vi "UHR-Fleezers Control (host) - 9.0.vi"() -> ()   [LabVIEW 2009]
uses:
  <vilib>/Utility/miscctls.llb/LVPoint32TypeDef.ctl
  <vilib>/Utility/miscctls.llb/LVMinMaxIncTypeDef.ctl
  <vilib>/userDefined/High Color/nirio_resource_hc.ctl
  <vilib>/Instr/_visa.llb/VISA Configure Serial Port (Instr).vi
  <vilib>/rvi/interface/nirviOpenFPGA/nirviOpenFPGA.xnode
  FPGA Bitfiles/UHR-Fleezers Instr~3C_FPGA Target_UHR-Fleezers Contr~F0.lvbitx
  UHR-Fleezers Control (fpga) - 9.1.vi
  <vilib>/FPGAPlugInAG/PCIe-7852R/nirviIntfOpen_PCIe-7852R.vi
  <vilib>/rvi/interface/nirviMethod/nirviMethod.xnode
  <vilib>/Utility/error.llb/Merge Errors.vi
  <vilib>/LabVIEW Targets/FPGA/Rio/nirio_HostInterface/nirio_Reset.vi
  <vilib>/LabVIEW Targets/FPGA/Rio/nirio_HostInterface/nirio_DMAStopAll.vi
  <vilib>/rvi/interface/common/niFpgaNodeNameForErrorReporting.ctl
  <vilib>/rvi/errors/niLvFpgaWhatHappensToTopLevelVI.ctl
  <vilib>/LabVIEW Targets/FPGA/Rio/nirio_HostInterface/nirio_DisableInterrupts.vi
  <vilib>/Utility/error.llb/Error Cluster From Error Code.vi
  <vilib>/rvi/errors/niLvFpgaAdjustHostInterfaceError.vi
  <vilib>/rvi/interface/nirviReadWriteControl/nirviReadWriteControl.xnode
  <vilib>/LabVIEW Targets/FPGA/Rio/nirio_HostInterface/nirio_WriteBig.vi
  <vilib>/LabVIEW Targets/FPGA/Rio/nirio_HostInterface/nirio_DMAConfigure.vi
  <vilib>/LabVIEW Targets/FPGA/Rio/nirio_HostInterface/nirio_DMAStop.vi
  <vilib>/RVI Host/nirviSupport.llb/nirviErrorClusterFromErrorCode.vi
  <vilib>/LabVIEW Targets/FPGA/Rio/nirio_HostInterface/nirio_EnableInterrupts.vi
  <vilib>/rvi/errors/niLvFpgaReportInternalErrorWithAdditionalInfo.vi
  <vilib>/Platform/TimedLoop/XDataNode/XDataNode.xnode
  <vilib>/Platform/TimedLoop/XDataNode/loadlvalarms.vi
  <vilib>/Platform/TimedLoop/XDataNode/timing_clust.ctl
  <vilib>/Platform/TimedLoop/XDataNode/nitl_modes.ctl
  <vilib>/Platform/TimedLoop/XDataNode/wakeup.ctl
  <vilib>/express/express analysis/Spectral/XNode/ExpressSpectralMeasurementsBlockNode.xnode
  <vilib>/express/express analysis/Spectral/Block/exnSpectralBlock spectral measurements PSD poly.vi
  <vilib>/express/express analysis/Spectral/Block/exnSpectralBlock spectral measurements PSD WFM.vi
  <vilib>/Waveform/WDTOps.llb/WDT Append Waveforms DBL.vi
  <vilib>/LabVIEW Targets/FPGA/Rio/nirio_HostInterface/nirio_ReadBig.vi
  <vilib>/vision/Avi1.llb/AviRefnum.ctl
  <vilib>/rvi/interface/nirviCloseFPGA/nirviCloseFPGA.xnode
  <vilib>/FPGAPlugInAG/PCIe-7852R/nirviIntfClose_PCIe-7852R.vi
  <vilib>/Analysis/NI_AALBase.lvlib
  <vilib>/Platform/TimedLoop/XDataNode/XDNodeRunTimeDep.lvlib
  openfpgaref.8.6.ctl
  NiRioSrv.dll
  <vilib>/vision/NI_Vision_Development_Module.lvlib
panel:
  in  "Set Confocal Spot":bool
  out "X (V)":dbl format="%_3g"
  out "Y (V)":dbl format="%_3g"
  in  "Tab Control 8":enum32{"APD 1 Image", "APD 1 Line Scan"}(tab)
  out "APD 1b":T1(plugin-control)
  out "Waveform Graph":dbl[](graph)
  in  "Total Volume\nFlushed (uL)":dbl
  in  "Flush Center Channel":bool
  in  "Inject Bottom Channel":bool
  in  "Inject Top Channel":bool
  out "Messages":string
  in  "APD Ave N":dbl=10.0
  out "Int. Time (s)":dbl
  in  "Stop All":bool
  out "sigma/mean":dbl
  out "Rate sigma (Hz)":dbl format="%0.2f"
  out "Current Stage  Position":cluster{dbl, dbl, dbl}
  in  "Index":dbl=1.0 caption="Save File Index" min=1.0 step=1.0
  in  "Tab Control 6":T2(tab)=enum."Dual Display (APD)"
  out "All Signals":waveform(dbl)[](graph)
  in  "Signals to Plot":i32(listbox)
  out "Trap Disp. Freq. (Hz)":dbl caption="Freq. (Hz)" format="%#_6p"
  out "Display Period (s)":dbl caption="Period (s)" format="%#_6p"
  in  "Trap Disp. Downsample":dbl=20000.0 caption="Downsample"
  in  "APD Disp. Scale":dbl=0.1 caption="Scale (Divide,\nfor above plot only)"
  in  "APD Disp. Downsample":dbl=30.0 caption="Integrate" min=1.0 step=1.0
  out "APD Display Freq. (Hz)":dbl caption="Freq. (Hz)"
  out "APD Display Period (s)":dbl caption="Period (s)"
  out "RMS (Ang)":dbl format="%_2g"
  in  "Bead Sep. Int. Time (s)":dbl=5.0 caption="Int. Time (s)"
  in  "Below (kHz)":dbl=0.5
  in  "Above (kHz)":dbl=2.0
  in  "Adjust Scale\nto Mean":bool
  in  "Rescale on Mean":bool
  in  "Offset (nm)":dbl
  out "Mean":dbl caption="Mean (pN)" format="%#_3g"
  out "Force":waveform(dbl)[](graph)
  out "APD 1 Chart":waveform(dbl)(graph)
  in  "Calibration":u16(ring)=2 items=["None", "Position", "Force"]
  out "T1 X":dbl caption="T1 X (pN)" format="%0.2f"
  out "T2 X":dbl caption="T2 X (pN)" format="%0.2f"
  out "Bead Separation":waveform(dbl)(graph)
  in  "Amplitude (nm)":dbl=1.0
  out "Bead Mean (nm)":dbl caption="Mean (nm)" format="%0.2f"
  out "Difference":dbl caption="Difference (pN)" format="%.2g"
  out "FFT 1":cluster{"f0":dbl, "df":dbl, "magnitude":dbl[]}[](graph)
  out "FFT 2":cluster{"f0":dbl, "df":dbl, "magnitude":dbl[]}[](graph)
  in  "FFT 1 Choice 1":u16(ring) items=["T1 Y", "T1 X", "T1 Sum", "T2 Y", "T2 X", "T2 Sum", "T1 FB X", "T1 FB Sum", "T2 FB X", "T2 FB Sum", "PSD Y", "PSD X", "PSD Y Sum", "none"]
  in  "FFT 2 Choice 1":u16(ring)=13 items=["T1 Y", "T1 X", "T1 Sum", "T2 Y", "T2 X", "T2 Sum", "T1 FB X", "T1 FB Sum", "T2 FB X", "T2 FB Sum", "PSD Y", "PSD X", "PSD Y Sum", "none"]
  in  "FFT 1 Choice 2":u16(ring)=1 items=["T1 Y", "T1 X", "T1 Sum", "T2 Y", "T2 X", "T2 Sum", "T1 FB X", "T1 FB Sum", "T2 FB X", "T2 FB Sum", "PSD Y", "PSD X", "PSD Y Sum", "none"]
  in  "FFT 2 Choice 2":u16(ring)=13 items=["T1 Y", "T1 X", "T1 Sum", "T2 Y", "T2 X", "T2 Sum", "T1 FB X", "T1 FB Sum", "T2 FB X", "T2 FB Sum", "PSD Y", "PSD X", "PSD Y Sum", "none"]
  in  "Compute FFT":bool
  in  "Reset FFT":bool
  in  "# Spectra to Ave.":dbl=100.0
  out "Ave. Time (s)":dbl
  out "1 Channel":waveform(dbl)(graph)
  out "Slow mean":dbl format="%0.2f"
  in  "Slow mean N ave.":dbl=1.0 min=1.0 step=1.0
  out "Mean Intensity":dbl
  out "Sigma":dbl
  out "Sigma/Mean":dbl
  in  "Subtract mean":bool
  in  "High Res. Display":u16(ring) items=["T1 Y", "T1 X", "T1 Sum", "T2 Y", "T2 X", "T2 Sum", "T1 FB X", "T1 FB Sum", "T2 FB X", "T2 FB Sum", "PSD Y", "PSD X", "PSD Y Sum"]
  out "APD 1 Rate (Hz)":dbl format="%#_3p"
  out "Image":u32[][](graph)
  in  "Tab Control":T3(tab)
  in  "Read Cal":bool
  out "Tether":bool
  in  "Tether Alarm?":bool=TRUE
  in  "Move to Delta (MHz)":dbl=15.6
  in  "Then...":string(combo)="2"
  in  "Data Acq. Spot":bool
  out "Fl. High":bool
  out "Waiting":bool
  in  "Yank to Freq. (MHz)":dbl
  in  "Fl. Threshold (kHz)":dbl
  in  "Fl. Triggered...":bool
  in  "Confocal Linescan":bool
  in  "Speed (nm/s)":dbl=100.0
  in  "Stop F (pN)":dbl=4.0
  in  "Furthest Withdraw (MHz)":dbl=15.0
  in  "Closest Delta (MHz)":dbl=10.0 step=0.25
  in  "Fish for Tether":bool
  in  "Confocal Image":bool
  in  "Round T1 X":bool caption="Round"
  in  "T1 offset_x (mV)":dbl=-26.302542012392074 format="%#_2g"
  in  "T1 kappa_x (pN/nm)":dbl=0.22546432407642192 min=0.0 step=0.001 format="%#_2g"
  out "Time (s)":dbl
  out "Total Time (s)":dbl
  in  "Start Saving":bool
  in  "Limits Enable":bool=TRUE caption="Enable"
  in  "Limit Max (MHz)":dbl=16.0 caption="Max (MHz)"
  in  "Limit Min (MHz)":dbl=10.0 caption="Min (MHz)"
  in  "Cal sets to save":u32=100 min=1 step=1
  in  "Comment (data description)":string="testing confocal setup"
  out "Calibrating Trap...":bool
  in  "Trap 2 (ON/OFF)":bool
  in  "Trap 1 (ON/OFF)":bool
  in  "Save Calibration":bool
  in  "N sets to save":u32=200 caption="N Sets"
  in  "Save N Sets":bool
  out "Save file name":path
  in  "Save ave N":dbl=500.0 caption="Averaging Factor"
  out "Saving...":bool
  in  "Stop Saving":bool
  out "Progress":u16(slide) scale=0.0..100.0
  out "Manipulating Trap":bool
  out "Buffer Status":dbl(slide) scale=0.0..1.0
  out "Overflow (data lost)":bool
  in  "Reset":bool
  out "Data Rate (Hz)":dbl caption="Trap Data Rate (Hz)" format="%#_3p"
  out "Data Period (s)":dbl caption="Trap Data Period (s)" format="%#_6p"
  out "Save Data Rate (Hz)":dbl caption="Rate (Hz)" format="%#_6p"
  out "Save Data Period (s)":dbl caption="Period (s)" format="%#_6p"
  in  "T1 alpha_x (nm/V)":dbl=630.439304367558 step=10.0 format="%#_3g"
  in  "T2 alpha_x (nm/V)":dbl=704.7738222964198 step=10.0 format="%#_3g"
  in  "T2 kappa_x (pN/nm)":dbl=0.2030110880477556 min=0.0 step=0.001 format="%#_2g"
  in  "T2 offset_x (mV)":dbl=-26.67973517613748 format="%#_2g"
  in  "BD 1 Frequency 1 (MHz)":dbl=69.4 caption="T1 X (MHz)" min=60.0 max=90.0 step=1.0 format="%#_6p"
  in  "BD 1 Frequency 2 (MHz)":dbl=85.0 caption="T2 X (MHz)" min=60.0 max=90.0 step=1.0 format="%#_6p"
  in  "Green Laser ON/Interlacing":bool
  in  "Round T2 X":bool caption="Round"
  in  "AO1":dbl(slide)=5.5955906765028605 caption="Confocal Y (V)" min=0.0 max=10.0 step=0.01 scale=0.0..10.0 scale format="%_1f"
  in  "AO2":dbl(slide)=5.59714185835527 caption="Confocal X (V)" min=0.0 max=10.0 step=0.01 scale=0.0..10.0 scale format="%_1f"
  in  "Upper Cap.":bool
  in  "Lower Cap.":bool
  in  "Trap Raster Scan":bool
  out "Raster Scanning...":bool
  in  "Trap Delta (MHz)":dbl=15.599999999999994
  in  "Action":string(combo)="Alarm"
  in  "Dump Beads":bool
  out "Duration (s)":dbl
  out "Stage Moving":bool
  in  "Wait Before Save (s)":u32=1
  out "Attempts":dbl
  in  "Attempt Limit":dbl=20.0 caption="Limit"
  in  "z nudge increment (um)":dbl=0.5
  in  "+z":bool
  in  "Saved Stage Positions":T4={"Position 1"={1.27817, -0.38076, 0.0}, "Position 2"={0.0, 0.0, 0.0}, "Position 3"={2.04843, -0.2477, 0.0}, "Position 4"={2.04843, 0.60288, 0.0}} {"Position 1"."?" min=-0.1 max=0.1 step=0.1; "Position 2"."?" min=-0.1 max=0.1 step=0.1; "Position 3"."?" min=-0.1 max=0.1 step=0.1; "Position 4"."?" min=-0.1 max=0.1 step=0.1}
  in  "Position 1 Label":string="Upper capillary"
  in  "Set Position 1":bool
  in  "Set Position 2":bool
  in  "Set Position 3":bool
  in  "Set Position 4":bool
  in  "Move to Position 3":bool
  in  "Move to Position 4":bool
  in  "Move to Position 2":bool
  in  "Move to Position 1":bool
  in  "Position 2 Label":string="Lower capillary"
  in  "Position 3 Label":string="Measurement Spot"
  in  "Position 4 Label":string="Dump beads"
  in  "-z":bool
  in  "Top Ch Inject Rate (ul/h)":dbl=10.0
  in  "Pump write delay (ms)":dbl=300.0
  in  "All Pump Parameters":T5={"Pump 1"={"Diameter (mm)"=4.61, "Units"=3.0, "Volume"=0.0, "Rate"=0.0}, "Pump 2"={"Diameter (mm)"=4.61, "Units"=3.0, "Volume"=0.0, "Rate"=0.0}, "Pump 3"={"Diameter (mm)"=4.61, "Units"=3.0, "Volume"=0.0, "Rate"=0.0}}
  in  "Top Ch Inject Volume (uL)":dbl=100.0
  in  "Pump pause delay (ms)":u32
  in  "Bottom Ch Inject Volume (uL)":dbl=100.0
  in  "Bottom Ch Inject Rate (ul/h)":dbl=10.0
  in  "Flush Center Ch Volume (uL)":dbl=15.0
  in  "Flush Center Ch Rate (ul/m)":dbl=100.0
  in  "Tab Control 2":T6(tab)=enum."AOD Raster Scan"
  out "Total Counts (ticks)":u32
  in  "Trap ON/OFF X or Y Amp?":bool=TRUE
  in  "Oscillate Set 1":bool
  in  "Trap 1 ON":bool
  in  "Number Interlace Sets":u8=3 min=1 max=3
  in  "DIO count 3 (ticks)":u32=200
  in  "DIO count 2 (ticks)":u32=200
  in  "DIO count 1 (ticks)":u32=200
  in  "BD 2 Amplitude 3 (%)":dbl min=0.0 max=50.0 step=1.0
  in  "BD 2 Amplitude 2 (%)":dbl min=0.0 max=50.0 step=1.0
  in  "BD 2 Amplitude 1 (%)":dbl min=0.0 max=50.0 step=1.0
  in  "BD 1 Amplitude 3 (%)":dbl min=0.0 max=50.0 step=1.0
  in  "BD 1 Amplitude 2 (%)":dbl=35.0 min=0.0 max=50.0 step=1.0
  in  "BD 1 Amplitude 1 (%)":dbl=10.0 min=0.0 max=50.0 step=1.0
  in  "BD 2 Frequency 3 (MHz)":dbl=26.0 min=0.0 max=40.0 step=1.0 format="%#_6p"
  in  "BD 1 Frequency 3 (MHz)":dbl=70.0 min=60.0 max=90.0 step=1.0 format="%#_6p"
  in  "BD 2 Frequency 2 (MHz)":dbl=26.0 min=0.0 max=40.0 step=1.0 format="%#_6p"
  in  "BD 2 Frequency 1 (MHz)":dbl=26.0 min=0.0 max=40.0 step=1.0 format="%#_6p"
  in  "Not-Interlacing Set":enum32{"Set 1", "Set 2", "Set 3"}(radio)
  in  "Interlace":bool=TRUE
  in  "Trap 2 ON":bool
  in  "Trap 3 ON":bool
  in  "Scan axis 2":bool=TRUE
  in  "Osc. freq. (Hz)":dbl=0.25
  in  "Osc. amp. (MHz)":dbl=2.0
  out "Coords":T7
  in  "Manipulation Scaling":cluster{"Horizontal":dbl, "Vertical":dbl}={"Horizontal"=0.075, "Vertical"=0.01}
  in  "Freq or Amp switch first":bool=TRUE
  in  "Swap F1 and F2":bool
  in  "Freq switch delay":u16
  in  "Amp switch delay":u16=5
  in  "MCL Step Increment (V_int)":dbl=3.0
  out "Time to Finish All (min)":dbl format="%#_2p"
  in  "Scan Speed (nm/s)":dbl=100.0
  in  "Scan Range (nm)":dbl=600.0
  in  "Step Size (nm)":dbl=1.0
  in  "MCL/AOM Scale Tweak":dbl=1.0
  in  "MCL Step Position Ratio":dbl=0.5
  in  "Move MCL Also?":bool=TRUE
  out "Final sep (nm)":dbl
  out "Initial sep (nm)":dbl
  out "Save index":dbl
  out "Final delta (MHz)":dbl
  out "Initial delta (MHz)":dbl
  out "Final freq. (MHz)":dbl
  out "Initial freq. (MHz)":dbl
  in  "Saved AOD Raster Scan Parameter Sets":T8(array[cluster])=[{"Scan Range AOD (nm) 2"=500.0, "Step Size AOD (nm) 2"=1.0, "Scan Speed AOD (nm/s) 2"=200.0, "Number of scans (AOD) 2"=1, "Label"=""}, {"Scan Range AOD (nm) 2"=1000.0, "Step Size AOD (nm) 2"=1.0, "Scan Speed AOD (nm/s) 2"=200.0, "Number of scans (AOD) 2"=5, "Label"="wide offset scan"}, {"Scan Range AOD (nm) 2"=20.0, "Step Size AOD (nm) 2"=0.68, "Scan Speed AOD (nm/s) 2"=0.68, "Number of scans (AOD) 2"=1, "Label"="2 bp steps"}]
  in  "Load parameters":bool
  out "Scan Range (MHz)":dbl=10.0
  in  "Restart DMA? (AOD)":bool=TRUE caption="Restart DMA?"
  out "Incr. int (AOD)":i64
  out "Time/Scan (s) (AOD)":dbl format="%#_2p"
  out "Data points/scans":dbl
  out "Data points/scan (f/b)":dbl
  in  "Save scans":bool=TRUE
  out "AOD Scan I":u64 caption="Scan I"
  in  "Continuous AOD Scanning":bool caption="Continuous Scanning"
  in  "Abort AOD Scan":bool caption="Abort Scan"
  in  "Scan BD":bool=TRUE
  out "Cycles/step (AOD)":u64=400 format="%.0p"
  in  "Number of F/B Scans (AOD)":u16=3 min=1
  out "Scan steps (AOD)":u64=1000
  out "Scan Increment (MHz)":dbl=0.2
  out "AOD Scanning":bool caption="Scanning"
  in  "Start AOD Scan":bool caption="Start Scan"
  out "N sets should be saved":dbl
  out "Progress 2":u16(slide) caption="Progress" scale=0.0..100.0
  in  "Abort save 2":bool caption="Abort save"
  in  "Trap 1 Bead Size (nm)":dbl=860.0
  in  "Trap 2 Bead Size (nm)":dbl=790.0
  out "MCL Count":dbl
  in  "All FB On/Off":bool=TRUE
  in  "AI2 to Setpoint":cluster{"Set 1":bool, "Set 2":bool}
  out "AI2 (V)":cluster{"Set 1":dbl, "Set 2":dbl}
  in  "Reset Feedback":cluster{"Set 1":bool, "Set 2":bool}
  in  "PID Gains":T9={"Set 1"={"proportional gain (Kc)"=0, "integral gain (Kc*Ts/Ti)"=5, "derivative gain (Kc*Td/Ts)"=0}, "Set 2"={"proportional gain (Kc)"=0, "integral gain (Kc*Ts/Ti)"=5, "derivative gain (Kc*Td/Ts)"=0}}
  in  "Setpoints (V)":cluster{"Set 1":dbl, "Set 2":dbl}={"Set 1"=7.0, "Set 2"=7.0}
  in  "Feedback On/Off":cluster{"Set 1":bool, "Set 2":bool}={"Set 1"=TRUE, "Set 2"=TRUE}
  in  "Tab Control 3":enum32{"Timing", "MCL Scan", "Analog Out"}(tab)
  out "APD Gate Late Counter":u32
  in  "- phase (APD Gate)":bool
  in  "+ phase (APD Gate)":bool
  out "APD Gate Relative Phase":i16
  in  "Phase Adj. (APD Gate)":i16=20
  in  "Initial Phase Adjustment (APD Gate)":i16=95
  in  "Save APD Data\nwith Trap Data":bool=TRUE
  out "APD FIFO Elements Remaining":u32
  in  "- phase (APD Acq)":bool
  in  "+ phase (APD Acq)":bool
  out "APD Acq Late Counter":u32
  out "APD Acq Relative Phase":i16
  in  "Phase Adj. (APD Acq)":i16=20
  in  "Initial Phase Adjustment (APD Acq)":i16
  in  "Invert APD Gate":bool caption="Invert Gate"
  in  "APD Gate OFF Count":u32=450 caption="Gate OFF Count"
  in  "APD Gate ON Count":u32=150 caption="Gate ON Count"
  in  "APD Gate":enum32{"ON", "OFF", "Interlace"}(radio)=enum."Interlace"
  in  "APD Integration Time (s)":dbl=0.01 caption="Integration Time (s)"
  out "APD Acq Rate (Hz)":dbl=20000000.0 caption="Rate (Hz)"
  out "APD Samples/FIFO Acq.":dbl
  out "APD Elements/DMA read":u32
  out "APD Int. Count":u32 format="%.0p"
  in  "Tab Control 5":enum32{"PSD X", "PSD Y", "Other Data Channel"}(tab)
  out "PSD X map":dbl[][](graph)
  out "PSD Y map":dbl[][](graph)
  out "Data map":dbl[][](graph)
  in  "Channel":i32=4
  in  "Abort MCL Scan":bool
  out "MCL Scan I":u64
  out "MCL Scanning":bool
  in  "Start MCL Scan":bool
  out "wait to reset values":bool
  in  "Tab Control 4":enum32{"Scan Settings", "MCL FPGA Loop Timing"}(tab)
  out "Total Time (s)":dbl
  in  "Scan lines (y)":u64=10
  in  "Fast Scan Dir":bool=TRUE
  in  "2D or 1D Scan":bool=TRUE
  out "Initial X":dbl
  out "Initial Y":dbl
  out "Time/f+b scan (s) (MCL)":dbl caption="Time/scan (s)"
  in  "Number of scans (MCL)":u64=1 caption="Scans"
  in  "Scan steps (MCL)":u64=20 caption="Scan steps (x)"
  in  "N APD Samp/step":dbl=6.0
  in  "Scan Range (V)\n(of steps)":dbl=3.0
  in  "Restart DMA? (MCL)":bool=TRUE caption="Restart DMA?"
  in  "Continuous MCL Scanning":bool caption="Cont. Scanning"
  in  "Center Scan":bool=TRUE
  in  "Save Data (MCL)":bool=TRUE caption="Save Data"
  out "Actual Incr. int (MCL)":i16 caption="Incr. int"
  out "Desired incr (int)":dbl
  out "Desired Scan Incr (V)":dbl
  out "N sets should be saved (MCL)":dbl caption="N sets should be saved"
  out "Data points/scans (MCL)":dbl caption="Data points/scans"
  out "Data points/scan (f+b)":dbl caption="points/scan (f+b)"
  out "Cycles/step (MCL)":u64 caption="Cycles/step" format="%.0p"
  out "Actual MCL Inc (V)":dbl
  in  "Phase adjust (MCL)":i16 caption="Phase adjust"
  out "Relative Phase (MCL)":i16 caption="Relative Phase"
  in  "Initial Phase Adj. (MCL)":i16 caption="Initial Phase Adj."
  in  "Update Count (MCL)":u32=800
  in  "+ phase (MCL)":bool
  in  "- phase (MCL)":bool
  out "MCL Late Counter":u32
  in  "APD 1 AO Mult.":i16=1 min=1
  in  "APD 2 AO Mult.":i16=1 min=1
  in  "APD 1 AO offset":i16
  in  "APD 2 AO offset":i16
  in  "Tab Control 7":enum32{"Green FB Signals", "Slow MCL Scan"}(tab)
  out "Green FB Plot":dbl(graph)
  out "MCL Scan 2":cluster{"Begin (V)":dbl, dbl, dbl[]}(graph)
  out "MCL Scan":cluster{"Begin (V)":dbl, dbl, dbl[]}(graph)
  in  "Green laser mode":enum32{"Laser ON", "Laser OFF", "Interlace"}(radio)=enum."Interlace"
  in  "GI Frequency, ON count":u32=150 min=1 step=1
  in  "Invert GI":bool
  out "GI Late Counter":u32
  in  "Phase adj. (GI)":i16=5
  out "GI relative phase":i16
  in  "+ phase (GI)":bool
  in  "Initial Phase Adjustment (GI)":i16=15
  in  "GI Frequency, OFF count":u32=450 min=1 step=1
  in  "- phase (GI)":bool
  out "Green FB Signals (V)":cluster{"Y":dbl, "X":dbl, "Sum":dbl}
  out "Relative phase (Green FB)":i16
  in  "+ phase (Green FB)":bool
  in  "- phase (Green FB)":bool
  in  "Green FB Count":u32=600
  in  "Phase adj. (Green FB)":i16=10
  in  "Initial Phase Adjustment (Green FB)":i16=50
  in  "Green FB On/Off":bool=TRUE
  in  "Current When FB OFF (%)":dbl=65.0 min=0.0 max=100.0 step=1.0
  in  "Green int current ON count adj":u32=150
  in  "Green FB Gains":T10={"proportional gain (Kc)"=10, "integral gain (Kc*Ts/Ti)"=5, "derivative gain (Kc*Td/Ts)"=0}
  in  "Green FB Setpoint (mV)":dbl=125.0
  in  "- phase (GI) 2":bool
  in  "Initial Phase Adjustment (GI) 2":i16=-100
  in  "+ phase (GI) 2":bool
  out "GI relative phase 2":i16
  in  "Phase adj. (GI) 2":i16=20
  out "GI Late Counter 2":u32
  in  "# Samples/trap":dbl=20000.0 format="%#_6p"
  out "Elements/DMA read":u32 format="%.0p"
  out "Ave. Rate (Hz)":dbl format="%#_6p"
  out "FIFO El. Rem.":u32 format="%.0p"
  in  "Phase adj. (AI1)":i16=15
  out "Relative phase (AI1)":i16
  in  "+ phase (AI1)":bool
  in  "- phase (AI1)":bool
  out "Late Counter (AI1)":u32
  in  "Initial Phase Adjustment (AI1)":i16=220
  out "AI rate (Hz)":dbl=50000.0 format="%#_6p"
  in  "AI Count (ticks)":u32=200
  out "# Samples/channel":u32=20000 format="%.0p"
  in  "FIFO Depth":u32=600000 format="%.0p"
  in  "Detector Type":string(combo)="IR-QPD + PSD + FB-QPD X position"
  in  "N Acq Sets (Traps)":i16=3
  in  "Sets to FIFO (Traps)":T11={"Set 1"=TRUE, "Set 2"=TRUE, "Set 3"=FALSE}
  in  "FPGA Ave.":dbl=1.0 min=1.0 step=1.0
  out "Ave. Period (s)":dbl format="%#_6p"
  out "DMA Update Period (s)":dbl
  out "FPGA Averaging":bool
  out "Trap Sets":i16
  out "Counts/DMA":dbl format="%#_6p"
  in  "Video Capture Rate (Hz)":dbl=30.0
  in  "Video Index":dbl=1.0 min=1.0 step=1.0
  in  "New Video File":bool
  in  "Capture Video":bool
  in  "Reset Averaging":bool
  in  "Averaging":bool
  in  "Capture and Save Image":bool
  in  "Image Index":dbl=1.0 min=1.0
  out "Path Out":path
  in  "Center Point":cluster{"X":i32, "Y":i32}
  in  "Zoom Factor":sgl=2.0
  out "Window Size":cluster{"Width":i32, "Height":i32}
  out "Window Position":cluster{"X Position":i32, "Y Position":i32}={"X Position"=40, "Y Position"=40}
  in  "Initial Window Size":cluster{"Width":i32, "Height":i32}={"Width"=884, "Height"=619}
  in  "Initial Window Position":cluster{"X Position":i32, "Y Position":i32}={"X Position"=796, "Y Position"=4}
  in  "Intensity Upper":u8=88
  in  "Intensity Lower":u8=66
  out "error out":errorcluster
  out "error out 2":errorcluster
  in  "Lost Tether Alarm Threshold (pN)":dbl=0.5
  in  "AOM X Cal (nm/MHz)":dbl=123.0
  in  "MCL X Cal (nm/V)":dbl=1070.0
  out "X RF Amplitude Limits (%)":T12={"Minimum"=0.0, "Maximum"=50.0, "Increment"=1.0}
  out "X RF Frequency Limits (MHz)":T12={"Minimum"=60.0, "Maximum"=90.0, "Increment"=1.0}
  out "Y RF Frequency Limits (MHz)":T12={"Minimum"=60.0, "Maximum"=90.0, "Increment"=1.0}
  out "Y RF Amplitude Limits (%)":T12={"Minimum"=0.0, "Maximum"=50.0, "Increment"=1.0}
  in  "Manip. X?":bool=TRUE
  in  "Manip. Y?":bool
  in  "Force Manip Abort":bool
  out "Read cal error":errorcluster
  in  "DAQ Delay (ms)":u32=1000
  in  "Start Scan":bool
  in  "Scan axis":bool=TRUE
  in  "Osc. amp. (V)":dbl=5.0
  in  "Osc. center (V)":dbl=5.0
  in  "Osc. freq. (Hz) 2":dbl=1.0
  in  "MCL Mode":u16(ring) items=["Manual Positioning", "Sinusoidal Wave", "Linear Scan"]
  in  "Begin (V)":dbl
  in  "End (V)":dbl=10.0
  in  "N Points":dbl=20.0
  in  "Delay to Interlace (s)":dbl
  in  "Delayed Interlace Start":bool
  in  "Read Lateness and Rel Phase":bool
  out "Vec Mean of T1 T2":dbl[](array[numeric])
  in  "Cal read wait (s)":u32=5
  out "Time tether formed":timestamp
  in  "Sample Chamber Stage Serial Port":refnum<visa-resource-name>="COM5"
  in  "Syringe Pump Serial Port":refnum<visa-resource-name>="COM4"
  # "Trap Display:"
  # "APD Display:"
  # "DAQ"
  # "Move Stage and Take Action"
  # "Trap Manipulation"
  # "Data Saving"
  # "Bead Calibration"
  # "Trap Position Difference Limits"
  # "Center channel"
  # "Units: \n1 = ml/m\n2 = ml/h\n3 = ul/m\n4 = ul/h"
  # "Rate param is ul/h\nVolume param is ul"
  # "X"
  # "Y"
  # "Oscillate Set 1 freq. (debugging)"
  # "BD 1"
  # "BD 2"
  # "AOD Raster Scan"
  # "Approx. trap separations"
  # "X"
  # "Y"
  # "Gate"
  # "X"
  # "2D"
  # "Y"
  # "1D"
  # "Green Laser Interlacing"
  # "Green FB Measurement"
  # "Digital Gate"
  # "Current Analog Control"
  # "Total AI Rates (NOT rates/trap)"
  # "(Samples/trap x Trap Sets)"
  # "(Samples/channel x\n8 if averaging (8 channels)\n4 if no averaging)"
  # "Trap 1"
  # "Trap 2"
  # "Flour./Trap 3"
  # "External Video Window"
  # "MCL Position Debugging"
  # "Temporary Control Storage\n(these used to be somewhere else, still want to keep them)"
  # "Y"
  # "X"
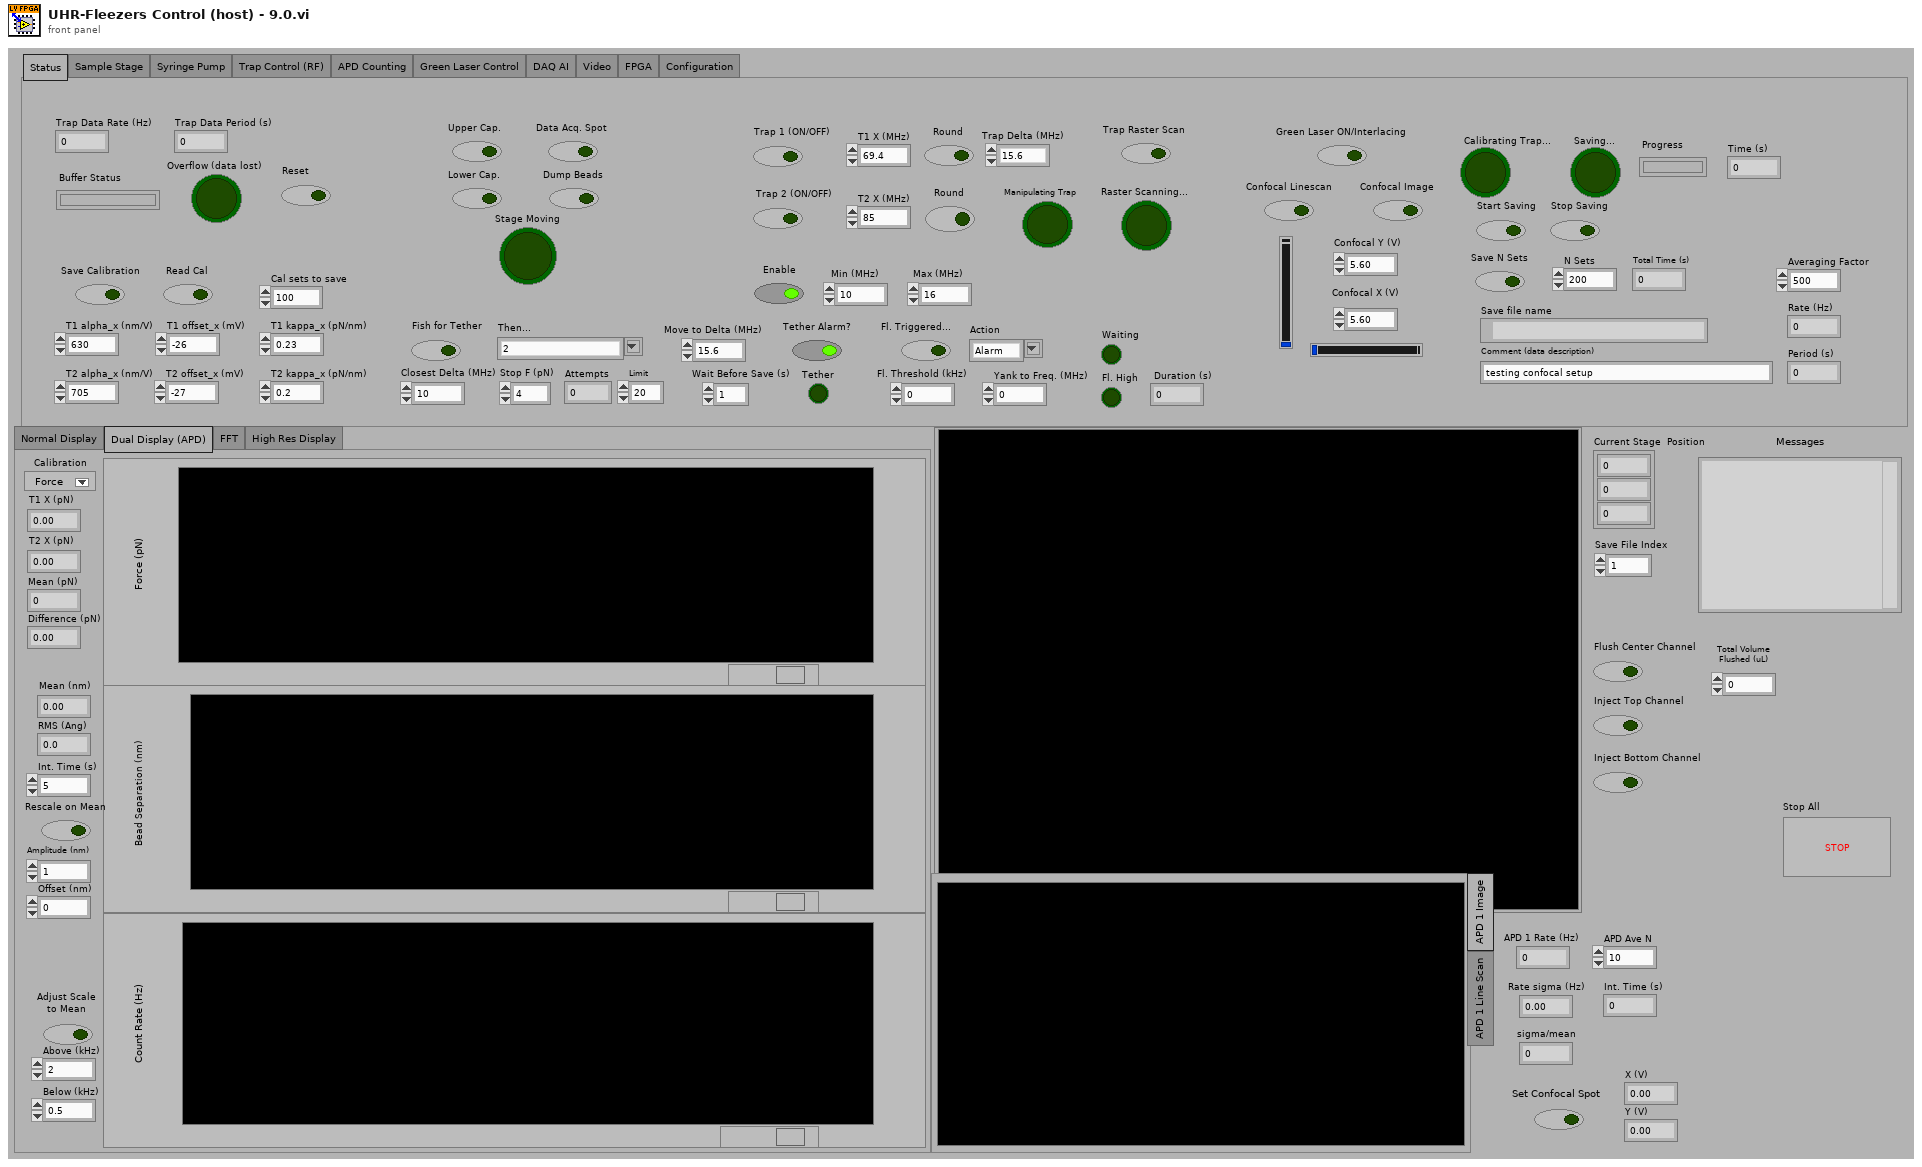
[diagram p1: front panel]
types:
  T1 = typedef "IMAQ Image.ctl" = refnum<image>
  T2 = enum32{"Normal Display", "Dual Display (APD)", "FFT", "High Res Display"}
  T3 = enum32{"Status", "Sample Stage", "Syringe Pump", "Trap Control (RF)", "APD Counting", "Green Laser Control", "DAQ AI", "Video", "FPGA", "Configuration"}
  T4 = cluster{"Position 1":cluster{dbl, dbl, dbl}, "Position 2":cluster{dbl, dbl, dbl}, "Position 3":cluster{dbl, dbl, dbl}, "Position 4":cluster{dbl, dbl, dbl}}
  T5 = cluster{"Pump 1":cluster{"Diameter (mm)":dbl, "Units":dbl, "Volume":dbl, "Rate":dbl}, "Pump 2":cluster{"Diameter (mm)":dbl, "Units":dbl, "Volume":dbl, "Rate":dbl}, "Pump 3":cluster{"Diameter (mm)":dbl, "Units":dbl, "Volume":dbl, "Rate":dbl}}
  T6 = enum32{"IR Laser Interlacing (Direct RF Board Control Method)", "AOD Raster Scan", "Feedback on BD 1 Amp to Control AI2"}
  T7 = typedef "LVPoint32TypeDef.ctl" = cluster{"Horizontal":i32, "Vertical":i32}
  T8 = cluster{"Scan Range AOD (nm) 2":dbl, "Step Size AOD (nm) 2":dbl, "Scan Speed AOD (nm/s) 2":dbl, "Number of scans (AOD) 2":u16, "Label":string}[]
  T9 = cluster{"Set 1":cluster{"proportional gain (Kc)":i16, "integral gain (Kc*Ts/Ti)":i16, "derivative gain (Kc*Td/Ts)":i16}, "Set 2":cluster{"proportional gain (Kc)":i16, "integral gain (Kc*Ts/Ti)":i16, "derivative gain (Kc*Td/Ts)":i16}}
  T10 = cluster{"proportional gain (Kc)":i16, "integral gain (Kc*Ts/Ti)":i16, "derivative gain (Kc*Td/Ts)":i16}
  T11 = cluster{"Set 1":bool, "Set 2":bool, "Set 3":bool}
  T12 = typedef "LVMinMaxIncTypeDef.ctl" = cluster{"Minimum":dbl, "Maximum":dbl, "Increment":dbl}
  T13 = typedef "Image Type" = u32
  T14 = typedef "nirio_resource_hc.ctl" = tag
  T15 = typedef "openfpgaref.8.6.ctl" = refnum<k20>
  T16 = typedef "niFpgaNodeNameForErrorReporting.ctl" = enum16{"Open FPGA VI Reference", "Read/Write Control", "Invoke Method: Abort", "Invoke Method: Acknowledge IRQ", "Invoke Method: Download", "Invoke Method: FIFO.Configure", "Invoke Method: FIFO.Read", "Invoke Method: FIFO.Start", "Invoke Method: FIFO.Stop", "Invoke Method: FIFO.Write", "Invoke Method: Reset", "Invoke Method: Run", "Invoke Method: Wait on IRQ", "Close FPGA VI Reference"}
  T17 = typedef "niLvFpgaWhatHappensToTopLevelVI.ctl" = enum16{"top level VI scripted behind XNode", "top level VI inlined behind XNode"}
  T18 = typedef "XDNodeRunTimeDep.lvlib/timing_clust.ctl" = cluster{"Expected End [f-1]":u64, "Actual End [f-1]":u64, "Finished Late? [f-1]":bool, "Expected End [i-1]":u64, "Actual End [i-1]":u64, "Finished Late? [i-1]":bool, "Expected Start [i]":u64, "Actual Start [i]":u64, "Expected Start [f]":u64, "Actual Start [f]":u64, "Source Name":string, "Structure Name":string, "Period":i64, "Deadline":i64, "Offset":i64, "Start":i64, "Priority":i32, "Timeout":i32, "Mode":T19, "Wakeup Reason":T20, "Error":errorcluster, "Source Type":string, "Secondary Source Type":string, "Global End Time":u64, "Global Start Time":u64, "Frame Duration":u64, "Iteration Duration":u64, "Assigned CPU":i32, "I/O Scan Engine Mode":u32}
  T19 = typedef "XDNodeRunTimeDep.lvlib/nitl_modes.ctl" = enum32{"No Change", "Process missed periods, maintain original phase", "Discard missed periods, maintain original phase", "Process missed periods, ignore original phase", "Discard missed periods, ignore original phase"}
  T20 = typedef "XDNodeRunTimeDep.lvlib/wakeup.ctl" = enum32{"Normal", "Aborted", "Asynchronous wakeup", "Timing source error", "Timed loop error", "Timeout"}
  T21 = enum32{"setting", "request", "request control", "info", "statistics", "system settings", "I/O sub system", "HRT control", "camera descriptions", "device specific data", "event sub system settings", "event sub system results", "image memory manager"}
  T22 = typedef "AviRefnum.ctl" = refnum<k1>
  T23 = typedef "imagedata.ctl" = cluster{"image type":i32, "image depth":i32, "image":u8[], "mask":u8[], "colors":u32[], "Rectangle":cluster{"left":i16, "top":i16, "right":i16, "bottom":i16}}
  T24 = cluster{"Origin Pixel":cluster{"X":sgl, "Y":sgl}, "Angle Relative to Horizontal (deg)":sgl, "Axis Reference":u32}
  T25 = typedef "Simple Grid Descriptor" = cluster{"X Step":sgl, "Y Step":sgl, "Unit":T26}
  T26 = typedef "Image Unit" = enum32{"Undefined", "Angström", "Micrometer", "Millimeter", "Centimeter", "Meter", "Kilometer", "Microinch", "Inch", "Feet", "Nautical miles", "Standard miles", "Steps"}
  T27 = cluster{"averaging mode":u16, "weighting mode":u16, "number of averages":u32}
  T28 = cluster{"dB On (F)":bool, "unwrap phase (F)":bool, "convert to degree (F)":bool}
  T29 = cluster{"Green FB Ch 0":i16, "Green FB Ch 1":i16, "Green FB Ch 2":i16}
  T30 = enum16{"open", "replace", "create", "open or create", "replace or create", "replace or create with confirmation"}
  T31 = enum16{"big-endian, network order", "native, host order", "little-endian"}
  T32 = cluster{string, string, string, string, string, string, string, string}
  T33 = cluster{string, string, string, string, string, string, string, string, string, string, string, string}
  T34 = cluster{string, string, string, string, string, string, string, string, string, string, string, string, string}
  T35 = cluster{string, string, string, string, string, string, string, string, string, string, string, string, string, string}
  T36 = cluster{"f0":dbl, "df":dbl, "magnitude":dbl[]}[][]
  T37 = cluster{"Green FB Ch 0":dbl, "Green FB Ch 1":dbl, "Green FB Ch 2":dbl}
  T38 = cluster{"Scan Range AOD (nm) 2":dbl, "Step Size AOD (nm) 2":dbl, "Scan Speed AOD (nm/s) 2":dbl, "Number of scans (AOD) 2":u16, "Label":string}
  T39 = cluster{"[0]":dbl, "[1]":dbl, "[2]":dbl, "[3]":dbl, "[4]":dbl, "[5]":dbl}
  T40 = cluster{"Diameter (mm)":dbl, "Units":dbl, "Volume":dbl, "Rate":dbl}
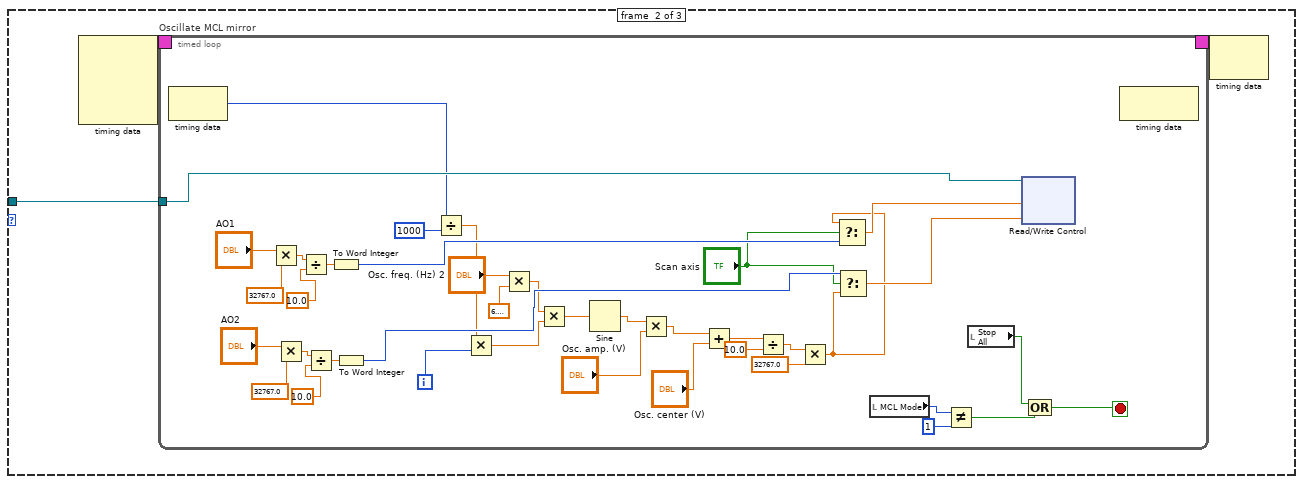
[diagram p2: hidden frame]
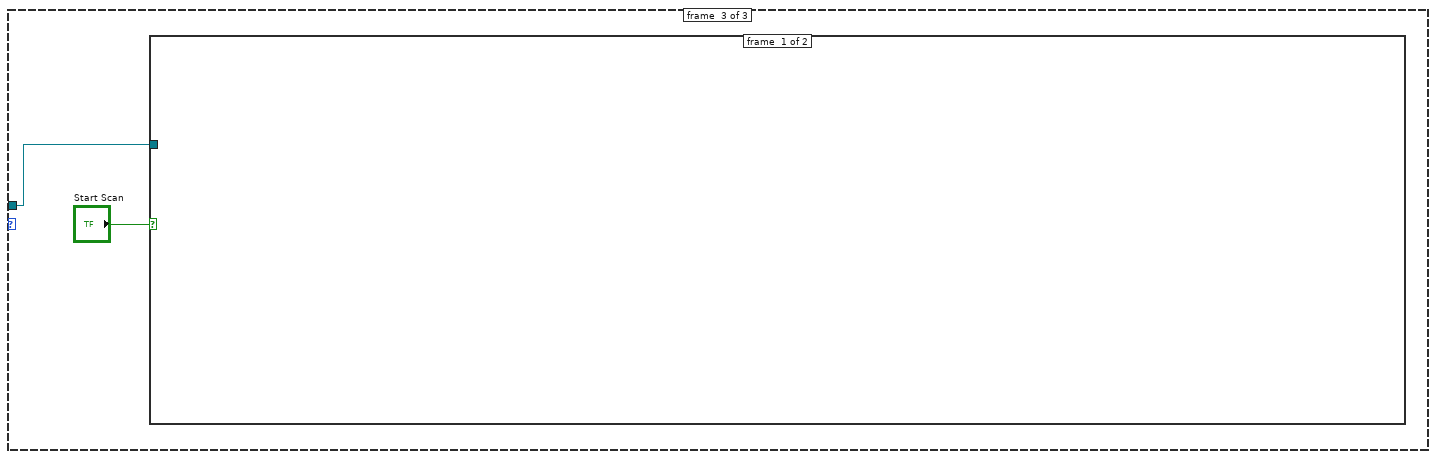
[diagram p3: hidden frame]
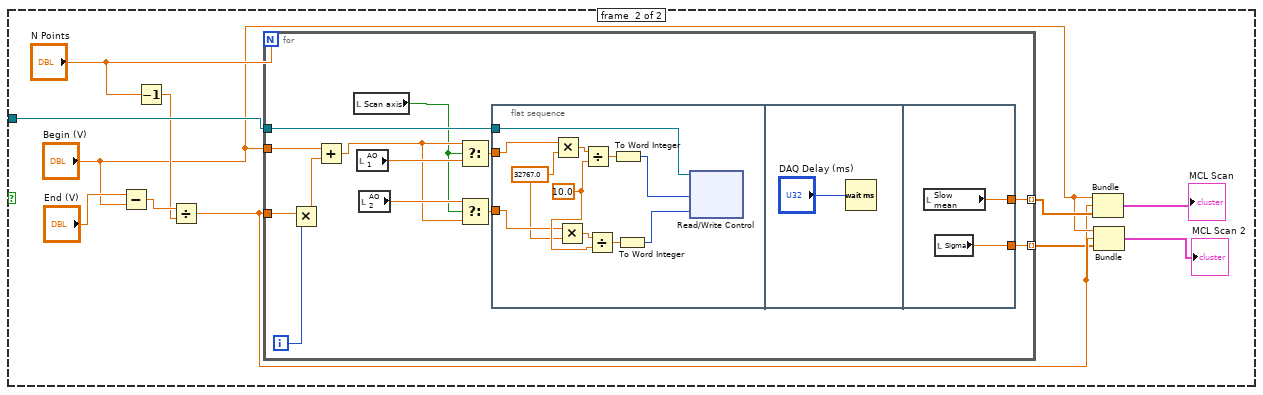
[diagram p4: hidden frame]
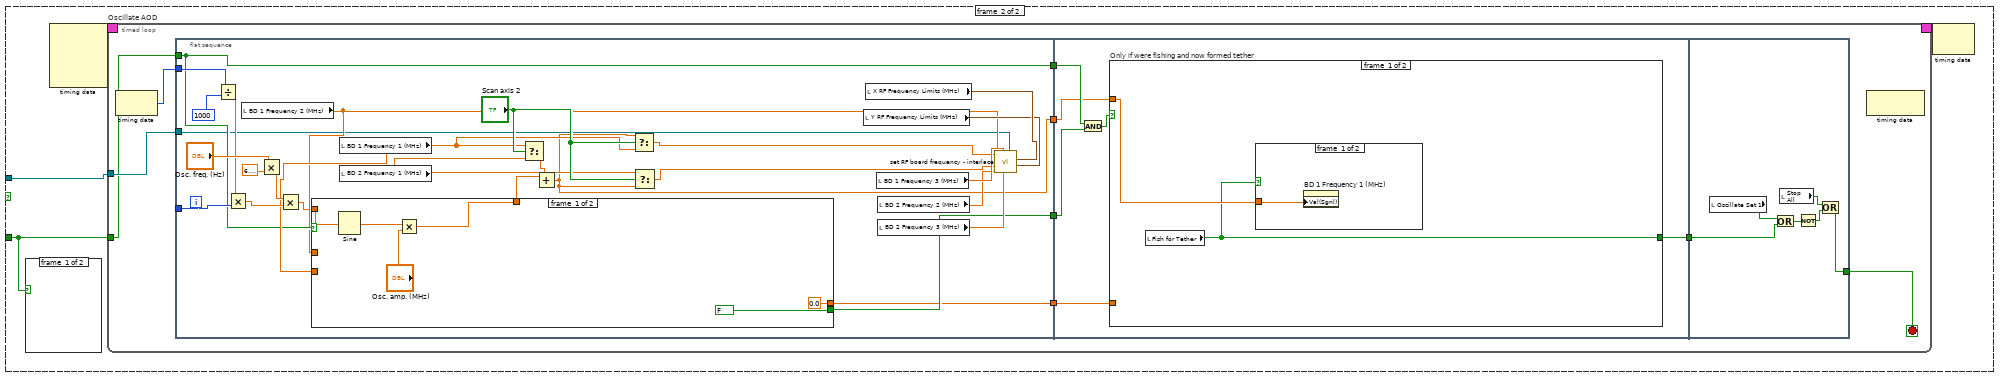
[diagram p5: hidden frame]
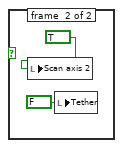
[diagram p6: hidden frame]
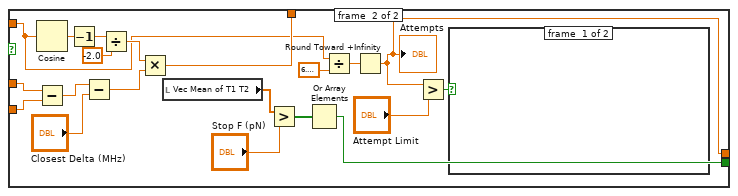
[diagram p7: hidden frame]
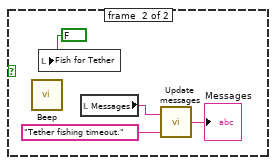
[diagram p8: hidden frame]
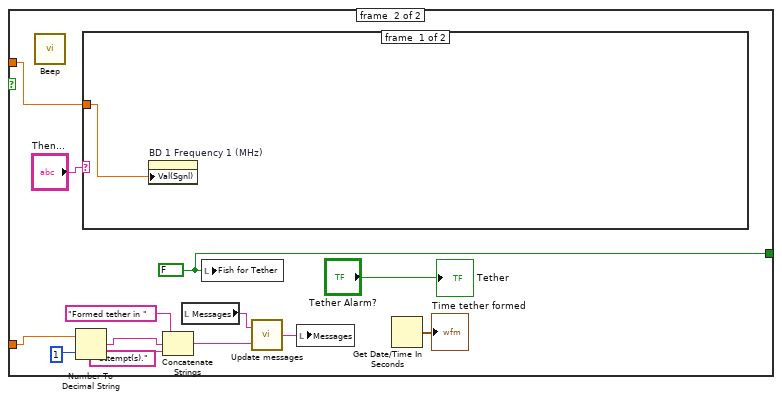
[diagram p10: hidden frame]
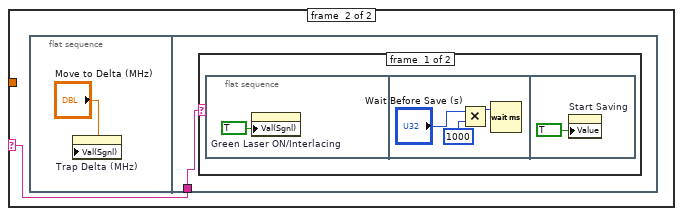
[diagram p11: hidden frame]
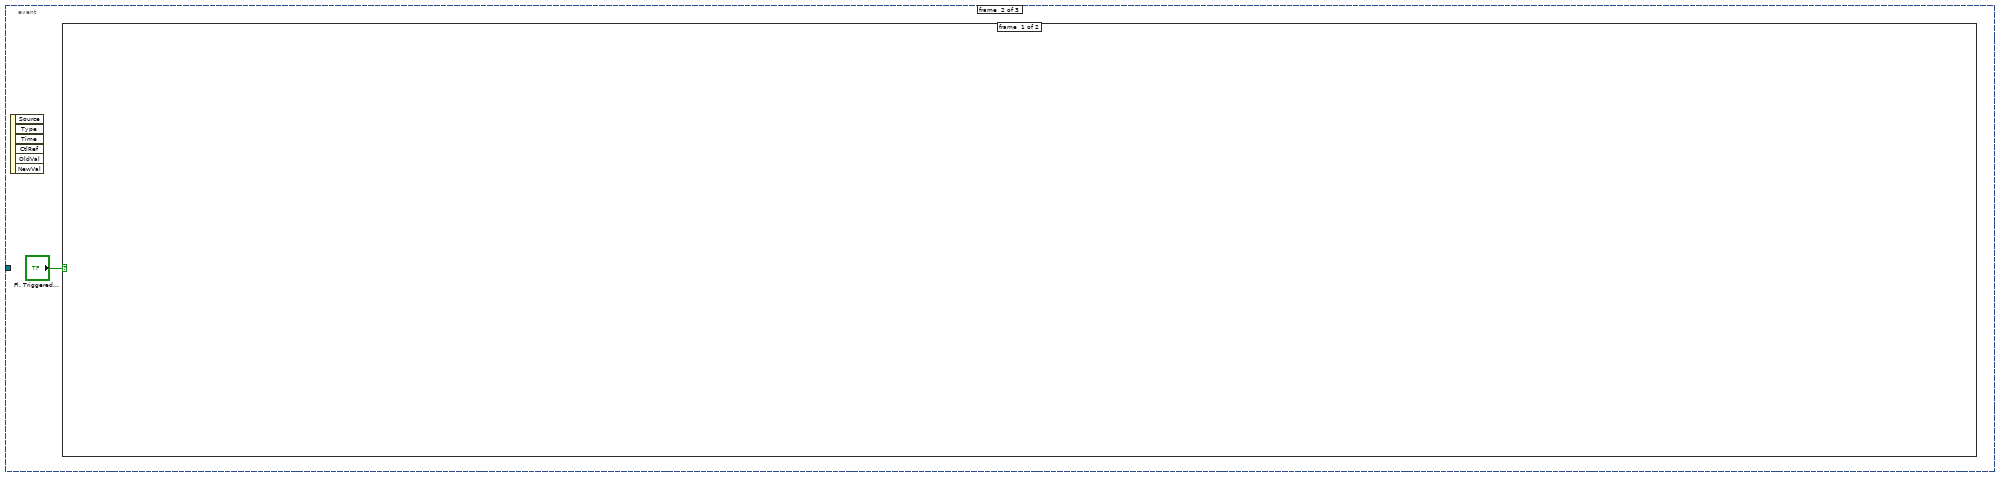
[diagram p13: hidden frame]
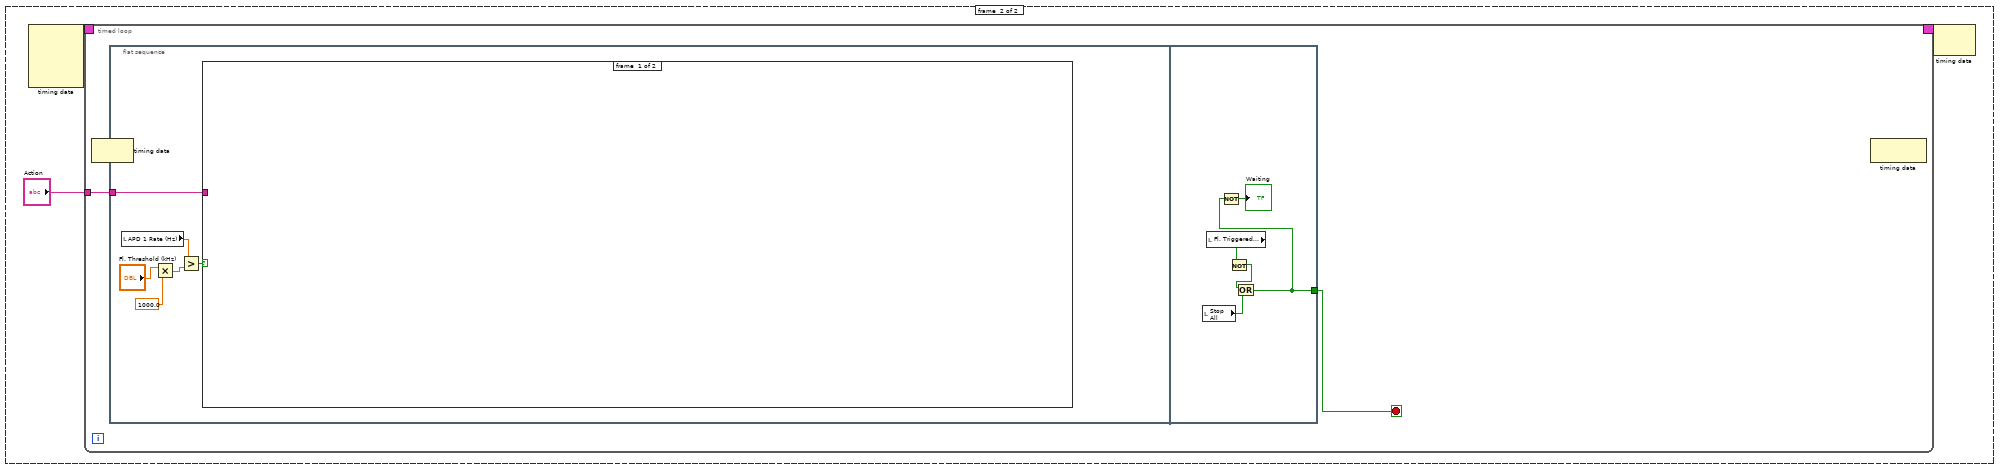
[diagram p14: hidden frame]
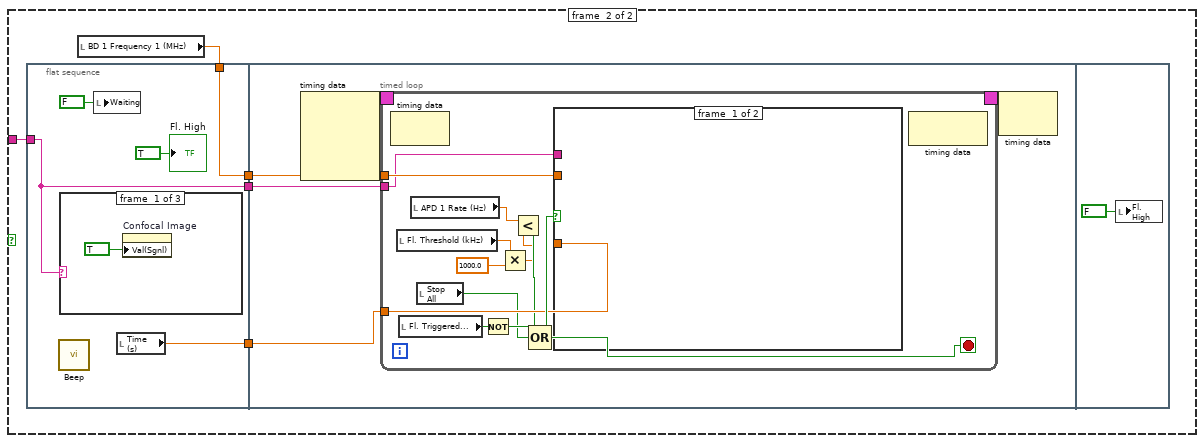
[diagram p15: hidden frame]
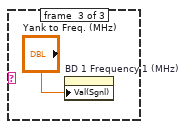
[diagram p17: hidden frame]
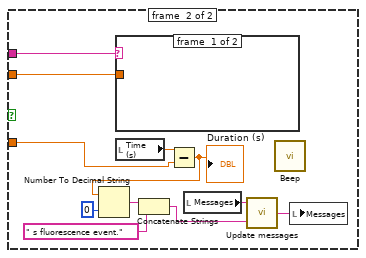
[diagram p18: hidden frame]
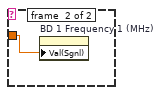
[diagram p19: hidden frame]
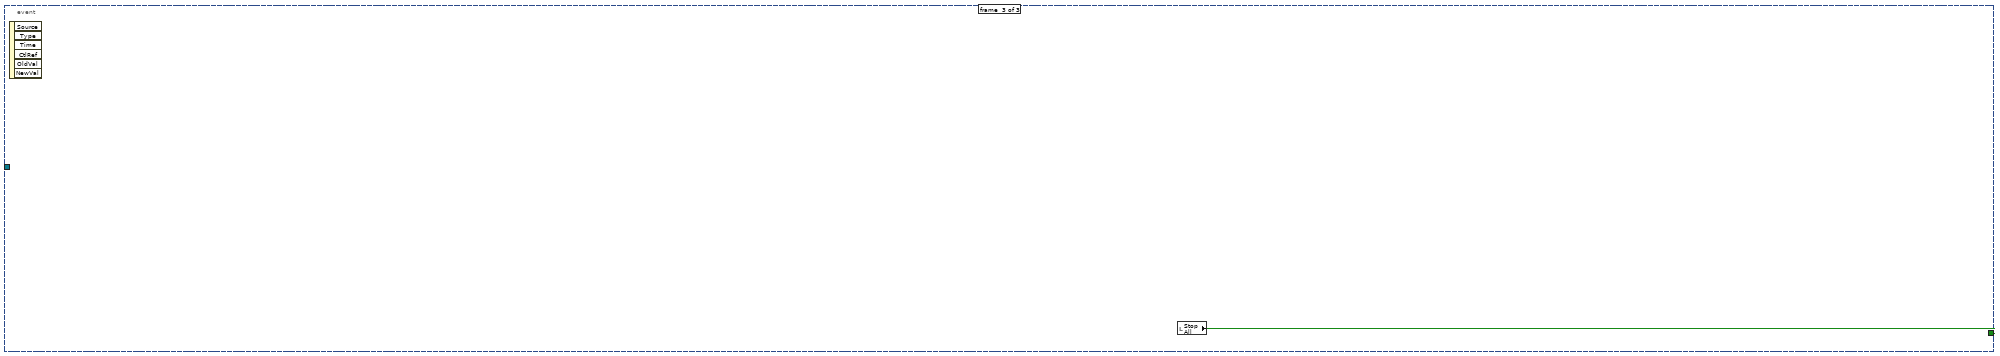
[diagram p20: hidden frame]
diagram:
  w2 = T13 2 items=["Grayscale (U8)", "Grayscale (I16)", "Grayscale (SGL)", "Complex (CSG)", "RGB (U32)", "HSL (U32)", "RGB (U64)", "Grayscale (U16)"] ("Image Type")
  w55 = T12 {"Minimum"=-0.1, "Maximum"=0.1, "Increment"=0.1}  # Z Limits
  w68 = cluster{"output high":i16, "output low":i16} {"output high"=3000, "output low"=0} ("FB output range 1")
  w74 = TRUE ("AI to FIFO")
  w159 = 10.0 ("y")
  w158 = 32767.0 ("y")
  w174 = 6.0  # clock mult.
  w175 = 49152000.0  # TCXO frequ.
  n1 = Build Array("DIO count 1 (ticks)", "DIO count 2 (ticks)", "DIO count 3 (ticks)") -> (w50:u32[])
  n2 = Multiply(x="APD Integration Time (s)", y=40000000.0) -> (x*y=w82:dbl)
  n3 = Reciprocal(x="APD Integration Time (s)") -> (1/x=w79:dbl)
  n4 = local write "APD Acq Rate (Hz)"(w79) -> ()
  n5 = local read "AO1"() -> (w153:dbl)
  n6 = local read "AO2"() -> (w152:dbl)
  n7 = To Unsigned Long Integer(number=w82) -> (unsigned 32bit integer=w81:u32)
  "APD Int. Count" <- w81
  n8 = local read "Scan Increment (MHz)"() -> (w170:dbl)
  n9 = local read "Fast Scan Dir"() -> (w139:bool)
  n10 = local read "Continuous MCL Scanning"() -> (w140:bool)
  n11 = Multiply(x=w153, y=w158) -> (x*y=w155:dbl)
  n12 = Multiply(x=w152, y=w158) -> (x*y=w157:dbl)
  n13 = local read "Number of scans (MCL)"() -> (w141:u64)
  n14 = Divide(x=w155, y=w159) -> (x/y=w154:dbl)
  n15 = Divide(x=w157, y=w159) -> (x/y=w156:dbl)
  n16 = To Word Integer(number=w154) -> (16bit integer=w151:i16)
  n17 = To Word Integer(number=w156) -> (16bit integer=w150:i16)
  n18 = Not(x=w139) -> (.not. x?=w134:bool)
  n19 = local read "Cycles/step (MCL)"() -> (w142:u64)
  n20 = Multiply(x=w170, y=1000.0) -> (x*y=w177:dbl)
  n21 = local read "Scan steps (MCL)"() -> (w143:u64)
  n22 = local read "Desired Scan Incr (V)"() -> (w145:dbl)
  n23 = Scale By Power Of 2(n=48, x=w177) -> (x*2^n=w178:dbl)
  n24 = Multiply(x=w175, y=w174) -> (x*y=w173:dbl)
  n25 = Divide(x=w178, y=w173) -> (x/y=w172:dbl)
  n26 = local read "Setpoints (V)"() -> (w198:cluster{"Set 1":dbl, "Set 2":dbl})
  n27 = property on="AI Count (ticks)" class="DigNum (strict)"("Val(Sgnl)"="AI Count (ticks)") -> ()  [unwired: 2 in, 2 out]
  n28 = local read "Number Interlace Sets"() -> (w43:u8)
  n29 = Split 1D Array(array=w50, index=w43) -> (first subarray=w52:u32[])  [unwired: 1 out]
  n30 = Add Array Elements(numeric array=w52) -> (sum=w51:u32)
  n31 = To Quad Integer(1:w172) -> (0:w169:i64)
  n32 = local read "Sets to FIFO (Traps)"() -> (w205:T11)
  n33 = local read "# Samples/channel"() -> (w162:u32)
  n34 = local read "Number of F/B Scans (AOD)"() -> (w163:u16)
  n35 = local read "Not-Interlacing Set"() -> (w42:enum32{"Set 1", "Set 2", "Set 3"})
  n36 = To Unsigned Byte Integer(number=w42) -> (unsigned 8bit integer=w48:u8)
  n37 = Index Array(array=w50, index=w48) -> (element=w49:u32)
  n38 = Divide(x=40000000.0, y="AI Count (ticks)") -> (x/y=w130:dbl)
  n39 = Multiply(x=w145, y=32767.0) -> (x*y=w147:dbl)
  n40 = local read "Feedback On/Off"() -> (w201:cluster{"Set 1":bool, "Set 2":bool})
  n41 = local read "PID Gains"() -> (w193:T9)
  n42 = local read "Scan steps (AOD)"() -> (w168:u64)
  n43 = local read "All FB On/Off"() -> (w202:bool)
  n44 = local write "AI rate (Hz)"(w130) -> ()
  n45 = local read "Cycles/step (AOD)"() -> (w167:u64)
  n46 = Divide(x=w147, y=10.0) -> (x/y=w146:dbl)
  n47 = Multiply(x=w168, y=w167) -> (x*y=w166:u64)
  n48 = Multiply(x=3276.7, y=w198) -> (x*y=w197:cluster{"Set 1":dbl, "Set 2":dbl})
  n49 = To Word Integer(number=w146) -> (16bit integer=w144:i16)
  n50 = Multiply(x=w166, y=u64 2) -> (x*y=w164:u64)
  n51 = Divide(x=w130, y="FPGA Ave.") -> (x/y=w131:dbl)
  n52 = To Word Integer(number=w197) -> (16bit integer=w196:cluster{"Set 1":i16, "Set 2":i16})
  n53 = xnode "Open FPGA VI Reference"("resource name"=T14 "750kHzDAQ") -> ("FPGA VI Reference Out"=w185:T15, "error out"=w184:errorcluster)  [unwired: 1 in]
  n54 = Unbundle By Name(w193) -> ("Set 1"=w192:T10, "Set 2"=w191:T10)
  n55 = Multiply(x=w164, y=w163) -> (x*y=w161:u64)
  n56 = Divide(x=w161, y=w162) -> (x/y=w160:dbl)
  n57 = Unbundle By Name(w196) -> ("Set 1"=w195:i16, "Set 2"=w194:i16)
  n58 = local write "Ave. Rate (Hz)"(w131) -> ()
  n59 = And(x=w201, y=w202) -> (x .and. y?=w200:cluster{"Set 1":bool, "Set 2":bool})
  n60 = local read "2D or 1D Scan"() -> (w71:bool)
  n61 = local write "Data points/scans"(w161) -> ()
  n62 = local read "Scan BD"() -> (w179:bool)
  n63 = Reciprocal(x=w131) -> (1/x=w132:dbl)
  n64 = local write "Data points/scan (f/b)"(w164) -> ()
  n65 = local write "N sets should be saved"(w160) -> ()
  n66 = local read "N Acq Sets (Traps)"() -> (w123:i16)
  n67 = Unbundle By Name(w200) -> ("Set 1"=w204:bool, "Set 2"=w203:bool)
  n68 = xnode "Invoke Method"("FPGA VI Reference In"=w185, "error in"=w184) -> ("FPGA VI Reference Out"=w67:T15, "error out"=w97:errorcluster)
  n69 = local read "Interlace"() -> (w44:bool)
  n70 = Select(t=w51, s=w44, f=w49) -> (s? t:f=w41:u32)
  n71 = local write "Update Count (MCL)"(w41) -> ()
  n72 = local write "Total Counts (ticks)"(w41) -> ()
  n73 = local write "Ave. Period (s)"(w132) -> ()
  n74 = property on="2D or 1D Scan" class="Bool (strict)"("Val(Sgnl)"=w71) -> ()  [unwired: 2 in, 2 out]
  n75 = xnode "Read/Write Control"("FPGA VI Reference In"=w66, "error in"=w97, "ai count"="AI Count (ticks)", "AI Averages"="FPGA Ave.", "DMA buffer timeout"=0, "AI to FIFO"=FALSE, "Interlace ON/OFF"=w44, "Number Interlace Cycles"=w43, "AI1 Sets to FIFO"=w205, "FB On/Off Set 1"=w204, "FB On/Off Set 2"=w203, "Interlace Off Parameters"=w42, "FB Setpoint Set 1"=w195, "FB Setpoint Set 2"=w194, "FB Gains Set 1"=w192, "FB Gains Set 2"=w191, "FB output range 1"=w68, "FB output range 2"=w68, "Cycles per step"=w167, "Scan BD"=w179, "Number of scans"=w163, "Scan steps"=w168, "Scan freq.  increment"=w169, "AO1"=w151, "AO2"=w150, "Scan freq.  increment (MCL)"=w144, "Scan steps (MCL)"=w143, "Cycles per step (MCL)"=w142, "Number of scans (MCL)"=w141, "MCL count"=w41, "Cont. Scan (MCL)"=w140, "MCL Scan Axis"=w134, "1D or 2D Scan?"=w71, "N of AI1 Int Acq Sets"=w123, "Freq or Amp switch first"="Freq or Amp switch first", "Freq switch delay"="Freq switch delay", "Amp switch delay"="Amp switch delay", "Swap F1 and F2"="Swap F1 and F2", "APD Acq Rate Count"=w81, "APD to FIFO"=FALSE, "APD Gate Operating Mode"="APD Gate", "APD Gate ON Count"="APD Gate ON Count", "APD Gate OFF Count"="APD Gate OFF Count", "Invert APD Gate"="Invert APD Gate", "DIO count 1 (ticks)"="DIO count 1 (ticks)", "DIO count 2 (ticks)"="DIO count 2 (ticks)", "DIO count 3 (ticks)"="DIO count 3 (ticks)", "APD 1 AO scale factor"="APD 1 AO Mult.", "APD 2 AO scale factor"="APD 2 AO Mult.", "APD 1 AO offset"="APD 1 AO offset", "APD 2 AO offset"="APD 2 AO offset") -> ("FPGA VI Reference Out"=w36:T15, "error out"=w38:errorcluster)
  n76 = local read "Green Laser ON/Interlacing"() -> (w39:bool)
  n77 = local read "GI Frequency, OFF count"() -> (w32:u32)
  n78 = Multiply(x="Current When FB OFF (%)", y=655.35) -> (x*y=w22:dbl)
  n79 = local read "GI Frequency, ON count"() -> (w31:u32)
  n80 = local read "Green laser mode"() -> (w40:enum32{"Laser ON", "Laser OFF", "Interlace"})
  n81 = local read "Green FB Count"() -> (w30:u32)
  n82 = To Unsigned Word Integer(number=w22) -> (unsigned 16bit integer=w20:u16)
  n83 = local read "Invert GI"() -> (w34:bool)
  n84 = Multiply(x="Green FB Setpoint (mV)", y=3.2767) -> (x*y=w19:dbl)
  n85 = case shown="False" w39 {
    tunnel: w40 -> [_ w232]
    tunnel: [enum32{"Laser ON", "Laser OFF", "Interlace"}."Laser OFF" ("Green laser mode") w232] -> w33
    frame #0 {
    }
    frame #1 {
    }
  }
  n86 = To Word Integer(number=w19) -> (16bit integer=w17:i16)
  n87 = xnode "Read/Write Control"("FPGA VI Reference In"=w36, "error in"=w38, "Green interlace ON count 2"=w31, "Green interlace OFF count 2"=w32, "Invert GI 2"=w34, "Operating Mode 2"=w33, "Green FB Gains"="Green FB Gains", "Green FB Setpoint"=w17, "Green FB On/Off"="Green FB On/Off", "Current Out"=w20, "Green int current ON count adj"="Green int current ON count adj", "Green FB Count"=w30, "Operating Mode"=w33, "Green interlace OFF count"=w32, "Green interlace ON count"=w31, "Invert GI"=w34) -> ("FPGA VI Reference Out"=w35:T15, "error out"=w37:errorcluster)
  n88 = flat-sequence {
    tunnel: w67 -> [w237]
    tunnel: [w237] -> w66
    tunnel: [w236] -> w65
    tunnel: [w235] -> w64
    tunnel: [w233] -> w62
    tunnel: [w234] -> w63
    frame #0 {
      w234 = T12 {"Minimum"=0.0, "Maximum"=40.0, "Increment"=1.0} ("Min Max Inc")
      w233 = T12 {"Minimum"=0.0, "Maximum"=50.0, "Increment"=1.0} ("Data Entry Limits")
      w236 = T12 {"Minimum"=60.0, "Maximum"=90.0, "Increment"=1.0} ("Min Max Inc")
      w235 = T12 {"Minimum"=0.0, "Maximum"=50.0, "Increment"=1.0} ("Data Entry Limits")
      n89 = property on="BD 2 Frequency 1 (MHz)" class="DigNum (strict)"("Data Range"=w234) -> ()  [unwired: 2 in, 2 out]
      n90 = property on="BD 2 Frequency 3 (MHz)" class="DigNum (strict)"("Data Range"=w234) -> ()  [unwired: 2 in, 2 out]
      n91 = property on="BD 2 Frequency 2 (MHz)" class="DigNum (strict)"("Data Range"=w234) -> ()  [unwired: 2 in, 2 out]
      n92 = property on="BD 1 Frequency 1 (MHz)" class="DigNum (strict)"("Data Range"=w236) -> ()  [unwired: 2 in, 2 out]
      n93 = property on="BD 1 Frequency 2 (MHz)" class="DigNum (strict)"("Data Range"=w236) -> ()  [unwired: 2 in, 2 out]
      n94 = property on="BD 1 Frequency 3 (MHz)" class="DigNum (strict)"("Data Range"=w236) -> ()  [unwired: 2 in, 2 out]
      n95 = property on="BD 2 Amplitude 1 (%)" class="DigNum (strict)"("Data Range"=w233) -> ()  [unwired: 2 in, 2 out]
      n96 = property on="BD 2 Amplitude 2 (%)" class="DigNum (strict)"("Data Range"=w233) -> ()  [unwired: 2 in, 2 out]
      n97 = property on="BD 2 Amplitude 3 (%)" class="DigNum (strict)"("Data Range"=w233) -> ()  [unwired: 2 in, 2 out]
      n98 = property on="BD 1 Amplitude 3 (%)" class="DigNum (strict)"("Data Range"=w235) -> ()  [unwired: 2 in, 2 out]
      n99 = property on="BD 1 Amplitude 2 (%)" class="DigNum (strict)"("Data Range"=w235) -> ()  [unwired: 2 in, 2 out]
      n100 = property on="BD 1 Amplitude 1 (%)" class="DigNum (strict)"("Data Range"=w235) -> ()  [unwired: 2 in, 2 out]
      "X RF Frequency Limits (MHz)" <- w236
      "X RF Amplitude Limits (%)" <- w235
      "Y RF Amplitude Limits (%)" <- w233
      "Y RF Frequency Limits (MHz)" <- w234
    }
  }
  n101 = xnode "Invoke Method"("FPGA VI Reference In"=w35, "error in"=w37, "Depth"="FIFO Depth") -> ("FPGA VI Reference Out"=w190:T15, "error out"=w189:errorcluster)
  n102 = xnode "Invoke Method"("FPGA VI Reference In"=w190, "error in"=w189) -> ("FPGA VI Reference Out"=w96:T15, "error out"=w95:errorcluster)
  n103 = xnode "Invoke Method"("FPGA VI Reference In"=w96, "error in"=w95) -> ("FPGA VI Reference Out"=w94:T15, "error out"=w93:errorcluster)  [unwired: 1 out]
  n104 = flat-sequence "Initial FPGA Loop Relative Phase Adjustment" {
    tunnel: "Initial Phase Adjustment (AI1)" -> [w247]
    tunnel: "Initial Phase Adjustment (GI)" -> [w246]
    tunnel: w94 -> [w245]
    tunnel: w93 -> [w244]
    tunnel: "Initial Phase Adj. (MCL)" -> [w243]
    tunnel: [w248] -> w105
    tunnel: [w242] -> w101
    tunnel: "Initial Phase Adjustment (APD Acq)" -> [w241]
    tunnel: "Initial Phase Adjustment (APD Gate)" -> [w240]
    tunnel: "Initial Phase Adjustment (Green FB)" -> [w239]
    tunnel: "Initial Phase Adjustment (GI) 2" -> [w238]
    tunnel: w105 -> [w400]
    tunnel: [w401] -> w102
    tunnel: w101 -> [w401]
    tunnel: [w400] -> w100
    tunnel: w102 -> [w404]
    tunnel: w100 -> [w403]
    tunnel: [w406] -> w99
    tunnel: [w405] -> w98
    tunnel: [w565] -> w103
    tunnel: [w566] -> w104
    tunnel: w99 -> [w566]
    tunnel: w98 -> [w565]
    frame #0 {
      n105 = xnode "Read/Write Control"("FPGA VI Reference In"=w245, "error in"=w244, "Phase count adjustment"=w247, "Phase count adjustment (GI)"=w246, "Phase count adjustment (MCL)"=w243, "Phase Count Adjustment (APD Acq)"=w241, "Phase count adjustment (APD Gate)"=w240, "Phase count adjustment (Green FB)"=w239, "Phase count adjustment (GI) 2"=w238) -> ("FPGA VI Reference Out"=w242:T15, "error out"=w248:errorcluster)
    }
    frame #1 {
      n106 = Wait (ms)(milliseconds to wait=u32 1000) -> ()  [unwired: 1 out]
    }
    frame #2 {
      w402 = TRUE
      n107 = xnode "Read/Write Control"("FPGA VI Reference In"=w404, "error in"=w403, "+ phase"=w402, "+ phase (GI)"=w402, "+ phase (MCL)"=w402, "+ phase (APD Acq)"=w402, "+ phase (APD Gate)"=w402, "+ phase (Green FB)"=w402, "+ phase (GI) 2"=w402) -> ("FPGA VI Reference Out"=w405:T15, "error out"=w406:errorcluster)
    }
    frame #3 {
      n108 = Wait (ms)(milliseconds to wait=u32 1000) -> ()  [unwired: 1 out]
    }
  }
  n109 = local read "Phase adj. (Green FB)"() -> (w53:i16)
  n110 = local read "Phase adj. (GI) 2"() -> (w23:i16)
  n111 = local read "Phase adj. (AI1)"() -> (w137:i16)
  n112 = local read "Phase adj. (GI)"() -> (w136:i16)
  n113 = local read "Phase adjust (MCL)"() -> (w135:i16)
  n114 = xnode "Read/Write Control"("FPGA VI Reference In"=w103, "error in"=w104, "Phase count adjustment"=w137, "Phase count adjustment (GI)"=w136, "Phase count adjustment (MCL)"=w135, "Phase Count Adjustment (APD Acq)"="Phase Adj. (APD Acq)", "Phase count adjustment (APD Gate)"="Phase Adj. (APD Gate)", "Phase count adjustment (Green FB)"=w53, "Phase count adjustment (GI) 2"=w23) -> ("FPGA VI Reference Out"=w4:T15, "error out"=w112:errorcluster)
  n115 = call "Initialize RF boards - interlace 3.vi"("error in"=w112, "FPGA VI Reference In"=w4) -> ("error out"=w110:errorcluster, "FPGA VI Reference Out"=w111:T15)
  n116 = call "set RF board frequency - interlace.vi"("Board 2 Frequency Limits"=w63, "Board 1 Frequency Limits"=w65, "error in"=w110, "FPGA VI Reference In"=w111, "Board 2 Frequency 3 (MHz)"="BD 2 Frequency 3 (MHz)", "Board 1 Frequency 3 (MHz)"="BD 1 Frequency 3 (MHz)", "Board 2 Frequency 2 (MHz)"="BD 2 Frequency 2 (MHz)", "Board 2 Frequency 1 (MHz)"="BD 2 Frequency 1 (MHz)", "Board 1 Frequency 2 (MHz)"="BD 1 Frequency 2 (MHz)", "Board 1 Frequency 1  (MHz)"="BD 1 Frequency 1 (MHz)") -> ("error out"=w221:errorcluster, "FPGA VI Reference Out"=w222:T15)
  n117 = call "set RF board amplitude - interlace.vi"("Board 2 Amplitude Limits"=w62, "Board 1 Amplitude Limits"=w64, "error in"=w221, "FPGA VI Reference In"=w222, "Board 2 Amplitude 3 (%)"="BD 2 Amplitude 3 (%)", "Board 1 Amplitude 3 (%)"="BD 1 Amplitude 3 (%)", "Board 2 Amplitude 2 (%)"="BD 2 Amplitude 2 (%)", "Board 2 Amplitude 1 (%)"="BD 2 Amplitude 1 (%)", "Board 1 Amplitude 2 (%)"="BD 1 Amplitude 2 (%)", "Board 1 Amplitude 1 (%)"="BD 1 Amplitude 1 (%)") -> ("error out"=w209:errorcluster, "FPGA VI Reference Out"=w210:T15)
  n118 = flat-sequence {
    tunnel: w210 -> [w575]
    tunnel: w209 -> [w574]
    tunnel: [w573] -> w214
    tunnel: [w572] -> w213
    tunnel: [w616] -> w212
    tunnel: w214 -> [w616]
    tunnel: [w615] -> w211
    tunnel: w213 -> [w615]
    tunnel: w212 -> [w624]
    tunnel: w211 -> [w623]
    tunnel: [w622] -> w76
    tunnel: [w621] -> w75
    frame #0 {
      n119 = local read "Trap 1 (ON/OFF)"() -> (w567:bool)
      n120 = xnode "Read/Write Control"("FPGA VI Reference In"=w575, "error in"=w574, "Direct RF Box  Communication"=FALSE) -> ("FPGA VI Reference Out"=w573:T15, "error out"=w572:errorcluster)
      n121 = local write "Saving..."(FALSE ("Saving Data")) -> ()
      n122 = local write "Stop All"(FALSE ("Stop All")) -> ()
      n123 = local write "Index"(1.0 ("Index")) -> ()
      n124 = property on="Trap 1 ON" class="Bool (strict)"("Value"=w567) -> ()  [unwired: 2 in, 2 out]
      "Manipulating Trap" <- FALSE ("Manipulating Trap")
    }
    frame #1 {
      n125 = local read "Trap 2 (ON/OFF)"() -> (w614:bool)
      n126 = Wait (ms)(milliseconds to wait=u32 10) -> ()  [unwired: 1 out]
      n127 = property on="Trap 2 ON" class="Bool (strict)"("Val(Sgnl)"=w614) -> ()  [unwired: 2 in, 2 out]
    }
    frame #2 {
      n128 = xnode "Read/Write Control"("FPGA VI Reference In"=w624, "error in"=w623, "FPGA Controls  RF Box"=TRUE ("Direct RF Box  Communication")) -> ("FPGA VI Reference Out"=w622:T15, "error out"=w621:errorcluster)
      n129 = call "Update messages.vi"("Message to add"="UHR-Fleezers ready.", "Old message string"="") -> ("New message string"=w620:string)
      n130 = local write "Messages"(w620) -> ()
    }
  }
  n131 = Subtract(x="BD 1 Frequency 1 (MHz)", y="BD 1 Frequency 2 (MHz)") -> (x-y=w122:dbl)
  n132 = Subtract(x="BD 2 Frequency 1 (MHz)", y="BD 2 Frequency 2 (MHz)") -> (x-y=w121:dbl)
  n133 = Square(x=w121) -> (x^2=w119:dbl)
  n134 = Square(x=w122) -> (x^2=w120:dbl)
  n135 = Add(x=w120, y=w119) -> (x+y=w118:dbl)
  n136 = Square Root(x=w118) -> (sqrt(x)=w117:dbl)
  n137 = local write "Trap Delta (MHz)"(w117) -> ()
  n138 = xnode "Read/Write Control"("FPGA VI Reference In"=w76, "error in"=w75, "AI to FIFO"=w74, "APD to FIFO"=w74) -> ("FPGA VI Reference Out"=w73:T15, "error out"=w72:errorcluster)
  n139 = property on="pos 1 z" class="DigNum (strict)"("Data Range"=w55) -> ()  [unwired: 2 in, 2 out]
  n140 = property on="pos 2 z" class="DigNum (strict)"("Data Range"=w55) -> ()  [unwired: 2 in, 2 out]
  n141 = property on="pos 3 z" class="DigNum (strict)"("Data Range"=w55) -> ()  [unwired: 2 in, 2 out]
  n142 = property on="pos 4 z" class="DigNum (strict)"("Data Range"=w55) -> ()  [unwired: 2 in, 2 out]
  n143 = node-c288(i64 1 ("Period")) -> (w126:T18)  [unwired: 3 out]
  n144 = node-c288() -> (w9:T18)  [unwired: 4 out]
  n145 = node-c288() -> (w11:T18)  [unwired: 4 out]
  n146 = node-c288() -> (w7:T18)  [unwired: 4 out]
  n147 = node-c288() -> (w15:T18)  [unwired: 4 out]
  n148 = node-c288() -> (w13:T18)  [unwired: 4 out]
  n149 = call-poly "VISA Configure Serial Port"("VISA resource name"="Sample Chamber Stage Serial Port") -> ("VISA resource name out"=w59:refnum<visa-resource-name>, "error out"=w58:errorcluster)  [unwired: 5 in, 8 out]
  n150 = call "IMAQ Create"("Image Name"="APD1 Image", "Image Type"=w2) -> ("New Image"=w1:T1)  [unwired: 3 in, 1 out]
  n151 = flat-sequence "Video" {
    tunnel: [w671] -> w188
    tunnel: w188 -> [w707]
    tunnel: w186 -> [w705]
    frame #0 {
      n152 = while {
        stop <- w664 continue-if-true
        n153 = call "Close Video Capture.vi"() -> ("error code OUT"=w666:i32)
        n154 = Equal?(x=w666, y=0) -> (x = y?=w664:bool)
      }
      n155 = local write "Stop All"(FALSE ("Stop All")) -> ()
    }
    frame #1 {
      n156 = call "DMR_Init.vi"() -> ()  [unwired: 3 out]
    }
    frame #2 {
      # "Setting the destination format to Mono8 makes sure that the image can be displayed in the intensity plot."
      n157 = call "DMR_GetDevice.vi"("search string IN"="DE019116701") -> ("device handle OUT"=w689:i32)  [unwired: 4 in, 2 out]
      n158 = call "DMR_OpenDevice.vi"("device handle IN"=w689) -> ("driver handle OUT"=w672:i32)  [unwired: 4 out]
      n159 = call "DMR_FindList.vi"("flags IN"=u32 0 ("flags"), "list name IN"="" ("String"), "list type IN"=T21."camera descriptions", "driver handle IN"=w672) -> ("list handle OUT"=w675:i32)  [unwired: 2 out]
      n160 = call "DMR_FindList.vi"("flags IN"=u32 0 ("flags"), "list name IN"="Base", "list type IN"=T21."setting", "driver handle IN"=w672) -> ("list handle OUT"=w673:i32)  [unwired: 2 out]
      n161 = call "OBJ_GetHandle.vi"("object name IN"="VideoStandard", "list handle IN"=w675) -> ("object handle OUT"=w669:i32)  [unwired: 3 out]
      n162 = call "OBJ_GetHandle.vi"("object name IN"="PixelFormat", "list handle IN"=w673) -> ("object handle OUT"=w683:i32)  [unwired: 3 out]
      n163 = call "OBJ_SetS.vi"("value index IN"=0, "value IN"="NTSC M", "object handle IN"=w669) -> ()  [unwired: 2 out]
      n164 = call "OBJ_SetS.vi"("value index IN"=0, "value IN"="Mono8" ("value"), "object handle IN"=w683) -> ()  [unwired: 2 out]
      n165 = call "OBJ_GetHandle.vi"("object name IN"="VideoChannel", "list handle IN"=w673) -> ("object handle OUT"=w679:i32)  [unwired: 3 out]
      n166 = while {
        tunnel: [w694] -> w671
        tunnel: w672 -> [w691]
        stop <- w692 continue-if-true
        n167 = call "DMR_ImageRequestSingle.vi"("request control IN"=0, "driver handle IN"=w691) -> ("error code OUT"=w693:i32, "driver handle OUT"=w694:i32)  [unwired: 2 out]
        n168 = Equal To 0?(x=w693) -> (x = 0?=w692:bool)
      }
      n169 = call "OBJ_SetI.vi"("value index IN"=0, "value IN"=3 ("Video channel"), "object handle IN"=w679) -> ()  [unwired: 2 out]
    }
    frame #3 {
      w702 = T13 0 items=["Grayscale (U8)", "Grayscale (I16)", "Grayscale (SGL)", "Complex (CSG)", "RGB (U32)", "HSL (U32)", "RGB (U64)"] ("Image Type")
      n170 = call "IMAQ Create"("Image Name"="untitled", "Image Type"=w702) -> ("New Image"=w703:T1)  [unwired: 2 in, 2 out]
      n171 = node-c288() -> (w701:T18)  [unwired: 4 out]
      n172 = Initialize Array(u32 0 ("Window Number (0...15)"), 480 ("dimension size"), 640 ("dimension size")) -> (w696:u32[][])
      n173 = timed-loop {
        tunnel: w707 -> [w725]
        tunnel: [w724] -> w706
        tunnel: w705 -> [w723]
        tunnel: w703 -> [w722]
        timing: w701 -> [_]
        timing-out: [_] -> w700
        tunnel: w696 -> [w708]
        stop <- w711 stop-if-true
        # "This block performs the \nactual image capture."
        n174 = node-c288() -> ()  [unwired: 2 out]
        n175 = local read "Stop All"() -> (w712:bool)
        n176 = Reciprocal(x="Video Capture Rate (Hz)") -> (1/x=w714:dbl)
        n177 = Or(x=FALSE, y=w712) -> (x .or. y?=w711:bool)
        n178 = Multiply(x=w714, y=1000.0) -> (x*y=w709:dbl)
        n179 = call "DMR_ImageRequestWaitFor.vi"("queue number IN"=0, "timeout(ms) IN"=500, "driver handle IN"=w725) -> ("error code OUT"=w729:i32, "request number OUT"=w726:i32, "driver handle OUT"=w727:i32)
        n180 = feedback #1(T22 refnum ("Avi Refnum")) -> (w716:T22)
        n181 = case shown="True" "New Video File" {
          tunnel: [T22 refnum ("Avi Refnum") w746] -> w718
          tunnel: [FALSE TRUE] -> w719
          tunnel: w716 -> [_ w742]
          frame #0 {
          }
          frame #1 {
            n182 = call "Create new save file.vi"("Ext"=".avi" ("string"), "Index In"="Video Index") -> ("Path Out"=w738:path, "Index Out"=w739:dbl)  [unwired: 1 in]
            "Path Out" <- w738
            n183 = Not Equal?(x=w742, y=T22 refnum ("Avi Refnum")) -> (x != y?=w743:bool)
            n184 = Increment(x=w739) -> (x+1=w748:dbl)
            n185 = case shown="True" w743 {
              tunnel: w742 -> [_ w749]
              frame #0 {
              }
              frame #1 {
                n186 = call "IMAQ AVI Close"("Avi Refnum"=w749) -> ()  [unwired: 1 in, 10 out]
              }
            }
            n187 = call "IMAQ AVI Create"("Frames Per Second"=u32 30, "AVI Path"=w738) -> ("Avi Refnum"=w746:T22)  [unwired: 5 in, 4 out]
            n188 = local write "Video Index"(w748) -> ()
          }
        }
        n189 = Equal To 0?(x=w729) -> (x = 0?=w728:bool)
        n190 = Select(t=w718, s=w719, f=w716) -> (s? t:f=w717:T22)
        n191 = case shown="True" w728 {
          tunnel: w727 -> [w750 w790]
          tunnel: w726 -> [_ w789]
          tunnel: [w750 w786] -> w724
          tunnel: w723 -> [_ w776]
          tunnel: w722 -> [_ w769]
          tunnel: w708 -> [_ w773]
          tunnel: w717 -> [_ w771]
          frame #0 {
          }
          frame #1 {
            w780 = u32 0 ("X-offset IN")
            n192 = call "DMR_GetImageRequestBufferData.vi"("driver handle IN"=w790, "request number IN"=w789) -> ("width OUT"=w779:i32, "height OUT"=w778:i32, "driver handle OUT"=w785:i32, "request number OUT"=w784:i32, "bytes per pixel OUT"=w781:i32)  [unwired: 13 out]
            n193 = call "DMR_GetImageRequestBufferImageData.vi"("driver handle IN"=w785, "request number IN"=w784, "bytes per pixel IN"=w781, "X-offset IN"=w780, "Y-offset IN"=w780, "height IN"=w778, "width IN"=w779) -> ("driver handle OUT"=w783:u32, "request number OUT"=w782:u32, "image OUT"=w774:u32[][])  [unwired: 10 out]
            n194 = call "DMR_ImageRequestUnlock.vi"("request number IN"=w782, "driver handle IN"=w783) -> ("driver handle OUT"=w788:i32)  [unwired: 1 in, 2 out]
            n195 = case shown="True" "Averaging" {
              tunnel: w774 -> [w816 w821]
              tunnel: [w816 w820] -> w770
              tunnel: w773 -> [_ w818]
              frame #0 {
              }
              frame #1 {
                (unwired) 1
                w826 = 1
                n196 = feedback #2(w818) -> (w817:u32[][])
                n197 = Add(x=w821, y=w817) -> (x+y=w822:u32[][])
                n198 = Select(t=w818, s="Reset Averaging", f=w822) -> (s? t:f=w824:u32[][])
                n199 = feedback #3(w826) -> (w819:i32)
                n200 = Divide(x=w822, y=w819) -> (x/y=w823:dbl[][])
                n201 = Increment(x=w819) -> (x+1=w827:i32)
                n202 = To Unsigned Long Integer(number=w823) -> (unsigned 32bit integer=w820:u32[][])
                n203 = Select(t=w826, s="Reset Averaging", f=w827) -> (s? t:f=w825:i32)
              }
            }
            "Image" <- w770
            n204 = case shown="True" "Capture and Save Image" {
              tunnel: w770 -> [_ w838]
              tunnel: w776 -> [_ w837]
              frame #0 {
              }
              frame #1 {
                n205 = To Unsigned Byte Integer(number=w838) -> (unsigned 8bit integer=w834:u8[][])
                n206 = call <vilib>:"Flatten Pixmap.vi"("colors"=w837, "8-bit pixmap"=w834) -> ("image data"=w835:T23)  [unwired: 4 in, 5 out]
                n207 = call "Create new save file.vi"("Insert"="video_frame_" ("string"), "Ext"=".bmp" ("string"), "Index In"="Image Index") -> ("Path Out"=w830:path, "Index Out"=w836:dbl)
                n208 = call <vilib>:"Write BMP File.vi"("image data"=w835, "path to BMP file"=w830) -> ()  [unwired: 1 in, 9 out]
                n209 = Increment(x=w836) -> (x+1=w829:dbl)
                n210 = local write "Image Index"(w829) -> ()
              }
            }
            n211 = case shown="True" "Capture Video" {
              tunnel: w771 -> [_ w815]
              tunnel: w770 -> [_ w813]
              tunnel: w769 -> [_ w812]
              frame #0 {
              }
              frame #1 {
                n212 = To Unsigned Byte Integer(number=w813) -> (unsigned 8bit integer=w814:u8[][])
                n213 = call "IMAQ ArrayToImage"("Image Pixels (U8)"=w814, "Image"=w812) -> ("Image Out"=w811:T1)  [unwired: 4 in, 5 out]
                n214 = call "IMAQ AVI Write Frame"("Image"=w811, "Avi Refnum"=w815) -> ()  [unwired: 2 in, 8 out]
              }
            }
            n215 = call "DMR_ImageRequestSingle.vi"("request control IN"=0, "driver handle IN"=w788) -> ("driver handle OUT"=w786:i32)  [unwired: 3 out]
            n216 = To Double Precision Float(number=w770) -> (double precision float=w763:dbl[][])
            n217 = Initialize Array(u8 1, 480 ("dimension size"), 640 ("dimension size")) -> (w762:u8[][])
            n218 = Multiply(x=w762, y="Intensity Upper") -> (x*y=w761:u8[][])
            n219 = Multiply(x=w762, y="Intensity Lower") -> (x*y=w760:u8[][])
            n220 = In Range and Coerce(upper limit=w761, x=w763, lower limit=w760) -> (coerced(x)=w759:dbl[][])  [unwired: 1 out]
            n221 = Subtract(x=w759, y="Intensity Lower") -> (x-y=w755:dbl[][])
            n222 = Subtract(x="Intensity Upper", y="Intensity Lower") -> (x-y=w754:u8)
            n223 = Divide(x=w755, y=w754) -> (x/y=w756:dbl[][])
            n224 = Multiply(x=u8 255, y=w756) -> (x*y=w752:dbl[][])
            n225 = To Unsigned Byte Integer(number=w752) -> (unsigned 8bit integer=w751:u8[][])
            n226 = call "IMAQ ArrayToImage"("Image Pixels (U8)"=w751, "Image"=w769) -> ("Image Out"=w767:T1)  [unwired: 4 in, 5 out]
            n227 = First Call?() -> (First Call?: T/F=w768:bool)
            n228 = case shown="False" w768 {
              tunnel: w767 -> [w791 w802]
              frame #0 {
                n229 = flat-sequence {
                  tunnel: w791 -> [w797]
                  frame #0 {
                    w794 = FALSE ("Get/Set Status? (Set)")
                    w793 = 0 ("Window Number (0...15)")
                    n230 = call "IMAQ WindSize"("Get/Set Status? (Set)"=w794, "Window Number"=w793) -> ("Width & Height out"=→"Window Size":cluster{"Width":i32, "Height":i32})  [unwired: 4 in, 2 out]
                    n231 = call "IMAQ WindMove"("Window Number (0...15)"=w793, "Get/Set Status? (Set)"=w794) -> ("Coordinates (screen)"=→"Window Position":cluster{"X Position":i32, "Y Position":i32})  [unwired: 3 in, 1 out]
                    n232 = call "IMAQ WindDraw"("Resize to Image Size? (Y)"=FALSE, "Window Number (0...15)"=w793, "Image"=w797) -> ()  [unwired: 7 in, 2 out]
                  }
                  frame #1 {
                    n233 = call "IMAQ WindZoom 2"("Center Point"="Center Point", "Zoom to Fit? (False)"=FALSE, "Zoom Factor"="Zoom Factor") -> ()  [unwired: 5 in, 4 out]
                  }
                }
              }
              frame #1 {
                n234 = flat-sequence {
                  tunnel: w802 -> [w805]
                  tunnel: [w803] -> w801
                  tunnel: w801 -> [w807]
                  frame #0 {
                    w804 = TRUE ("Resize to Image Size? (Y)")
                    w803 = 0 ("Window Number (0...15)")
                    n235 = call "IMAQ WindNonTearing"("Window Number"=w803, "NonTearing? (True)"=w804) -> ()  [unwired: 8 in, 2 out]
                    n236 = call "IMAQ WindDraw"("Resize to Image Size? (Y)"=w804, "Window Number (0...15)"=w803, "Image"=w805) -> ()  [unwired: 7 in, 2 out]
                  }
                  frame #1 {
                    n237 = call "IMAQ WindToolsSetup"() -> ("error out"=w810:errorcluster)  [unwired: 6 in]
                    n238 = call "IMAQ WindSize"("Scrollbars? (N)"=FALSE, "Width & Height"="Initial Window Size", "Window Number"=w807) -> ()  [unwired: 3 in, 3 out]
                    n239 = call "IMAQ WindToolsShow"("error in (no error)"=w810) -> ()  [unwired: 4 in, 2 out]
                    n240 = call "IMAQ WindMove"("Window Number (0...15)"=w807, "Coordinates (screen)"="Initial Window Position") -> ()  [unwired: 3 in, 2 out]
                  }
                }
              }
            }
          }
        }
        n241 = node-c288(w709) -> ()  [unwired: 1 out]
      }
      n242 = node-c288(w700) -> ()  [unwired: 1 out]
      n243 = call "DMR_CloseDevice.vi"("driver handle IN"=w706) -> ()  [unwired: 1 in, 4 out]
    }
    frame #4 {
      n244 = call "DMR_Close.vi"() -> ()  [unwired: 1 out]
    }
  }
  n245 = timed-loop "Acquire Data" {
    tunnel: w73 -> [w1013]
    tunnel: w72 -> [w1012]
    tunnel: [w1050] -> w229
    tunnel: [w1044] -> w227
    timing: w126 -> [_]
    timing-out: [_] -> w125
    tunnel: w1 -> [w842]
    stop <- "Stop All" stop-if-true
    w893 = "NI_ChannelName" ("name")
    n246 = node-c288() -> ()  [unwired: 2 out]
    n247 = case "Reset data stream" shown="True" "Reset" {
      tunnel: w1013 -> [w3229 w3236]
      tunnel: w1012 -> [w3228 w3235]
      tunnel: [w3229 w3231] -> w1008
      tunnel: [w3228 w3230] -> w1007
      frame #0 {
      }
      frame #1 {
        w3234 = TRUE ("AI to FIFO")
        w3241 = FALSE ("AI to FIFO")
        n248 = local write "Overflow (data lost)"(FALSE ("Overflow (data lost)")) -> ()
        n249 = xnode "Read/Write Control"("FPGA VI Reference In"=w3236, "error in"=w3235, "AI to FIFO"=w3241, "APD to FIFO"=w3241) -> ("FPGA VI Reference Out"=w3239:T15, "error out"=w3240:errorcluster)
        n250 = xnode "Invoke Method"("FPGA VI Reference In"=w3239, "error in"=w3240) -> ("FPGA VI Reference Out"=w3237:T15, "error out"=w3238:errorcluster)
        n251 = xnode "Invoke Method"("FPGA VI Reference In"=w3237, "error in"=w3238) -> ("FPGA VI Reference Out"=w3233:T15, "error out"=w3232:errorcluster)
        n252 = xnode "Read/Write Control"("FPGA VI Reference In"=w3233, "error in"=w3232, "AI to FIFO"=w3234, "APD to FIFO"=w3234) -> ("FPGA VI Reference Out"=w3231:T15, "error out"=w3230:errorcluster)
      }
    }
    n253 = Or(x="Start AOD Scan", y="Trap Raster Scan") -> (x .or. y?=w955:bool)
    n254 = And(x="Save scans", y=w955) -> (x .and. y?=w1004:bool)
    n255 = case "Start AOM raster scan" shown="True" w955 {
      tunnel: w1008 -> [w2468 w2477]
      tunnel: w1007 -> [w2467 w2476]
      tunnel: [w2468 w2470] -> w1006
      tunnel: [w2467 w2469] -> w1005
      frame #0 {
      }
      frame #1 {
        n256 = case shown="True" "Restart DMA? (AOD)" {
          tunnel: [w2843 w2844] -> w2471
          tunnel: [w2842 w2845] -> w2472
          tunnel: w2477 -> [w2843 w2851]
          tunnel: w2476 -> [w2842 w2850]
          frame #0 {
          }
          frame #1 {
            w2847 = FALSE ("AI to FIFO")
            n257 = xnode "Read/Write Control"("FPGA VI Reference In"=w2851, "error in"=w2850, "AI to FIFO"=w2847, "APD to FIFO"=w2847) -> ("FPGA VI Reference Out"=w2849:T15, "error out"=w2848:errorcluster)
            n258 = xnode "Invoke Method"("FPGA VI Reference In"=w2849, "error in"=w2848) -> ("FPGA VI Reference Out"=w2853:T15, "error out"=w2852:errorcluster)
            n259 = xnode "Invoke Method"("FPGA VI Reference In"=w2853, "error in"=w2852) -> ("FPGA VI Reference Out"=w2844:T15, "error out"=w2845:errorcluster)
            n260 = local write "Overflow (data lost)"(FALSE ("Overflow (data lost)")) -> ()
          }
        }
        n261 = case shown="True" "Move MCL Also?" {
          tunnel: w2472 -> [w2480 w2586]
          tunnel: w2471 -> [w2481 w2587]
          tunnel: [w2479 w2590] -> w2470
          tunnel: [w2478 w2589] -> w2469
          frame #0 {
            w2482 = TRUE ("AI to FIFO")
            n262 = xnode "Read/Write Control"("FPGA VI Reference In"=w2481, "error in"=w2480, "AI to FIFO"=w2482, "APD to FIFO"=w2482, "Start scan"=w2482) -> ("FPGA VI Reference Out"=w2479:T15, "error out"=w2478:errorcluster)
          }
          frame #1 {
            w2583 = FALSE ("1D or 2D Scan?")
            w2588 = TRUE ("AI to FIFO")
            # "Count for MCL loop"
            # "N total cycles"
            # "N steps"
            # "V_int"
            n263 = local read "Scan Range (nm)"() -> (w2565:dbl)
            n264 = local read "Number of F/B Scans (AOD)"() -> (w2582:u16)
            n265 = Sign(1:w2565) -> (0:w2564:dbl)
            n266 = Compound Arithmetic op=MULTIPLY(w2565, "MCL Step Position Ratio", "MCL/AOM Scale Tweak") -> (w2569:dbl)
            n267 = Negate(x=w2564) -> (-x=w2561:dbl)
            n268 = Multiply(x=w2561, y="MCL Step Increment (V_int)") -> (x*y=w2563:dbl)
            n269 = Divide(x=w2569, y="MCL X Cal (nm/V)") -> (x/y=w2575:dbl)
            n270 = Multiply(x=32767.0 ("y"), y=w2575) -> (x*y=w2581:dbl)
            n271 = local read "Total Counts (ticks)"() -> (w2566:u32)
            n272 = local read "Cycles/step (AOD)"() -> (w2577:u64)
            n273 = local read "Scan steps (AOD)"() -> (w2578:u64)
            n274 = Divide(x=w2581, y=10.0) -> (x/y=w2574:dbl)
            n275 = Divide(x=w2574, y="MCL Step Increment (V_int)") -> (x/y=w2572:dbl)
            n276 = Absolute Value(x=w2572) -> (abs(x)=w2560:dbl)
            n277 = Compound Arithmetic op=MULTIPLY(w2578, w2577, w2566) -> (w2573:u64)
            n278 = local write "wait to reset values"(w2588) -> ()
            n279 = local write "MCL Scanning"(w2588) -> ()
            n280 = Divide(x=w2573, y=w2560) -> (x/y=w2570:dbl)
            "MCL Count" <- w2570
            n281 = xnode "Read/Write Control"("FPGA VI Reference In"=w2587, "error in"=w2586, "Scan steps (MCL)"=w2560, "Number of scans (MCL)"=w2582, "Cycles per step (MCL)"=u64 1, "Scan freq.  increment (MCL)"=w2563, "1D or 2D Scan?"=w2583, "MCL Scan Axis"=w2583, "Cont. Scan (MCL)"=w2583, "MCL count"=w2570) -> ("FPGA VI Reference Out"=w2585:T15, "error out"=w2584:errorcluster)
            n282 = xnode "Read/Write Control"("FPGA VI Reference In"=w2585, "error in"=w2584, "AI to FIFO"=w2588, "APD to FIFO"=w2588, "Start scan"=w2588, "Start scan (MCL)"=w2588) -> ("FPGA VI Reference Out"=w2590:T15, "error out"=w2589:errorcluster)
          }
        }
        "Raster Scanning..." <- TRUE ("Scanning...")
      }
    }
    n283 = Compound Arithmetic op=OR("Start MCL Scan", "Confocal Image", "Confocal Linescan") -> (w953:bool)
    n284 = And(x="Save Data (MCL)", y=w953) -> (x .and. y?=w1003:bool)
    n285 = case "Start MCL raster scan" shown="True" w953 {
      tunnel: w1006 -> [w1652 w1667]
      tunnel: w1005 -> [w1651 w1666]
      tunnel: [w1652 w1662] -> w888
      tunnel: [w1651 w1661] -> w887
      tunnel: [FALSE w1660] -> w989
      tunnel: "Start MCL Scan" -> [_ w1655]
      tunnel: "Confocal Image" -> [_ w1654]
      tunnel: "Confocal Linescan" -> [_ _]
      frame #0 {
      }
      frame #1 {
        w1660 = TRUE
        n286 = case shown="True" "Restart DMA? (MCL)" {
          tunnel: [w1904 w1907] -> w1665
          tunnel: [w1903 w1906] -> w1664
          tunnel: w1667 -> [w1904 w1912]
          tunnel: w1666 -> [w1903 w1911]
          frame #0 {
          }
          frame #1 {
            w1908 = FALSE ("AI to FIFO")
            n287 = xnode "Read/Write Control"("FPGA VI Reference In"=w1912, "error in"=w1911, "AI to FIFO"=w1908, "APD to FIFO"=w1908) -> ("FPGA VI Reference Out"=w1910:T15, "error out"=w1909:errorcluster)
            n288 = xnode "Invoke Method"("FPGA VI Reference In"=w1910, "error in"=w1909) -> ("FPGA VI Reference Out"=w1914:T15, "error out"=w1913:errorcluster)
            n289 = xnode "Invoke Method"("FPGA VI Reference In"=w1914, "error in"=w1913) -> ("FPGA VI Reference Out"=w1907:T15, "error out"=w1906:errorcluster)
            n290 = local write "Overflow (data lost)"(FALSE ("Overflow (data lost)")) -> ()
          }
        }
        n291 = case shown="False" w1655 {
          selector: w1655 -> [_ w1671]
          tunnel: w1654 -> [w1670 _]
          tunnel: [w1670 w1671] -> w1653
          frame #0 {
            n292 = property on="2D or 1D Scan" class="Bool (strict)"("Val(Sgnl)"=w1670) -> ()  [unwired: 2 in, 2 out]
            n293 = property on="Confocal Image" class="Bool (strict)"("Value"=FALSE ("Start Confocal Map")) -> ()  [unwired: 2 in, 2 out]
          }
          frame #1 {
          }
        }
        n294 = local write "MCL Scanning"(w1660) -> ()
        n295 = local read "AO1"() -> (w1657:dbl)
        n296 = local read "AO2"() -> (w1656:dbl)
        n297 = case shown="True" "Center Scan" {
          tunnel: w1665 -> [w1678 w1787]
          tunnel: w1664 -> [w1677 w1786]
          tunnel: [w1676 w1785] -> w1662
          tunnel: [w1675 w1784] -> w1661
          tunnel: [w1673 w1771] -> w1659
          tunnel: [w1672 w1770] -> w1658
          tunnel: w1657 -> [w1673 w1776]
          tunnel: w1656 -> [w1672 w1779]
          tunnel: w1653 -> [_ _]
          frame #0 {
            w1674 = TRUE ("AI to FIFO")
            n298 = xnode "Read/Write Control"("FPGA VI Reference In"=w1678, "error in"=w1677, "AI to FIFO"=w1674, "APD to FIFO"=w1674, "Start scan (MCL)"=w1674) -> ("FPGA VI Reference Out"=w1676:T15, "error out"=w1675:errorcluster)
          }
          frame #1 {
            w1783 = TRUE ("AI to FIFO")
            n299 = local read "Scan steps (MCL)"() -> (w1762:u64)
            n300 = local read "Scan lines (y)"() -> (w1758:u64)
            n301 = local read "Fast Scan Dir"() -> (w1769:bool)
            n302 = local read "Actual MCL Inc (V)"() -> (w1759:dbl)
            n303 = Decrement(x=w1758) -> (x-1=w1757:u64)
            n304 = Decrement(x=w1762) -> (x-1=w1761:u64)
            n305 = Multiply(x=w1759, y=w1757) -> (x*y=w1756:dbl)
            n306 = Divide(x=w1756, y=2.0) -> (x/y=w1766:dbl)
            n307 = Multiply(x=w1759, y=w1761) -> (x*y=w1760:dbl)
            n308 = Divide(x=w1760, y=2.0) -> (x/y=w1765:dbl)
            n309 = Select(t=w1765, s=w1769, f=w1766) -> (s? t:f=w1764:dbl)
            n310 = Select(t=w1766, s=w1769, f=w1765) -> (s? t:f=w1768:dbl)
            n311 = Subtract(x=w1776, y=w1768) -> (x-y=w1767:dbl)
            n312 = Subtract(x=w1779, y=w1764) -> (x-y=w1763:dbl)
            n313 = local read "2D or 1D Scan"() -> (w1781:bool)
            n314 = Not(x=w1769) -> (.not. x?=w1775:bool)
            n315 = Not(x=w1781) -> (.not. x?=w1777:bool)
            n316 = And(x=w1769, y=w1777) -> (x .and. y?=w1778:bool)
            n317 = And(x=w1777, y=w1775) -> (x .and. y?=w1780:bool)
            n318 = Select(t=w1779, s=w1780, f=w1763) -> (s? t:f=w1770:dbl)
            n319 = Select(t=w1776, s=w1778, f=w1767) -> (s? t:f=w1771:dbl)
            n320 = call "Volt to I16.vi"("Voltage In"=w1771) -> ("I16 Voltage Out"=w1774:i16)
            n321 = call "Volt to I16.vi"("Voltage In"=w1770) -> ("I16 Voltage Out"=w1773:i16)
            n322 = xnode "Read/Write Control"("FPGA VI Reference In"=w1787, "error in"=w1786, "AI to FIFO"=w1783, "APD to FIFO"=w1783, "Start scan (MCL)"=w1783, "AO1"=w1774, "AO2"=w1773) -> ("FPGA VI Reference Out"=w1785:T15, "error out"=w1784:errorcluster)
          }
        }
        "Initial Y" <- w1659
        "Initial X" <- w1658
        "wait to reset values" <- w1660
      }
    }
    n323 = local read "APD Elements/DMA read"() -> (w856:u32)
    n324 = local read "Elements/DMA read"() -> (w911:u32)
    n325 = xnode "Get APD Data"("FPGA VI Reference In"=w888, "error in"=w887, "Number of Elements"=w856, "Timeout (ms)"=-1) -> ("Data"=w855:u32[], "Elements Remaining"=→"APD FIFO Elements Remaining":u32)  [unwired: 2 out]
    n326 = xnode "Get Trap Data"("FPGA VI Reference In"=w888, "error in"=w887, "Number of Elements"=w911, "Timeout (ms)"=-1 ("Timeout")) -> ("FPGA VI Reference Out"=w890:T15, "error out"=w889:errorcluster, "Data"=w1029:u32[], "Elements Remaining"=w1059:u32)
    "FIFO El. Rem." <- w1059
    n327 = local read "FIFO Depth"() -> (w1061:u32)
    n328 = Subtract(x=w1061, y=w911) -> (x-y=w1060:u32)
    n329 = Divide(x=w1059, y=w1060) -> (x/y=w1058:dbl)
    "Buffer Status" <- w1058
    n330 = Equal?(x=w1058, y=1.0) -> (x = y?=w1056:bool)
    n331 = case "Alert buffer overflow" shown="True" w1056 {
      frame #0 {
      }
      frame #1 {
        n332 = call <vilib>:"Beep.vi"() -> ()  [unwired: 3 in, 9 out]
        "Overflow (data lost)" <- TRUE ("Overflow (data lost)")
      }
    }
    n333 = local read "FPGA Averaging"() -> (w910:bool)
    n334 = case "Special unpacking case if no averaging done by FPGA" shown="False" w910 {
      tunnel: w1029 -> [w2064 w2090]
      tunnel: [w2035 w2065] -> w1028
      frame #0 {
        n335 = Decimate 1D Array(w2064) -> (w2063:u32[], w2062:u32[], w2061:u32[], w2060:u32[])
        n336 = Split Number(x=w2063) -> (hi(x)=w2059:u16[], lo(x)=w2058:u16[])
        n337 = Split Number(x=w2062) -> (hi(x)=w2057:u16[], lo(x)=w2056:u16[])
        n338 = Split Number(x=w2061) -> (hi(x)=w2055:u16[], lo(x)=w2054:u16[])
        n339 = Split Number(x=w2060) -> (hi(x)=w2053:u16[], lo(x)=w2052:u16[])
        n340 = To Word Integer(number=w2059) -> (16bit integer=w2051:i16[])
        n341 = To Word Integer(number=w2058) -> (16bit integer=w2050:i16[])
        n342 = To Word Integer(number=w2057) -> (16bit integer=w2049:i16[])
        n343 = To Word Integer(number=w2056) -> (16bit integer=w2048:i16[])
        n344 = To Word Integer(number=w2055) -> (16bit integer=w2047:i16[])
        n345 = To Word Integer(number=w2054) -> (16bit integer=w2046:i16[])
        n346 = To Word Integer(number=w2053) -> (16bit integer=w2045:i16[])
        n347 = To Word Integer(number=w2052) -> (16bit integer=w2044:i16[])
        n348 = To Double Precision Float(number=w2051) -> (double precision float=w2043:dbl[])
        n349 = To Double Precision Float(number=w2050) -> (double precision float=w2042:dbl[])
        n350 = To Double Precision Float(number=w2049) -> (double precision float=w2041:dbl[])
        n351 = To Double Precision Float(number=w2048) -> (double precision float=w2040:dbl[])
        n352 = To Double Precision Float(number=w2047) -> (double precision float=w2039:dbl[])
        n353 = To Double Precision Float(number=w2046) -> (double precision float=w2038:dbl[])
        n354 = To Double Precision Float(number=w2045) -> (double precision float=w2037:dbl[])
        n355 = To Double Precision Float(number=w2044) -> (double precision float=w2036:dbl[])
        n356 = Interleave 1D Arrays(w2043, w2042, w2041, w2040, w2039, w2038, w2037, w2036) -> (w2035:dbl[])
      }
      frame #1 {
        n357 = Decimate 1D Array(w2090) -> (w2081:u32[], w2079:u32[], w2077:u32[], w2075:u32[], w2073:u32[], w2071:u32[], w2069:u32[], w2067:u32[])
        n358 = To Long Integer(number=w2081) -> (32bit integer=w2089:i32[])
        n359 = To Long Integer(number=w2079) -> (32bit integer=w2088:i32[])
        n360 = To Long Integer(number=w2077) -> (32bit integer=w2087:i32[])
        n361 = To Long Integer(number=w2075) -> (32bit integer=w2086:i32[])
        n362 = To Long Integer(number=w2073) -> (32bit integer=w2085:i32[])
        n363 = To Long Integer(number=w2071) -> (32bit integer=w2084:i32[])
        n364 = To Long Integer(number=w2069) -> (32bit integer=w2083:i32[])
        n365 = To Long Integer(number=w2067) -> (32bit integer=w2082:i32[])
        n366 = To Double Precision Float(number=w2089) -> (double precision float=w2080:dbl[])
        n367 = To Double Precision Float(number=w2088) -> (double precision float=w2078:dbl[])
        n368 = To Double Precision Float(number=w2087) -> (double precision float=w2076:dbl[])
        n369 = To Double Precision Float(number=w2086) -> (double precision float=w2074:dbl[])
        n370 = To Double Precision Float(number=w2085) -> (double precision float=w2072:dbl[])
        n371 = To Double Precision Float(number=w2084) -> (double precision float=w2070:dbl[])
        n372 = To Double Precision Float(number=w2083) -> (double precision float=w2068:dbl[])
        n373 = To Double Precision Float(number=w2082) -> (double precision float=w2066:dbl[])
        n374 = Interleave 1D Arrays(w2080, w2078, w2076, w2074, w2072, w2070, w2068, w2066) -> (w2065:dbl[])
      }
    }
    n375 = local read "FPGA Ave."() -> (w909:dbl)
    n376 = feedback #4(i16 -1 ("Trap Sets")) -> (w907:i16)
    n377 = feedback #5("" ("Detector Type")) -> (w904:string)
    n378 = Not Equal?(x=w904, y="Detector Type") -> (x != y?=w902:bool)
    n379 = local read "Trap Sets"() -> (w906:i16)
    n380 = Not Equal?(x=w907, y=w906) -> (x != y?=w901:bool)
    n381 = Or(x=w902, y=w901) -> (x .or. y?=w900:bool)
    n382 = Divide(x=w1028, y=w909) -> (x/y=w1036:dbl[])
    n383 = case "Deinterlace trap data, average down PSD" shown="2" w906 {
      tunnel: w1036 -> [w2109 w2174]
      tunnel: [w2106 w2171] -> w894
      tunnel: [w2109 w2173] -> w1035
      tunnel: "Detector Type" -> [w2108 w2169]
      tunnel: [w2107 w2172] -> w892
      tunnel: [w2105 w2170] -> w1027
      frame #0 {
        n384 = Divide(x=w2109, y=3276.7) -> (x/y=w2110:dbl[])
        n385 = Decimate 1D Array(w2110) -> (w2119:dbl[], w2118:dbl[], w2117:dbl[], w2116:dbl[], w2115:dbl[], w2114:dbl[], w2113:dbl[], w2112:dbl[])
        n386 = case shown="\"IR-QPD + PSD + FB-QPD position\"" w2108 {
          tunnel: w2119 -> [w2143 w2168]
          tunnel: w2118 -> [w2142 w2167]
          tunnel: w2117 -> [w2127 w2145]
          tunnel: w2116 -> [w2128 w2155]
          tunnel: w2115 -> [w2141 w2166]
          tunnel: w2114 -> [w2140 w2165]
          tunnel: w2113 -> [w2124 w2146]
          tunnel: w2112 -> [w2123 w2144]
          tunnel: [w2122 w2152] -> w2107
          tunnel: [w2121 w2151] -> w2106
          tunnel: [w2120 w2150] -> w2105
          frame #0 {
            w2120 = 0  # Channel pattern
            n387 = Divide(x=w2143, y=w2128) -> (x/y=w2130:dbl[])
            n388 = Divide(x=w2142, y=w2128) -> (x/y=w2129:dbl[])
            n389 = Divide(x=w2141, y=w2124) -> (x/y=w2126:dbl[])
            n390 = Divide(x=w2140, y=w2123) -> (x/y=w2125:dbl[])
            n391 = Build Array(w2130, w2129, w2128, w2127, w2126, w2125, w2124, w2123) -> (w2121:dbl[][])
            n392 = Bundle("T1 Y", "T1 X", "T1 Sum", "FB Sum", "PSD Y", "PSD X", "PSD Y Sum", "PSD X Sum") -> (w2139:T32)  [unwired: 1 out]
            n393 = Cluster To Array(cluster=w2139) -> (array=w2122:string[])
          }
          frame #1 {
            w2150 = 3  # Channel pattern
            n394 = Negate(x=w2146) -> (-x=w2147:dbl[])
            n395 = Divide(x=w2168, y=w2155) -> (x/y=w2157:dbl[])
            n396 = Divide(x=w2167, y=w2155) -> (x/y=w2156:dbl[])
            n397 = Divide(x=w2166, y=w2146) -> (x/y=w2154:dbl[])
            n398 = Divide(x=w2165, y=w2147) -> (x/y=w2153:dbl[])
            n399 = Build Array(w2157, w2156, w2155, w2144, w2145, w2154, w2153, w2146) -> (w2151:dbl[][])
            n400 = Bundle("T1 Y", "T1 X", "T1 Sum", "FB X", "FB Sum", "PSD Y", "PSD X", "PSD Y Sum") -> (w2164:T32)  [unwired: 1 out]
            n401 = Cluster To Array(cluster=w2164) -> (array=w2152:string[])
          }
        }
      }
      frame #1 {
        n402 = case shown="\"IR-QPD + PSD + FB-QPD X position\"" w2169 {
          tunnel: w2174 -> [w2235 w2302 w2372]
          tunnel: [w2215 w2287 w2359] -> w2173
          tunnel: [w2201 w2278 w2350] -> w2172
          tunnel: [w2200 w2238 w2317] -> w2171
          tunnel: [w2194 w2276 w2348] -> w2170
          frame #0 {
            w2194 = 1  # Channel pattern
            # "time average x2 the 4th signal and the 4 psd signals (detection laser)"
            # "deinterlace 3 signals from qpd"
            n403 = Decimate 1D Array(w2235) -> (w2234:dbl[], w2233:dbl[], w2199:dbl[], w2232:dbl[], w2222:dbl[], w2220:dbl[], w2219:dbl[], w2217:dbl[])
            n404 = Decimate 1D Array(w2199) -> (w2198:dbl[], w2197:dbl[])
            n405 = Decimate 1D Array(w2234) -> (w2231:dbl[], w2203:dbl[])
            n406 = Decimate 1D Array(w2233) -> (w2230:dbl[], w2228:dbl[])
            n407 = Decimate 1D Array(w2232) -> (w2229:dbl[], w2227:dbl[])
            n408 = call "downsample 1D array - double.vi"("Ave N"=2.0, "Array In"=w2222) -> ("Array Out"=w2221:dbl[])  [unwired: 1 out]
            n409 = call "downsample 1D array - double.vi"("Ave N"=2.0, "Array In"=w2220) -> ("Array Out"=w2202:dbl[])  [unwired: 1 out]
            n410 = call "downsample 1D array - double.vi"("Ave N"=2.0, "Array In"=w2219) -> ("Array Out"=w2218:dbl[])  [unwired: 1 out]
            n411 = call "downsample 1D array - double.vi"("Ave N"=2.0, "Array In"=w2217) -> ("Array Out"=w2216:dbl[])  [unwired: 1 out]
            n412 = Interleave 1D Arrays(w2231, w2230, w2229, w2203, w2228, w2227, w2198, w2197, w2221, w2202, w2218, w2216) -> (w2215:dbl[])
            n413 = Divide(x=w2215, y=3276.7) -> (x/y=w2214:dbl[])
            n414 = Decimate 1D Array(w2214) -> (w2213:dbl[], w2212:dbl[], w2211:dbl[], w2210:dbl[], w2209:dbl[], w2208:dbl[], w2196:dbl[], w2195:dbl[], w2207:dbl[], w2206:dbl[], w2205:dbl[], w2204:dbl[])
            n415 = Divide(x=w2213, y=w2211) -> (x/y=w2181:dbl[])
            n416 = Divide(x=w2212, y=w2211) -> (x/y=w2180:dbl[])
            n417 = Divide(x=w2210, y=w2208) -> (x/y=w2179:dbl[])
            n418 = Divide(x=w2209, y=w2208) -> (x/y=w2178:dbl[])
            n419 = Divide(x=w2207, y=w2205) -> (x/y=w2177:dbl[])
            n420 = Divide(x=w2206, y=w2204) -> (x/y=w2176:dbl[])
            n421 = Build Array(w2181, w2180, w2211, w2179, w2178, w2208, w2196, w2195, w2177, w2176, w2205, w2204) -> (w2200:dbl[][])
            n422 = Bundle("T1 Y", "T1 X", "T1 Sum", "T2 Y", "T2 X", "T2 Sum", "T1 FB Sum", "T2 FB Sum", "PSD Y", "PSD X", "PSD Y Sum", "PSD X Sum") -> (w2182:T33)  [unwired: 1 out]
            n423 = Cluster To Array(cluster=w2182) -> (array=w2201:string[])
          }
          frame #1 {
            w2276 = 2  # Channel pattern
            # "time average x2 the 3 psd signals (detection laser)"
            # "deinterlace 3 signals from qpds"
            n424 = Decimate 1D Array(w2302) -> (w2301:dbl[], w2300:dbl[], w2277:dbl[], w2299:dbl[], w2290:dbl[], w2289:dbl[], w2288:dbl[], w2264:dbl[])
            n425 = Decimate 1D Array(w2277) -> (w2259:dbl[], w2257:dbl[])
            n426 = Decimate 1D Array(w2301) -> (w2298:dbl[], w2279:dbl[])
            n427 = Decimate 1D Array(w2300) -> (w2297:dbl[], w2295:dbl[])
            n428 = Decimate 1D Array(w2299) -> (w2296:dbl[], w2294:dbl[])
            n429 = Decimate 1D Array(w2264) -> (w2260:dbl[], w2258:dbl[])
            n430 = call "downsample 1D array - double.vi"("Ave N"=2.0, "Array In"=w2290) -> ("Array Out"=w2263:dbl[])  [unwired: 1 out]
            n431 = call "downsample 1D array - double.vi"("Ave N"=2.0, "Array In"=w2289) -> ("Array Out"=w2262:dbl[])  [unwired: 1 out]
            n432 = call "downsample 1D array - double.vi"("Ave N"=2.0, "Array In"=w2288) -> ("Array Out"=w2261:dbl[])  [unwired: 1 out]
            n433 = Interleave 1D Arrays(w2298, w2297, w2296, w2279, w2295, w2294, w2260, w2259, w2258, w2257, w2263, w2262, w2261) -> (w2287:dbl[])
            n434 = Divide(x=w2287, y=3276.7) -> (x/y=w2286:dbl[])
            n435 = Decimate 1D Array(w2286) -> (w2285:dbl[], w2284:dbl[], w2283:dbl[], w2282:dbl[], w2281:dbl[], w2280:dbl[], w2249:dbl[], w2247:dbl[], w2246:dbl[], w2244:dbl[], w2243:dbl[], w2242:dbl[], w2239:dbl[])
            n436 = Negate(x=w2239) -> (-x=w2237:dbl[])
            n437 = Divide(x=w2243, y=w2239) -> (x/y=w2241:dbl[])
            n438 = Divide(x=w2242, y=w2237) -> (x/y=w2240:dbl[])
            n439 = Divide(x=w2285, y=w2283) -> (x/y=w2268:dbl[])
            n440 = Divide(x=w2284, y=w2283) -> (x/y=w2267:dbl[])
            n441 = Divide(x=w2282, y=w2280) -> (x/y=w2266:dbl[])
            n442 = Divide(x=w2281, y=w2280) -> (x/y=w2265:dbl[])
            n443 = Divide(x=w2249, y=w2247) -> (x/y=w2248:dbl[])
            n444 = Divide(x=w2246, y=w2244) -> (x/y=w2245:dbl[])
            n445 = Build Array(w2268, w2267, w2283, w2266, w2265, w2280, w2248, w2247, w2245, w2244, w2241, w2240, w2239) -> (w2238:dbl[][])
            n446 = Bundle("T1 Y", "T1 X", "T1 Sum", "T2 Y", "T2 X", "T2 Sum", "T1 FB X", "T1 FB Sum", "T2 FB X", "T2 FB Sum", "PSD Y", "PSD X", "PSD Y Sum") -> (w2269:T34)  [unwired: 1 out]
            n447 = Cluster To Array(cluster=w2269) -> (array=w2278:string[])
          }
          frame #2 {
            w2348 = 4  # Channel pattern
            # "time average x2 the 3 psd signals (detection laser)"
            # "deinterlace 3 signals from qpds"
            n448 = Decimate 1D Array(w2372) -> (w2371:dbl[], w2370:dbl[], w2349:dbl[], w2369:dbl[], w2315:dbl[], w2361:dbl[], w2360:dbl[], w2337:dbl[])
            n449 = Decimate 1D Array "Feedback Sum"(w2349) -> (w2333:dbl[], w2331:dbl[])
            n450 = Decimate 1D Array "QPD Y"(w2371) -> (w2368:dbl[], w2351:dbl[])
            n451 = Decimate 1D Array "QPD X"(w2370) -> (w2367:dbl[], w2365:dbl[])
            n452 = Decimate 1D Array "Feedback Y"(w2315) -> (w2314:dbl[], w2313:dbl[])
            n453 = Decimate 1D Array "QPD Sum"(w2369) -> (w2366:dbl[], w2364:dbl[])
            n454 = Decimate 1D Array "Feedback X"(w2337) -> (w2334:dbl[], w2332:dbl[])
            n455 = call "downsample 1D array - double.vi"("Ave N"=2.0, "Array In"=w2361) -> ("Array Out"=w2336:dbl[])  [unwired: 1 out]
            n456 = call "downsample 1D array - double.vi"("Ave N"=2.0, "Array In"=w2360) -> ("Array Out"=w2335:dbl[])  [unwired: 1 out]
            n457 = Interleave 1D Arrays(w2368, w2367, w2366, w2351, w2365, w2364, w2314, w2334, w2333, w2313, w2332, w2331, w2336, w2335) -> (w2359:dbl[])
            n458 = Divide(x=w2359, y=3276.7) -> (x/y=w2358:dbl[])
            n459 = Decimate 1D Array(w2358) -> (w2357:dbl[], w2356:dbl[], w2355:dbl[], w2354:dbl[], w2353:dbl[], w2352:dbl[], w2310:dbl[], w2324:dbl[], w2308:dbl[], w2309:dbl[], w2322:dbl[], w2306:dbl[], w2320:dbl[], w2318:dbl[])
            n460 = Negate(x=w2318) -> (-x=w2316:dbl[])
            n461 = Divide(x=w2320, y=w2316) -> (x/y=w2319:dbl[])
            n462 = Divide(x=w2309, y=w2306) -> (x/y=w2305:dbl[])
            n463 = Divide(x=w2310, y=w2308) -> (x/y=w2307:dbl[])
            n464 = Divide(x=w2357, y=w2355) -> (x/y=w2341:dbl[])
            n465 = Divide(x=w2356, y=w2355) -> (x/y=w2340:dbl[])
            n466 = Divide(x=w2354, y=w2352) -> (x/y=w2339:dbl[])
            n467 = Divide(x=w2353, y=w2352) -> (x/y=w2338:dbl[])
            n468 = Divide(x=w2324, y=w2308) -> (x/y=w2323:dbl[])
            n469 = Divide(x=w2322, y=w2306) -> (x/y=w2321:dbl[])
            n470 = Build Array(w2341, w2340, w2355, w2339, w2338, w2352, w2307, w2323, w2308, w2305, w2321, w2306, w2319, w2318) -> (w2317:dbl[][])
            n471 = Bundle("T1 Y", "T1 X", "T1 Sum", "T2 Y", "T2 X", "T2 Sum", "T1 FB Y", "T1 FB X", "T1 FB Sum", "T2 FB Y", "T2 FB X", "T2 FB Sum", "PSD X", "PSD Y Sum") -> (w2304:T35)  [unwired: 1 out]
            n472 = Cluster To Array(cluster=w2304) -> (array=w2350:string[])
          }
        }
      }
    }
    n473 = case "Update these things only if detector type or number of traps changes" shown="True" w900 {
      tunnel: w892 -> [_ w1182]
      frame #0 {
      }
      frame #1 {
        n474 = property on="High Res. Display" class="Ring (strict)"("Strings []"=w1182) -> ()  [unwired: 2 in, 2 out]
        n475 = Build Array (concatenate)(w1182, "none") -> (w1175:string[])
        n476 = property on="FFT 1 Choice 1" class="Ring (strict)"("Strings []"=w1175) -> ()  [unwired: 2 in, 2 out]
        n477 = property on="FFT 1 Choice 2" class="Ring (strict)"("Strings []"=w1175) -> ()  [unwired: 2 in, 2 out]
        n478 = property on="FFT 2 Choice 1" class="Ring (strict)"("Strings []"=w1175) -> ()  [unwired: 2 in, 2 out]
        n479 = property on="FFT 2 Choice 2" class="Ring (strict)"("Strings []"=w1175) -> ()  [unwired: 2 in, 2 out]
        n480 = Bundle("APD 1", "APD 2") -> (w1178:cluster{string, string})  [unwired: 1 out]
        n481 = Cluster To Array(cluster=w1178) -> (array=w1176:string[])
        n482 = Build Array (concatenate)(w1176, w1175) -> (w1180:string[])
        n483 = Array Size(array=w1180) -> (size(s)=w1181:i32)
        n484 = property on="Signals to Plot" class="LstBox (strict)"("Item Names"=w1180) -> ()  [unwired: 2 in, 2 out]
        n485 = property on="Signals to Plot" class="LstBox (strict)"("Number of Rows"=w1181) -> ()  [unwired: 2 in, 2 out]
        n486 = property on="All Signals" class="WFChart (strict)"("LegNumRows"=w1181) -> ()  [unwired: 2 in, 2 out]
      }
    }
    n487 = local read "Data points/scans (MCL)"() -> (w998:dbl)
    n488 = Increment(x=w998) -> (x+1=w999:dbl)
    n489 = feedback #6(w999) -> (w1002:dbl)
    n490 = Select(t=0, s=w989, f=w1002) -> (s? t:f=w995:dbl)
    n491 = To Word Integer(number=w1035) -> (16bit integer=w1062:i16[])
    n492 = Decimate 1D Array(w855) -> (w886:u32[], w1025:u32[])
    n493 = To Double Precision Float(number=w886) -> (double precision float=w885:dbl[])
    n494 = Array Size(array=w885) -> (size(s)=w1001:i32)
    n495 = Add(x=w1001, y=w995) -> (x+y=w996:dbl)
    n496 = Greater?(x=w996, y=w998) -> (0:w997:bool)
    n497 = local read "DMA Update Period (s)"() -> (w913:dbl)
    n498 = Select(t=w995, s=w997, f=w996) -> (s? t:f=w994:dbl)
    n499 = Build Array(w886, w1025) -> (w986:u32[][])
    n500 = local read "MCL Scanning"() -> (w992:bool)
    n501 = local read "Data Period (s)"() -> (w871:dbl)
    n502 = To Double Precision Float(number=w986) -> (double precision float=w987:dbl[][])
    n503 = Not(x=w997) -> (.not. x?=w991:bool)
    n504 = local read "APD Integration Time (s)"() -> (w912:dbl)
    n505 = And(x=w991, y=w992) -> (x .and. y?=w993:bool)
    n506 = feedback #7(0.0) -> (w1022:dbl)
    n507 = Add(x=w913, y=w1022) -> (x+y=w1031:dbl)
    n508 = Or(x=w993, y=w989) -> (x .or. y?=w990:bool)
    n509 = Multiply(x=w871, y="Trap Disp. Downsample") -> (x*y=w869:dbl)
    "Display Period (s)" <- w869
    n510 = Equal?(x="Tab Control 6", y=T2."High Res Display") -> (x = y?=w897:bool)
    n511 = for {
      tunnel: [w2104] -> w1021 mode=indexing
      tunnel: w1022 -> [w2103]
      tunnel: "Trap Disp. Downsample" -> [w2100]
      tunnel: w894 -> [w2098] mode=indexing
      tunnel: w871 -> [w2097]
      tunnel: w892 -> [w2096] mode=indexing
      tunnel: w893 -> [w2095]
      tunnel: [w2094] -> w841 mode=indexing
      tunnel: w869 -> [w2093]
      n512 = Bundle By Name("Y"=w2098, "dt"=w2097) -> (w2099:waveform(dbl))  [unwired: 1 out]
      n513 = Set Waveform Attribute(5:w2096, 6:w2095, 7:w2099) -> (3:w2094:waveform(dbl))  [unwired: 1 in, 2 out]
      n514 = call "downsample 1D array - double.vi"("Ave N"=w2100, "Array In"=w2098) -> ("Array Out"=w2101:dbl[])  [unwired: 1 out]
      n515 = To Time Stamp(1:w2103) -> (0:w2102:timestamp)
      n516 = Bundle By Name(cluster=w2094, "t0"=w2102, "Y"=w2101, "dt"=w2093) -> (w2104:waveform(dbl))
    }
    n517 = case "For plotting results of scanning MCL" shown="True" w990 {
      tunnel: w989 -> [_ w1607]
      tunnel: w885 -> [_ w1640]
      tunnel: w998 -> [_ _]
      tunnel: w841 -> [_ w1586]
      tunnel: w842 -> [_ w1554]
      frame #0 {
      }
      frame #1 {
        w1552 = u32 0 items=["Horizontal", "Vertical", "Central", "1st Diagonal", "2nd Diagonal"] ("Type of Symmetry")
        n518 = Index Array(array=w1586, index=11) -> (element=w1590:waveform(dbl))
        n519 = Index Array(array=w1586, index=10) -> (element=w1594:waveform(dbl))
        n520 = Index Array(array=w1586, index="Channel") -> (element=w1588:waveform(dbl))
        n521 = Unbundle By Name(w1590) -> ("Y"=w1589:dbl[])
        n522 = Unbundle By Name(w1594) -> ("Y"=w1593:dbl[])
        n523 = Unbundle By Name(w1588) -> ("Y"=w1585:dbl[])
        n524 = feedback #8(w1640) -> (w1641:dbl[])
        n525 = Build Array (concatenate)(w1641, w1640) -> (w1596:dbl[])
        n526 = Select(t=w1640, s=w1607, f=w1596) -> (s? t:f=w1601:dbl[])
        n527 = feedback #9(w1593) -> (w1608:dbl[])
        n528 = Build Array (concatenate)(w1608, w1593) -> (w1592:dbl[])
        n529 = feedback #10(w1585) -> (w1638:dbl[])
        n530 = Build Array (concatenate)(w1638, w1585) -> (w1637:dbl[])
        n531 = feedback #11(w1589) -> (w1616:dbl[])
        n532 = Build Array (concatenate)(w1616, w1589) -> (w1617:dbl[])
        n533 = Select(t=w1593, s=w1607, f=w1592) -> (s? t:f=w1609:dbl[])
        n534 = Select(t=w1585, s=w1607, f=w1637) -> (s? t:f=w1636:dbl[])
        n535 = Select(t=w1589, s=w1607, f=w1617) -> (s? t:f=w1618:dbl[])
        n536 = local read "N APD Samp/step"() -> (w1600:dbl)
        n537 = Array Size(array=w1609) -> (size(s)=w1610:i32)
        n538 = Array Size(array=w1636) -> (size(s)=w1635:i32)
        n539 = Array Size(array=w1618) -> (size(s)=w1619:i32)
        n540 = local read "Scan steps (MCL)"() -> (w1549:u64)
        n541 = local read "Scan lines (y)"() -> (w1584:u64)
        n542 = call "integrate 1D array interval - double.vi"("Ave N"=w1600, "Array In"=w1601) -> ("Array Out"=w1599:dbl[])  [unwired: 1 out]
        n543 = Array Size(array=w1599) -> (size(s)=w1606:i32)
        n544 = Divide(x=w1610, y=w1606) -> (x/y=w1611:dbl)
        n545 = call "downsample 1D array - double.vi"("Ave N"=w1611, "Array In"=w1609) -> ("Array Out"=w1613:dbl[])  [unwired: 1 out]
        n546 = Divide(x=w1635, y=w1606) -> (x/y=w1634:dbl)
        n547 = call "downsample 1D array - double.vi"("Ave N"=w1634, "Array In"=w1636) -> ("Array Out"=w1627:dbl[])  [unwired: 1 out]
        n548 = Divide(x=w1619, y=w1606) -> (x/y=w1620:dbl)
        n549 = call "downsample 1D array - double.vi"("Ave N"=w1620, "Array In"=w1618) -> ("Array Out"=w1622:dbl[])  [unwired: 1 out]
        n550 = Multiply(x=w1549, y=u64 2) -> (x*y=w1604:u64)
        n551 = Multiply(x=w1584, y=w1604) -> (x*y=w1632:u64)
        n552 = Subtract(x=w1632, y=w1606) -> (x-y=w1605:u64)
        n553 = call <vilib>:"Mean.vi"("X"=w1599) -> ("mean"=w1631:dbl)  [unwired: 1 out]
        n554 = call <vilib>:"Mean.vi"("X"=w1613) -> ("mean"=w1612:dbl)  [unwired: 1 out]
        n555 = call <vilib>:"Mean.vi"("X"=w1627) -> ("mean"=w1628:dbl)  [unwired: 1 out]
        n556 = call <vilib>:"Mean.vi"("X"=w1622) -> ("mean"=w1621:dbl)  [unwired: 1 out]
        n557 = Initialize Array(w1631, w1605) -> (w1630:dbl[])
        n558 = Initialize Array(w1612, w1605) -> (w1614:dbl[])
        n559 = Initialize Array(w1628, w1605) -> (w1626:dbl[])
        n560 = Initialize Array(w1621, w1605) -> (w1623:dbl[])
        n561 = Build Array (concatenate)(w1599, w1630) -> (w1629:dbl[])
        n562 = Build Array (concatenate)(w1613, w1614) -> (w1615:dbl[])
        n563 = Build Array (concatenate)(w1627, w1626) -> (w1625:dbl[])
        n564 = Build Array (concatenate)(w1622, w1623) -> (w1624:dbl[])
        n565 = Reshape Array(w1629, w1584, w1604) -> (w1582:dbl[][])
        n566 = Reshape Array(w1615, w1584, w1604) -> (w1563:dbl[][])
        n567 = Reshape Array(w1625, w1584, w1604) -> (w1555:dbl[][])
        n568 = Reshape Array(w1624, w1584, w1604) -> (w1571:dbl[][])
        n569 = Index Array(array=w1582, index (row)=0) -> (element=→"Waveform Graph":dbl[])  [unwired: 1 in]
        n570 = Array Subset(array=w1571, index (col)=0 ("index"), length (col)=w1549) -> (w1577:dbl[][])  [unwired: 2 in]
        n571 = Array Subset(array=w1582, index (col)=0 ("index"), length (col)=w1549) -> (w1581:dbl[][])  [unwired: 2 in]
        n572 = Array Subset(array=w1571, index (col)=w1549) -> (w1575:dbl[][])  [unwired: 3 in]
        n573 = Array Subset(array=w1582, index (col)=w1549) -> (w1579:dbl[][])  [unwired: 3 in]
        n574 = Array Subset(array=w1555, index (col)=0 ("index"), length (col)=w1549) -> (w1561:dbl[][])  [unwired: 2 in]
        n575 = Array Subset(array=w1555, index (col)=w1549) -> (w1559:dbl[][])  [unwired: 3 in]
        n576 = Array Subset(array=w1563, index (col)=0 ("index"), length (col)=w1549) -> (w1569:dbl[][])  [unwired: 2 in]
        n577 = Array Subset(array=w1563, index (col)=w1549) -> (w1567:dbl[][])  [unwired: 3 in]
        n578 = for {
          tunnel: w1577 -> [w1647] mode=indexing
          tunnel: [w1646] -> w1576 mode=indexing
          n579 = Reverse 1D Array(array=w1647) -> (reversed array=w1646:dbl[])
        }
        n580 = for {
          tunnel: w1581 -> [w1649] mode=indexing
          tunnel: [w1648] -> w1580 mode=indexing
          n581 = Reverse 1D Array(array=w1649) -> (reversed array=w1648:dbl[])
        }
        n582 = for {
          tunnel: w1561 -> [w1643] mode=indexing
          tunnel: [w1642] -> w1560 mode=indexing
          n583 = Reverse 1D Array(array=w1643) -> (reversed array=w1642:dbl[])
        }
        n584 = for {
          tunnel: w1569 -> [w1645] mode=indexing
          tunnel: [w1644] -> w1568 mode=indexing
          n585 = Reverse 1D Array(array=w1645) -> (reversed array=w1644:dbl[])
        }
        n586 = Add(x=w1576, y=w1575) -> (x+y=w1574:dbl[][])
        n587 = Add(x=w1580, y=w1579) -> (x+y=w1551:dbl[][])
        n588 = Add(x=w1560, y=w1559) -> (x+y=w1558:dbl[][])
        n589 = Add(x=w1568, y=w1567) -> (x+y=w1566:dbl[][])
        n590 = Divide(x=w1574, y=2) -> (x/y=w1572:dbl[][])
        n591 = Divide(x=w1558, y=2) -> (x/y=w1556:dbl[][])
        n592 = Transpose 2D Array(2D array=w1572) -> (transposed array=→"PSD X map":dbl[][])
        n593 = Divide(x=w1566, y=2) -> (x/y=w1564:dbl[][])
        n594 = To Single Precision Float(number=w1551) -> (single precision float=w1550:sgl[][])
        n595 = Transpose 2D Array(2D array=w1564) -> (transposed array=→"PSD Y map":dbl[][])
        n596 = Transpose 2D Array(2D array=w1556) -> (transposed array=→"Data map":dbl[][])
        n597 = call "IMAQ ArrayToImage"("Image Pixels (Float)"=w1550, "Image"=w1554) -> ("Image Out"=w1553:T1)  [unwired: 8 in, 1 out]
        n598 = call "IMAQ Symmetry"("Type of Symmetry"=w1552, "Image Src"=w1553) -> ("Image Dst Out"=w1547:T1)  [unwired: 3 in, 1 out]
        n599 = call "IMAQ Set Simple Calibration"("Calibration Axis Info"=T24 {"Origin Pixel"={"X"=0.0, "Y"=0.0}, "Angle Relative to Horizontal (deg)"=0.0, "Axis Reference"=0}, "Grid Descriptor"=T25 {"X Step"=0.3, "Y Step"=0.3, "Unit"=enum."Undefined"}, "Image"=w1547) -> ("Calibrated Image"=→"APD 1b":T1)  [unwired: 7 in, 1 out]
      }
    }
    n600 = Reciprocal(x=w869) -> (1/x=→"Trap Disp. Freq. (Hz)":dbl)
    n601 = case shown="True" w897 {
      tunnel: w841 -> [_ w1151]
      frame #0 {
      }
      frame #1 {
        n602 = Index Array(array=w1151, index="High Res. Display") -> (element=w1152:waveform(dbl))
        n603 = call <vilib>:"Std Deviation and Variance.vi"("X"=w1152) -> ("mean"=w1159:dbl, "standard deviation"=w1164:dbl)  [unwired: 1 in, 1 out]
        "Mean Intensity" <- w1159
        "Sigma" <- w1164
        n604 = Subtract(x=w1152, y=w1159) -> (x-y=w1158:waveform(dbl))
        n605 = Select(t=w1158, s="Subtract mean", f=w1152) -> (s? t:f=→"1 Channel":waveform(dbl))
        n606 = Divide(x=w1164, y=w1159) -> (x/y=→"Sigma/Mean":dbl)
        n607 = feedback #12(1) -> (w1153:i32)
        n608 = Greater Or Equal?(x=w1153, y="Slow mean N ave.") -> (x >= y?=w1166:bool)
        n609 = Increment(x=w1153) -> (x+1=w1168:i32)
        n610 = Select(t=1, s=w1166, f=w1168) -> (s? t:f=w1155:i32)
        n611 = feedback #13() -> (w1156:waveform(dbl))  [unwired: 1 out]
        n612 = case shown="Default" w1153 {
          tunnel: [w1171 w1174] -> w1157
          tunnel: w1156 -> [w1173 _]
          tunnel: w1152 -> [w1172 w1174]
          frame #0 {
            n613 = call-poly <vilib>:"Append Waveforms.vi"("waveform B"=w1172, "waveform A"=w1173) -> ("waveform out"=w1171:waveform(dbl))  [unwired: 1 in, 8 out]
          }
          frame #1 {
          }
        }
        n614 = case shown="True" w1166 {
          tunnel: w1157 -> [_ w1170]
          frame #0 {
          }
          frame #1 {
            n615 = call <vilib>:"Mean.vi"("X"=w1170) -> ("mean"=→"Slow mean":dbl)  [unwired: 1 out]
          }
        }
      }
    }
    n616 = case "For computing FFTs for display" shown="True" "Compute FFT" {
      tunnel: w841 -> [_ w2988]
      frame #0 {
      }
      frame #1 {
        n617 = Build Array("FFT 1 Choice 1", "FFT 1 Choice 2", "FFT 2 Choice 1", "FFT 2 Choice 2") -> (w2981:u16[])
        n618 = Array Size(array=w2988) -> (size(s)=w2987:i32)
        n619 = feedback #14(u16[] [100, 100, 100, 100]) -> (w2982:u16[])
        n620 = feedback #15("# Spectra to Ave.") -> (w2979:dbl)
        n621 = Not Equal?(x="# Spectra to Ave.", y=w2979) -> (x != y?=w2978:bool)
        n622 = Not Equal?(x=w2981, y=w2982) -> (x != y?=w2980:bool)
        n623 = feedback #16(1.0) -> (w2965:dbl)
        n624 = Compound Arithmetic op=OR("Reset FFT", w2980, w2978) -> (w2963:bool)
        n625 = Select(t=1.0, s=w2963, f=w2965) -> (s? t:f=w2967:dbl)
        n626 = Greater?(x=w2967, y="# Spectra to Ave.") -> (0:w2986:bool)
        n627 = Increment(x=w2967) -> (x+1=w2966:dbl)
        n628 = local read "DMA Update Period (s)"() -> (w2961:dbl)
        n629 = Multiply(x="# Spectra to Ave.", y=w2961) -> (x*y=→"Ave. Time (s)":dbl)
        n630 = Build Array(cluster{"f0":dbl, "df":dbl, "magnitude":dbl[]} {"f0"=0.0, "df"=0.0, "magnitude"=[]} ("PSD")) -> (w2970:cluster{"f0":dbl, "df":dbl, "magnitude":dbl[]}[])
        n631 = Build Array(w2970, w2970, w2970, w2970) -> (w2972:T36)
        n632 = feedback #17(w2972) -> (w2977:T36)
        n633 = for {
          N: 4 -> [_]
          tunnel: w2981 -> [w3010] mode=indexing
          tunnel: w2988 -> [w3011]
          tunnel: w2987 -> [w3013]
          tunnel: w2963 -> [w3006]
          tunnel: w2986 -> [w3005]
          tunnel: "# Spectra to Ave." -> [w3004]
          tunnel: [w3003] -> w2976 mode=indexing
          tunnel: w2977 -> [w3008] mode=indexing
          tunnel: [w3007] -> w2964 mode=indexing
          tunnel: w2967 -> [w3002]
          n634 = Less?(x=w3010, y=w3013) -> (x < y?=w3012:bool)
          n635 = Index Array(array=w3011, index=w3010) -> (element=w3009:waveform(dbl))
          n636 = case shown="True" w3012 {
            tunnel: w3009 -> [_ w3030]
            tunnel: w3008 -> [w3015 w3028]
            tunnel: [w3015 w3016] -> w3007
            tunnel: w3006 -> [_ w3027]
            tunnel: w3005 -> [_ w3020]
            tunnel: w3004 -> [_ w3019]
            tunnel: [cluster{"f0":dbl, "df":dbl, "magnitude":dbl[]} {"f0"=0.0, "df"=0.0, "magnitude"=[]} ("PSD") w3021] -> w3003
            tunnel: w3002 -> [_ w3018]
            frame #0 {
            }
            frame #1 {
              n637 = call <vilib>:"Std Deviation and Variance.vi"("X"=w3030) -> ("mean"=w3031:dbl)  [unwired: 1 in, 2 out]
              n638 = Subtract(x=w3030, y=w3031) -> (x-y=w3029:waveform(dbl))
              n639 = xnode "Spectral Measurements"("Signals"=w3029) -> ("PSD"=w3023:cluster{"f0":dbl, "df":dbl, "magnitude":dbl[]})  [unwired: 1 in, 1 out]
              n640 = case shown="False" w3027 {
                tunnel: w3028 -> [w3040 _]
                tunnel: [w3036 w3045] -> w3016
                tunnel: w3023 -> [w3039 w3046]
                tunnel: w3020 -> [w3038 _]
                frame #0 {
                  n641 = Build Array (concatenate)(w3040, w3039) -> (w3037:cluster{"f0":dbl, "df":dbl, "magnitude":dbl[]}[])
                  n642 = case shown="True" w3038 {
                    tunnel: w3037 -> [w3041 w3044]
                    tunnel: [w3041 w3042] -> w3036
                    frame #0 {
                    }
                    frame #1 {
                      n643 = Delete From Array(array=w3044, index=0) -> (array with subset deleted=w3042:cluster{"f0":dbl, "df":dbl, "magnitude":dbl[]}[])  [unwired: 1 in, 1 out]
                    }
                  }
                }
                frame #1 {
                  n644 = Build Array(w3046) -> (w3045:cluster{"f0":dbl, "df":dbl, "magnitude":dbl[]}[])
                }
              }
              n645 = for {
                tunnel: w3016 -> [w3035] mode=indexing
                tunnel: [w3034] -> w3026 mode=indexing
                n646 = Unbundle By Name(w3035) -> ("magnitude"=w3034:dbl[])
              }
              n647 = Transpose 2D Array(2D array=w3026) -> (transposed array=w3025:dbl[][])
              n648 = for {
                tunnel: w3025 -> [w3033] mode=indexing
                tunnel: [w3032] -> w3024 mode=indexing
                n649 = Add Array Elements(numeric array=w3033) -> (sum=w3032:dbl)
              }
              n650 = Select(t=w3019, s=w3020, f=w3018) -> (s? t:f=w3017:dbl)
              n651 = Divide(x=w3024, y=w3017) -> (x/y=w3022:dbl[])
              n652 = Bundle By Name(cluster=w3023, "magnitude"=w3022) -> (w3021:cluster{"f0":dbl, "df":dbl, "magnitude":dbl[]})
            }
          }
        }
        n653 = case shown="True" w2963 {
          tunnel: w2964 -> [w2995 w3001]
          tunnel: [w2995 w2996] -> w2962
          frame #0 {
          }
          frame #1 {
            n654 = Array Subset(array=w3001, index (row)=0 ("index"), length (row)=4 ("length"), index (col)=0 ("index"), length (col)=1 ("length")) -> (w2996:T36)
          }
        }
        n655 = Split 1D Array(array=w2976, index=2) -> (first subarray=→"FFT 1":cluster{"f0":dbl, "df":dbl, "magnitude":dbl[]}[], second subarray=→"FFT 2":cluster{"f0":dbl, "df":dbl, "magnitude":dbl[]}[])
      }
    }
    n656 = Bundle("APD 1", "APD 2") -> (w1019:cluster{string, string})  [unwired: 1 out]
    n657 = Cluster To Array(cluster=w1019) -> (array=w1016:string[])
    n658 = for {
      tunnel: w987 -> [w2024] mode=indexing
      tunnel: w1022 -> [w2033]
      tunnel: w912 -> [w2032]
      tunnel: [w2028] -> w1020 mode=indexing
      tunnel: "APD Disp. Scale" -> [w2029]
      tunnel: w893 -> [w2027]
      tunnel: w1016 -> [w2026] mode=indexing
      tunnel: "APD Disp. Downsample" -> [w2022]
      tunnel: [w2025] -> w1015
      n659 = call "integrate 1D array interval - double.vi"("Ave N"=w2022, "Array In"=w2024) -> ("Array Out"=w2023:dbl[])  [unwired: 1 out]
      n660 = Multiply(x=w2032, y=w2022) -> (x*y=w2025:dbl)
      n661 = Divide(x=w2023, y=w2029) -> (x/y=w2030:dbl[])
      n662 = To Time Stamp(1:w2033) -> (0:w2034:timestamp)
      n663 = Bundle By Name("t0"=w2034, "Y"=w2030, "dt"=w2025) -> (w2031:waveform(dbl))  [unwired: 1 out]
      n664 = Set Waveform Attribute(5:w2026, 6:w2027, 7:w2031) -> (3:w2028:waveform(dbl))  [unwired: 1 in, 2 out]
    }
    "APD Display Period (s)" <- w1015
    n665 = Reciprocal(x=w1015) -> (1/x=→"APD Display Freq. (Hz)":dbl)
    n666 = feedback #18(w886) -> (w985:u32[])
    n667 = Build Array (concatenate)(w985, w886) -> (w982:u32[])
    n668 = Array Size(array=w982) -> (size(s)=w979:i32)
    n669 = Array Size(array=w886) -> (size(s)=w981:i32)
    n670 = Build Array (concatenate)(w1020, w1021) -> (w914:waveform(dbl)[])
    "All Signals" <- w914
    n671 = local read "APD Integration Time (s)"() -> (w846:dbl)
    n672 = Multiply(x=w981, y="APD Ave N") -> (x*y=w980:dbl)
    n673 = Greater?(x=w979, y=w980) -> (0:w983:bool)
    n674 = Index Array(array=w914, index=0) -> (element=w972:waveform(dbl))
    n675 = case shown="True" w983 {
      tunnel: w982 -> [w1539 w1544]
      tunnel: [w1539 w1540] -> w919
      tunnel: w980 -> [_ w1542]
      tunnel: w979 -> [_ w1543]
      frame #0 {
      }
      frame #1 {
        n676 = Subtract(x=w1543, y=w1542) -> (x-y=w1541:dbl)
        n677 = Array Subset(array=w1544, index=w1541, length=w1542) -> (w1540:u32[])
      }
    }
    n678 = Multiply(x="APD Disp. Scale", y=w972) -> (x*y=w848:waveform(dbl))
    n679 = Multiply(x="APD Disp. Downsample", y=w846) -> (x*y=w843:dbl)
    n680 = Divide(x=w848, y=w843) -> (x/y=→"APD 1 Chart":waveform(dbl))
    n681 = Index Array(array=w914, index=3) -> (element=w931:waveform(dbl))
    n682 = Index Array(array=w914, index=6) -> (element=w928:waveform(dbl))
    n683 = Array Size(array=w919) -> (size(s)=w977:i32)
    n684 = Add Array Elements(numeric array=w919) -> (sum=w988:u32)
    n685 = call <vilib>:"Std Deviation and Variance.vi"("X"=w919) -> ("standard deviation"=w918:dbl)  [unwired: 1 in, 2 out]
    n686 = Divide(x="T1 offset_x (mV)", y=1000.0) -> (x/y=w932:dbl)
    n687 = Multiply(x=w912, y=w977) -> (x*y=w978:dbl)
    "Int. Time (s)" <- w978
    n688 = Divide(x=w988, y=w978) -> (x/y=w916:dbl)
    "APD 1 Rate (Hz)" <- w916
    n689 = Divide(x=w918, y=w912) -> (x/y=w917:dbl)
    "Rate sigma (Hz)" <- w917
    n690 = Divide(x=w917, y=w916) -> (x/y=→"sigma/mean":dbl)
    n691 = Divide(x="T2 offset_x (mV)", y=1000.0) -> (x/y=w930:dbl)
    n692 = case shown="0, Default" "Calibration" {
      tunnel: "T1 alpha_x (nm/V)" -> [_ w1516 w1537]
      tunnel: "T1 kappa_x (pN/nm)" -> [_ _ w1527]
      tunnel: "T2 alpha_x (nm/V)" -> [_ w1515 w1535]
      tunnel: "T2 kappa_x (pN/nm)" -> [_ _ w1528]
      tunnel: w931 -> [w1498 w1513 w1533]
      tunnel: w928 -> [w1497 w1511 w1531]
      tunnel: [w1498 w1510 w1530] -> w961
      tunnel: [w1497 w1509 w1529] -> w960
      tunnel: ["T1 X (V)" ("Label.Text") "T1 X (nm)" ("Label.Text") "T1 X (pN)" ("Label.Text")] -> w949
      tunnel: ["T2 X (V)" ("Label.Text") "T2 X (nm)" ("Label.Text") "T2 X (pN)" ("Label.Text")] -> w948
      tunnel: ["Position (V)" ("Label.Text") "Position (nm)" ("Label.Text") "Force (pN)" ("Label.Text")] -> w950
      tunnel: w930 -> [_ w1501 w1520]
      tunnel: w932 -> [_ w1504 w1522]
      tunnel: ["Mean (V)" ("Label.Text") "Mean (nm)" ("Label.Text") "Mean (pN)" ("Label.Text")] -> w945
      tunnel: ["Difference (V)" ("Label.Text") "Difference (nm)" ("Label.Text") "Difference (pN)" ("Label.Text")] -> w849
      frame #0 {
      }
      frame #1 {
        n693 = Unbundle By Name(w1513) -> ("Y"=w1517:dbl[])
        n694 = Unbundle By Name(w1511) -> ("Y"=w1502:dbl[])
        n695 = Subtract(x=w1517, y=w1504) -> (x-y=w1505:dbl[])
        n696 = Subtract(x=w1502, y=w1501) -> (x-y=w1503:dbl[])
        n697 = Multiply(x=w1503, y=w1515) -> (x*y=w1512:dbl[])
        n698 = Multiply(x=w1516, y=w1505) -> (x*y=w1514:dbl[])
        n699 = Bundle By Name(cluster=w1511, "Y"=w1512) -> (w1509:waveform(dbl))
        n700 = Bundle By Name(cluster=w1513, "Y"=w1514) -> (w1510:waveform(dbl))
      }
      frame #2 {
        n701 = Unbundle By Name(w1533) -> ("Y"=w1538:dbl[])
        n702 = Unbundle By Name(w1531) -> ("Y"=w1536:dbl[])
        n703 = Subtract(x=w1536, y=w1520) -> (x-y=w1521:dbl[])
        n704 = Subtract(x=w1538, y=w1522) -> (x-y=w1523:dbl[])
        n705 = Compound Arithmetic op=MULTIPLY(w1521, w1535, w1528) -> (w1532:dbl[])
        n706 = Compound Arithmetic op=MULTIPLY(w1527, w1537, w1523) -> (w1534:dbl[])
        n707 = Bundle By Name(cluster=w1531, "Y"=w1532) -> (w1529:waveform(dbl))
        n708 = Bundle By Name(cluster=w1533, "Y"=w1534) -> (w1530:waveform(dbl))
      }
    }
    n709 = feedback #19(u16 1 ("Calibration")) -> (w952:u16)
    n710 = case shown="True" "Read Lateness and Rel Phase" {
      tunnel: w890 -> [w1184 w1202]
      tunnel: w889 -> [w1185 w1201]
      tunnel: [w1184 w1200] -> w922
      tunnel: [w1185 w1199] -> w921
      frame #0 {
      }
      frame #1 {
        n711 = xnode "Read/Write Control"("FPGA VI Reference In"=w1202, "error in"=w1201) -> ("FPGA VI Reference Out"=w1200:T15, "error out"=w1199:errorcluster, "GI Relative phase"=→"GI relative phase":i16, "Relative phase"=→"Relative phase (AI1)":i16, "AI Late Counter"=→"Late Counter (AI1)":u32, "GI Late Counter"=→"GI Late Counter":u32, "MCL Late Counter"=→"MCL Late Counter":u32, "MCL Relative Phase"=→"Relative Phase (MCL)":i16, "APD Acq Relative Phase"=→"APD Acq Relative Phase":i16, "APD Gate Relative Phase"=→"APD Gate Relative Phase":i16, "APD Acq Late Counter"=→"APD Acq Late Counter":u32, "APD Gate Late Counter"=→"APD Gate Late Counter":u32, "Green FB Relative Phase"=→"Relative phase (Green FB)":i16, "GI Relative phase 2"=→"GI relative phase 2":i16, "GI Late Counter 2"=→"GI Late Counter 2":u32)
      }
    }
    n712 = Not Equal?(x=w952, y="Calibration") -> (x != y?=w895:bool)
    n713 = Unbundle By Name(w931) -> ("Y"=w934:dbl[])
    n714 = Unbundle By Name(w928) -> ("Y"=w937:dbl[])
    n715 = Subtract(x=w934, y=w932) -> (x-y=w935:dbl[])
    n716 = Subtract(x=w937, y=w930) -> (x-y=w936:dbl[])
    n717 = Multiply(x=w936, y="T2 alpha_x (nm/V)") -> (x*y=w927:dbl[])
    n718 = Multiply(x="T1 alpha_x (nm/V)", y=w935) -> (x*y=w926:dbl[])
    n719 = Multiply(x=w960, y=-1.0) -> (x*y=w939:waveform(dbl))
    n720 = Subtract(x=w927, y=w926) -> (x-y=w924:dbl[])
    n721 = Unbundle By Name(w960) -> ("Y"=w877:dbl[])
    n722 = Unbundle By Name(w961) -> ("Y"=w878:dbl[])
    n723 = Build Array(w961, w939) -> (→"Force":waveform(dbl)[])
    n724 = Subtract(x=w924, y="Offset (nm)") -> (x-y=w875:dbl[])
    n725 = call <vilib>:"Mean.vi"("X"=w877) -> ("mean"=w853:dbl)  [unwired: 1 out]
    "T2 X" <- w853
    n726 = Absolute Value(x=w878) -> (abs(x)=w879:dbl[])
    n727 = Absolute Value(x=w877) -> (abs(x)=w880:dbl[])
    n728 = call <vilib>:"Mean.vi"("X"=w878) -> ("mean"=w854:dbl)  [unwired: 1 out]
    "T1 X" <- w854
    n729 = Add(x=w879, y=w880) -> (x+y=w881:dbl[])
    n730 = Bundle By Name(cluster=w931, "Y"=w875) -> (→"Bead Separation":waveform(dbl))
    n731 = Divide(x=w881, y=2.0) -> (x/y=→"Vec Mean of T1 T2":dbl[])
    n732 = case shown="True" w895 {
      tunnel: w950 -> [_ w1491]
      tunnel: w949 -> [_ w1490]
      tunnel: w948 -> [_ w1489]
      tunnel: w945 -> [_ w1488]
      tunnel: w849 -> [_ w1487]
      frame #0 {
      }
      frame #1 {
        n733 = property on="Force" class="WFChart (strict)"("YScale.NameLbl.Text"=w1491) -> ()  [unwired: 2 in, 2 out]
        n734 = property on="T2 X" class="DigNum (strict)"("Caption.Text"=w1489) -> ()  [unwired: 2 in, 2 out]
        n735 = property on="T1 X" class="DigNum (strict)"("Caption.Text"=w1490) -> ()  [unwired: 2 in, 2 out]
        n736 = property on="Mean" class="DigNum (strict)"("Caption.Text"=w1488) -> ()  [unwired: 2 in, 2 out]
        n737 = property on="Difference" class="DigNum (strict)"("Caption.Text"=w1487) -> ()  [unwired: 2 in, 2 out]
      }
    }
    n738 = local read "Tether"() -> (w884:bool)
    n739 = Absolute Value(x=w854) -> (abs(x)=w851:dbl)
    n740 = Absolute Value(x=w853) -> (abs(x)=w850:dbl)
    n741 = local read "Display Period (s)"() -> (w868:dbl)
    n742 = Add(x=w851, y=w850) -> (x+y=w947:dbl)
    n743 = Subtract(x=w851, y=w850) -> (x-y=→"Difference":dbl)
    n744 = feedback #20(w875) -> (w874:dbl[])
    n745 = Divide(x=w947, y=2.0) -> (x/y=w883:dbl)
    "Mean" <- w883
    n746 = case shown="True" w884 {
      tunnel: w883 -> [_ w1140]
      frame #0 {
      }
      frame #1 {
        n747 = Greater?(x="Lost Tether Alarm Threshold (pN)", y=w1140) -> (0:w1138:bool)
        n748 = case shown="True" w1138 {
          frame #0 {
          }
          frame #1 {
            n749 = local read "Time tether formed"() -> (w1146:timestamp)
            n750 = Get Date/Time In Seconds() -> (seconds since 1Jan1904=w1147:timestamp)
            n751 = Subtract(x=w1147, y=w1146) -> (x-y=w1145:dbl)
            n752 = Number To Decimal String(number=w1145) -> (decimal integer string=w1142:string)  [unwired: 1 out]
            n753 = local read "Messages"() -> (w1149:string)
            n754 = call <vilib>:"Beep.vi"() -> ()  [unwired: 3 in, 9 out]
            n755 = Concatenate Strings("Lost tether (" ("Message to add"), w1142, " s)." ("string")) -> (w1144:string)
            n756 = local write "Tether"(FALSE ("Tether")) -> ()
            n757 = call "Update messages.vi"("Message to add"=w1144, "Old message string"=w1149) -> ("New message string"=w1148:string)
            n758 = local write "Messages"(w1148) -> ()
          }
        }
      }
    }
    n759 = Build Array (concatenate)(w875, w874) -> (w873:dbl[])
    n760 = Divide(x="Bead Sep. Int. Time (s)", y=w868) -> (x/y=w867:dbl)
    n761 = Split 1D Array(array=w873, index=w867) -> (first subarray=w866:dbl[])  [unwired: 1 out]
    n762 = xnode "Read/Write Control"("FPGA VI Reference In"=w922, "error in"=w921) -> ("FPGA VI Reference Out"=w1051:T15, "error out"=w1045:errorcluster, "AI2 Y Sum Set 1"=w1041:i16, "AI2 Y Sum Set 2"=w1040:i16, "Scanning"=→"AOD Scanning":bool, "Scan I"=→"AOD Scan I":u64, "Scanning MCL"=w1043:bool, "Scan I (MCL)"=→"MCL Scan I":u64, "Green FB Signals"=w970:T29)  [unwired: 1 out]
    "MCL Scanning" <- w1043
    n763 = call <vilib>:"Mean.vi"("X"=w866) -> ("mean"=w865:dbl)  [unwired: 1 out]
    "Bead Mean (nm)" <- w865
    n764 = Subtract(x=w866, y=w865) -> (x-y=w864:dbl[])
    n765 = Square(x=w864) -> (x^2=w863:dbl[])
    n766 = call <vilib>:"Mean.vi"("X"=w863) -> ("mean"=w862:dbl)  [unwired: 1 out]
    n767 = Square Root(x=w862) -> (sqrt(x)=w861:dbl)
    n768 = Multiply(x=10.0, y=w861) -> (x*y=→"RMS (Ang)":dbl)
    n769 = flat-sequence "To save data" {
      tunnel: [w3429] -> w1064
      tunnel: [w3430] -> w1063
      tunnel: w1004 -> [w3423]
      tunnel: w871 -> [w3427]
      tunnel: ["Save Calibration"] -> w1032
      tunnel: w1027 -> [w3426]
      tunnel: [w3419] -> w1026
      tunnel: [w3416] -> w1024
      tunnel: [w3413] -> w1023
      tunnel: w1003 -> [w3415]
      tunnel: w892 -> [w3408]
      tunnel: [w3408] -> w891
      tunnel: w1064 -> [w3616]
      tunnel: w1063 -> [w3615]
      tunnel: w1062 -> [w3614]
      tunnel: w1032 -> [w3613]
      tunnel: w1026 -> [w3611]
      tunnel: w1024 -> [w3610]
      tunnel: w1023 -> [w3609]
      tunnel: w855 -> [w3608]
      tunnel: w913 -> [w3607]
      tunnel: w891 -> [w3606]
      frame #0 {
        n770 = Or(x="Save N Sets", y="Start Saving") -> (x .or. y?=w3410:bool)
        n771 = To Double Precision Float(number=w3426) -> (double precision float=w3420:dbl)
        n772 = Build Array(w3410, "Save Calibration", w3423, w3415) -> (w3425:bool[])
        n773 = Compound Arithmetic op=OR("Save Calibration", w3423, w3410, w3415) -> (w3428:bool)
        n774 = Boolean Array To Number(Boolean array=w3425) -> (number=w3422:u32)
        n775 = feedback #21(refnum<k0> refnum) -> (w3431:refnum<file>)
        n776 = feedback #22(FALSE ("Save APD Data\nwith Trap Data")) -> (w3414:bool)
        n777 = feedback #23(refnum<k0> refnum) -> (w3417:refnum<file>)
        n778 = feedback #24(0) -> (w3433:i32)
        n779 = feedback #25() -> (w3421:u32)  [unwired: 1 out]
        n780 = case shown="True" w3428 {
          tunnel: [w3438 1] -> w3429
          tunnel: w3433 -> [w3440 _]
          tunnel: [w3439 w3453] -> w3430
          tunnel: w3431 -> [w3439 _]
          tunnel: w3427 -> [_ w3473]
          tunnel: w3420 -> [_ w3471]
          tunnel: w3422 -> [_ w3474]
          tunnel: [w3437 w3452] -> w3419
          tunnel: w3421 -> [w3437 _]
          tunnel: [w3436 w3449] -> w3416
          tunnel: w3417 -> [w3436 _]
          tunnel: [w3435 w3448] -> w3413
          tunnel: w3414 -> [w3435 _]
          tunnel: "Start Saving" -> [_ w3446]
          tunnel: w3408 -> [_ w3445]
          frame #0 {
            n781 = Increment(x=w3440) -> (x+1=w3438:i32)
          }
          frame #1 {
            w3441 = FALSE ("Start Saving")
            w3447 = 9.0  # File Version
            w3456 = FALSE ("prepend array or string size? (T)")
            w3454 = T31."big-endian, network order" ("byte order (0:big-endian, network order)")
            n782 = Array Size(array=w3445) -> (size(s)=w3444:i32)
            n783 = local read "BD 1 Frequency 1 (MHz)"() -> (w3470:dbl)
            n784 = local read "BD 2 Frequency 1 (MHz)"() -> (w3469:dbl)
            n785 = local read "BD 1 Frequency 2 (MHz)"() -> (w3468:dbl)
            n786 = local read "BD 2 Frequency 2 (MHz)"() -> (w3467:dbl)
            n787 = local read "BD 1 Frequency 3 (MHz)"() -> (w3466:dbl)
            n788 = local read "BD 2 Frequency 3 (MHz)"() -> (w3465:dbl)
            n789 = To Double Precision Float(number=w3444) -> (double precision float=w3443:dbl)
            n790 = local write "Start Saving"(w3441) -> ()
            n791 = local write "Save Calibration"(w3441) -> ()
            n792 = Build Array(w3470, w3469, w3468, w3467, w3466, w3465) -> (w3464:dbl[])
            n793 = case shown="2" w3474 {
              tunnel: w3473 -> [w3518 w3532 w3547 w3584]
              tunnel: w3443 -> [w3523 w3539 w3567 w3603]
              tunnel: w3471 -> [w3522 w3538 w3566 w3602]
              tunnel: [w3519 w3534 w3558 w3594] -> w3462
              tunnel: [w3508 "Cal sets to save" w3548 w3585] -> w3452
              tunnel: w3464 -> [w3520 w3535 w3560 w3596]
              tunnel: "Save APD Data\nwith Trap Data" -> [w3517 _ w3543 w3581]
              tunnel: [w3517 w3528 w3543 w3581] -> w3448
              tunnel: w3447 -> [w3511 w3526 w3541 w3579]
              tunnel: w3446 -> [w3510 _ _ _]
              frame #0 {
                w3514 = 0.0 ("f")
                # "timeseries"
                n794 = local read "Save ave N"() -> (w3525:dbl)
                n795 = Multiply(x=w3525, y=w3518) -> (x*y=w3524:dbl)
                n796 = Boolean To (0,1)(Boolean=w3517) -> (0, 1=w3516:i16)
                n797 = To Double Precision Float(number=w3516) -> (double precision float=w3515:dbl)
                n798 = Build Array(w3511, w3518, w3524, w3523, w3522, 0.0 ("f")) -> (w3521:dbl[])
                n799 = Build Array(w3515, w3514, w3514, w3514, w3514) -> (w3512:dbl[])
                n800 = Select(t=u32 4000000000, s=w3510, f="N sets to save") -> (s? t:f=w3508:u32)
                n801 = Build Array (concatenate)(w3521, w3520, w3512) -> (w3519:dbl[])
              }
              frame #1 {
                w3529 = 0.0 ("f")
                w3528 = FALSE ("Save APD Data\nwith Trap Data")
                # "calibration"
                n802 = Boolean To (0,1)(Boolean=w3528) -> (0, 1=w3531:i16)
                n803 = To Double Precision Float(number=w3531) -> (double precision float=w3530:dbl)
                n804 = Build Array(w3530, w3529, w3529, w3529, w3529) -> (w3527:dbl[])
                n805 = Build Array(w3526, w3532, w3532, w3539, w3538, 1.0 ("t")) -> (w3536:dbl[])
                n806 = Build Array (concatenate)(w3536, w3535, w3527) -> (w3534:dbl[])
                "Calibrating Trap..." <- TRUE ("Calibrating...")
              }
              frame #2 {
                w3544 = 0.0 ("f")
                # "scan dir (x/y = 0/1)"
                # "cycles/step"
                # "n scans (f/b)"
                # "steps"
                # "freq. range"
                # "AOD raster scan"
                n807 = local read "Number of F/B Scans (AOD)"() -> (w3552:u16)
                n808 = local read "Cycles/step (AOD)"() -> (w3554:u64)
                n809 = local read "Scan Range (MHz)"() -> (w3557:dbl)
                n810 = local read "Scan steps (AOD)"() -> (w3556:u64)
                n811 = local read "Scan BD"() -> (w3564:bool)
                n812 = local read "Save ave N"() -> (w3569:dbl)
                n813 = Boolean To (0,1)(Boolean=w3564) -> (0, 1=w3563:i16)
                n814 = To Double Precision Float(number=w3552) -> (double precision float=w3551:dbl)
                n815 = To Double Precision Float(number=w3556) -> (double precision float=w3555:dbl)
                n816 = To Double Precision Float(number=w3554) -> (double precision float=w3553:dbl)
                n817 = To Double Precision Float(number=w3563) -> (double precision float=w3562:dbl)
                n818 = Boolean To (0,1)(Boolean=w3543) -> (0, 1=w3546:i16)
                n819 = Multiply(x=w3569, y=w3547) -> (x*y=w3568:dbl)
                n820 = To Double Precision Float(number=w3546) -> (double precision float=w3545:dbl)
                n821 = Build Array(w3545, w3544, w3544, w3544, w3544) -> (w3542:dbl[])
                n822 = local read "N sets should be saved"() -> (w3549:dbl)
                n823 = Build Array(w3562, w3557, w3555, w3553, w3551) -> (w3559:dbl[])
                n824 = Build Array(w3541, w3547, w3568, w3567, w3566, 2.0 ("t")) -> (w3561:dbl[])
                n825 = Round Toward +Infinity(x=w3549) -> (ceil(x): smallest int >= x=w3550:dbl)
                n826 = Build Array (concatenate)(w3561, w3560, w3542, w3559) -> (w3558:dbl[])
                n827 = To Unsigned Long Integer(number=w3550) -> (unsigned 32bit integer=w3548:u32)
              }
              frame #3 {
                w3576 = 0.0 ("f")
                # "MCL raster scan"
                n828 = local read "Number of scans (MCL)"() -> (w3571:u64)
                n829 = local read "Scan lines (y)"() -> (w3570:u64)
                n830 = local read "2D or 1D Scan"() -> (w3573:bool)
                n831 = local read "Scan Range (V)\n(of steps)"() -> (w3593:dbl)
                n832 = local read "Fast Scan Dir"() -> (w3600:bool)
                n833 = local read "Cycles/step (MCL)"() -> (w3590:u64)
                n834 = Select(t=w3570, s=w3573, f=w3571) -> (s? t:f=w3572:u64)
                n835 = local read "Scan steps (MCL)"() -> (w3592:u64)
                n836 = Boolean To (0,1)(Boolean=w3573) -> (0, 1=w3575:i16)
                n837 = local read "Save ave N"() -> (w3605:dbl)
                n838 = local read "Initial X"() -> (w3578:dbl)
                n839 = local read "Initial Y"() -> (w3577:dbl)
                n840 = To Double Precision Float(number=w3575) -> (double precision float=w3574:dbl)
                n841 = Boolean To (0,1)(Boolean=w3600) -> (0, 1=w3599:i16)
                n842 = To Double Precision Float(number=w3572) -> (double precision float=w3588:dbl)
                n843 = To Double Precision Float(number=w3592) -> (double precision float=w3591:dbl)
                n844 = To Double Precision Float(number=w3590) -> (double precision float=w3589:dbl)
                n845 = To Double Precision Float(number=w3599) -> (double precision float=w3598:dbl)
                n846 = Boolean To (0,1)(Boolean=w3581) -> (0, 1=w3583:i16)
                n847 = Multiply(x=w3605, y=w3584) -> (x*y=w3604:dbl)
                n848 = To Double Precision Float(number=w3583) -> (double precision float=w3582:dbl)
                n849 = local read "N sets should be saved (MCL)"() -> (w3586:dbl)
                n850 = Build Array(w3582, w3574, w3576, w3576, w3576) -> (w3580:dbl[])
                n851 = Build Array(w3598, w3593, w3591, w3589, w3588, w3578, w3577) -> (w3595:dbl[])
                n852 = Build Array(w3579, w3584, w3604, w3603, w3602, 3.0 ("t")) -> (w3597:dbl[])
                n853 = Round Toward +Infinity(x=w3586) -> (ceil(x): smallest int >= x=w3587:dbl)
                n854 = Build Array (concatenate)(w3597, w3596, w3580, w3595) -> (w3594:dbl[])
                n855 = To Unsigned Long Integer(number=w3587) -> (unsigned 32bit integer=w3585:u32)
              }
            }
            n856 = local read "Index"() -> (w3479:dbl)
            n857 = call "Create new save file.vi"("Insert"="", "Ext"=".dat", "Index In"=w3479) -> ("Path Out"=w3450:path, "Index Out"=w3451:dbl)
            n858 = local write "Index"(w3451) -> ()
            n859 = local write "Save file name"(w3450) -> ()
            n860 = local write "Save index"(w3451) -> ()
            n861 = Array Size(array=w3462) -> (size(s)=w3463:i32)
            n862 = Open/Create/Replace File(file path (use dialog)=w3450, operation (0:open)=T30."create", access (0:read/write)=enum16{"read/write", "read-only", "write-only"}."write-only") -> (refnum out=w3476:refnum<file>)  [unwired: 1 in, 4 out]
            n863 = local write "Saving..."(TRUE ("Saving...")) -> ()
            n864 = To Double Precision Float(number=w3463) -> (double precision float=w3461:dbl)
            n865 = String Length(string="Comment (data description)") -> (length=w3459:i32)
            n866 = To Double Precision Float(number=w3459) -> (double precision float=w3458:dbl)
            n867 = Deny Access(7:w3476) -> (3:w3475:refnum<file>)  [unwired: 1 in, 2 out]
            n868 = Build Array (concatenate)(w3461, w3462, w3458) -> (w3460:dbl[])
            n869 = case "If fluorescence data to be saved" shown="True" w3448 {
              tunnel: w3450 -> [_ w3506]
              tunnel: [refnum<k0> refnum w3486] -> w3449
              frame #0 {
              }
              frame #1 {
                w3485 = 0.0
                n870 = local read "APD Integration Time (s)"() -> (w3491:dbl)
                n871 = local read "N APD Samp/step"() -> (w3484:dbl)
                n872 = Path To String(path=w3506) -> (string=w3505:string)
                n873 = String Length(string=w3505) -> (length=w3504:i32)
                n874 = Subtract(x=w3504, y=4) -> (x-y=w3502:i32)
                n875 = String Subset(string=w3505, length (rest)=w3502) -> (substring=w3501:string)  [unwired: 1 out]
                n876 = Build Array(w3491, w3484, w3485, w3485, w3485, w3485, w3485, w3485) -> (w3488:dbl[])
                n877 = Concatenate Strings(w3501, "_fl.dat" ("string")) -> (w3499:string)
                n878 = Array Size(array=w3488) -> (size(s)=w3490:i32)
                n879 = String To Path(string=w3499) -> (path=w3495:path)
                n880 = Open/Create/Replace File(file path (use dialog)=w3495, operation (0:open)=T30."create", access (0:read/write)=enum16{"read/write", "read-only", "write-only"}."write-only") -> (refnum out=w3496:refnum<file>)  [unwired: 1 in, 4 out]
                n881 = Deny Access(7:w3496) -> (3:w3492:refnum<file>)  [unwired: 1 in, 2 out]
                n882 = To Double Precision Float(number=w3490) -> (double precision float=w3489:dbl)
                n883 = Build Array (concatenate)(w3489, w3488) -> (w3487:dbl[])
                n884 = Write to Binary File(file (use dialog)=w3492, data=w3487, 5:FALSE ("prepend array or string size? (T)"), 9:T31."big-endian, network order" ("byte order (0:big-endian, network order)")) -> (refnum out=w3486:refnum<file>)  [unwired: 1 in, 3 out]
              }
            }
            n885 = Write to Binary File(file (use dialog)=w3475, data=w3460, 5:w3456, 9:w3454) -> (refnum out=w3457:refnum<file>)  [unwired: 1 in, 3 out]
            n886 = Write to Binary File(file (use dialog)=w3457, data="Comment (data description)", 5:w3456, 9:w3454) -> (refnum out=w3453:refnum<file>)  [unwired: 1 in, 3 out]
          }
        }
      }
      frame #1 {
        n887 = local read "Saving..."() -> (w3612:bool)
        n888 = case shown="True" w3612 {
          tunnel: w3616 -> [_ w3620]
          tunnel: w3615 -> [_ w3634]
          tunnel: w3614 -> [_ w3630]
          tunnel: w3613 -> [_ w3629]
          tunnel: w3611 -> [_ w3628]
          tunnel: w3610 -> [_ w3623]
          tunnel: w3609 -> [_ w3622]
          tunnel: w3608 -> [_ w3621]
          tunnel: w3607 -> [_ w3619]
          tunnel: w3606 -> [_ w3617]
          frame #0 {
          }
          frame #1 {
            n889 = Multiply(x=w3620, y=w3619) -> (x*y=→"Time (s)":dbl)
            n890 = Less Or Equal?(x=w3620, y=w3628) -> (x <= y?=w3632:bool)
            n891 = Or(x="Stop Saving", y="Abort save 2") -> (x .or. y?=w3624:bool)
            n892 = Not(x=w3624) -> (.not. x?=w3633:bool)
            n893 = And(x=w3632, y=w3633) -> (x .and. y?=w3631:bool)
            n894 = case shown="True" w3631 {
              tunnel: w3634 -> [w3639 w3655]
              tunnel: [0.0 w3658] -> w3627
              tunnel: w3620 -> [_ w3656]
              tunnel: w3628 -> [_ w3657]
              tunnel: w3630 -> [_ w3652]
              tunnel: w3629 -> [_ _]
              tunnel: w3623 -> [w3636 w3643]
              tunnel: w3622 -> [w3635 w3644]
              tunnel: w3621 -> [_ w3642]
              tunnel: w3617 -> [_ w3641]
              frame #0 {
                w3637 = FALSE
                n895 = Close File(refnum=w3639) -> ()  [unwired: 1 in, 2 out]
                n896 = case shown="True" w3635 {
                  tunnel: w3636 -> [_ w3640]
                  frame #0 {
                  }
                  frame #1 {
                    n897 = Close File(refnum=w3640) -> ()  [unwired: 1 in, 2 out]
                  }
                }
                n898 = local write "Raster Scanning..."(w3637) -> ()
                n899 = local write "Calibrating Trap..."(w3637) -> ()
                n900 = call <vilib>:"Beep.vi"() -> ()  [unwired: 3 in, 9 out]
                "Saving..." <- w3637
              }
              frame #1 {
                n901 = local read "Calibrating Trap..."() -> (w3645:bool)
                n902 = case shown="True" w3644 {
                  tunnel: w3643 -> [_ w3662]
                  tunnel: w3642 -> [_ w3661]
                  frame #0 {
                  }
                  frame #1 {
                    n903 = Write to Binary File(file (use dialog)=w3662, data=w3661, 5:FALSE ("prepend array or string size? (T)"), 9:T31."big-endian, network order" ("byte order (0:big-endian, network order)")) -> ()  [unwired: 1 in, 4 out]
                  }
                }
                n904 = Greater?(x="Save ave N", y=1.0) -> (0:w3648:bool)
                n905 = Not(x=w3645) -> (.not. x?=w3647:bool)
                n906 = And(x=w3647, y=w3648) -> (x .and. y?=w3649:bool)
                n907 = case shown="True" w3649 {
                  tunnel: w3652 -> [w3665 w3677]
                  tunnel: [w3665 w3668] -> w3646
                  tunnel: "Save ave N" -> [_ w3669]
                  tunnel: w3641 -> [_ w3667]
                  frame #0 {
                  }
                  frame #1 {
                    n908 = Array Size(array=w3677) -> (size(s)=w3670:i32)
                    n909 = Array Size(array=w3667) -> (size(s)=w3666:i32)
                    n910 = Divide(x=w3670, y=w3666) -> (x/y=w3675:dbl)
                    n911 = Reshape Array(w3677, w3675, w3666) -> (w3676:i16[][])
                    n912 = Transpose 2D Array(2D array=w3676) -> (transposed array=w3674:i16[][])
                    n913 = for {
                      tunnel: w3674 -> [w3680] mode=indexing
                      tunnel: [w3679] -> w3673 mode=indexing
                      tunnel: w3669 -> [w3678]
                      n914 = call "downsample 1D array - I16.vi"("Ave N"=w3678, "Array In"=w3680) -> ("Array Out"=w3679:i16[])  [unwired: 1 out]
                    }
                    n915 = Transpose 2D Array(2D array=w3673) -> (transposed array=w3672:i16[][])
                    n916 = Divide(x=w3670, y=w3669) -> (x/y=w3671:dbl)
                    n917 = Reshape Array(w3672, w3671) -> (w3668:i16[])
                  }
                }
                n918 = Write to Binary File(file (use dialog)=w3655, data=w3646, 5:FALSE ("prepend array or string size? (T)"), 9:T31."big-endian, network order" ("byte order (0:big-endian, network order)")) -> ()  [unwired: 1 in, 4 out]
                n919 = Divide(x=w3656, y=w3657) -> (x/y=w3659:dbl)
                n920 = Multiply(x=w3659, y=100.0) -> (x*y=w3658:dbl)
              }
            }
            "Progress" <- w3627
            "Progress 2" <- w3627
          }
        }
      }
    }
    n921 = local read "AI2 (V)"() -> (w1042:cluster{"Set 1":dbl, "Set 2":dbl})
    n922 = Bundle By Name(cluster=w1042, "Set 1"=w1041, "Set 2"=w1040) -> (w1038:cluster{"Set 1":dbl, "Set 2":dbl})
    n923 = Divide(x=w1038, y=3276.7) -> (x/y=w1037:cluster{"Set 1":dbl, "Set 2":dbl})
    n924 = local write "AI2 (V)"(w1037) -> ()
    n925 = Divide(x=w970, y=3276.7) -> (x/y=w966:T37)
    n926 = Unbundle By Name(w966) -> ("Green FB Ch 0"=w969:dbl, "Green FB Ch 1"=w968:dbl, "Green FB Ch 2"=w967:dbl)
    n927 = Divide(x=w969, y=w967) -> (x/y=w965:dbl)
    n928 = Divide(x=w968, y=w967) -> (x/y=w964:dbl)
    n929 = Bundle By Name(cluster=w966, "Green FB Ch 0"=w965, "Green FB Ch 1"=w964) -> (w944:T37)
    "Green FB Signals (V)" <- w944
    n930 = Unbundle By Name(w944) -> ("Green FB Ch 2"=→"Green FB Plot":dbl)
    n931 = local read "wait to reset values"() -> (w1046:bool)
    n932 = Not(x=w1043) -> (.not. x?=w1047:bool)
    n933 = And(x=w1047, y=w1046) -> (x .and. y?=w1048:bool)
    n934 = case "Part of MCL raster scanning: returns to initial positions after scan done" shown="True" w1048 {
      tunnel: w1051 -> [w2375 w2382]
      tunnel: [w2375 w2381] -> w1050
      tunnel: w1045 -> [w2374 w2380]
      tunnel: [w2374 w2379] -> w1044
      frame #0 {
      }
      frame #1 {
        w2390 = 10.0 ("y")
        w2389 = 32767.0 ("y")
        # "to return scan values\nafter a synchronous \nAOM scan"
        n935 = local read "AO2"() -> (w2383:dbl)
        n936 = local read "AO1"() -> (w2384:dbl)
        n937 = Multiply(x=w2384, y=w2389) -> (x*y=w2386:dbl)
        n938 = Multiply(x=w2383, y=w2389) -> (x*y=w2388:dbl)
        n939 = local write "wait to reset values"(FALSE ("wait to reset values")) -> ()
        n940 = Divide(x=w2386, y=w2390) -> (x/y=w2385:dbl)
        n941 = Divide(x=w2388, y=w2390) -> (x/y=w2387:dbl)
        n942 = To Word Integer(number=w2385) -> (16bit integer=w2391:i16)
        n943 = To Word Integer(number=w2387) -> (16bit integer=w2392:i16)
        n944 = local read "Total Counts (ticks)"() -> (w2376:u32)
        n945 = xnode "Read/Write Control"("FPGA VI Reference In"=w2382, "error in"=w2380, "AO1"=w2391, "AO2"=w2392, "MCL count"=w2376) -> ("FPGA VI Reference Out"=w2381:T15, "error out"=w2379:errorcluster)
        n946 = local read "Scan Range (V)\n(of steps)"() -> (w2377:dbl)
        n947 = property on="Scan Range (V)\n(of steps)" class="DigNum (strict)"("Val(Sgnl)"=w2377) -> ()  [unwired: 2 in, 2 out]
      }
    }
    n948 = node-c288() -> ()  [unwired: 2 out]
  }
  n949 = timed-loop "Oscillate AOD (debugging)" {
    tunnel: w76 -> [w3754]
    tunnel: [w3753] -> w16
    timing: w9 -> [_]
    timing-out: [_] -> w8
    stop <- w3753 stop-if-true
    n950 = node-c288() -> ()  [unwired: 2 out]
    n951 = event shown="[0] \"Oscillate Set 1\", \"Fish for Tether\": Value Change" {
      selector: _ -> [_ _ _]
      dyn-events: _ -> [_ _ _]
      timeout: _ -> [_ _ _]
      tunnel: w3754 -> [w3761 _ _]
      tunnel: [FALSE ("Stop All") _ w3944] -> w3753
      event #0 {
        n952 = event-data() -> ()  [unwired: 6 out]
        n953 = local read "Oscillate Set 1"() -> (w3760:bool)
        n954 = Or(x=w3760, y="Fish for Tether") -> (x .or. y?=w3758:bool)
        n955 = case shown="True" w3758 {
          tunnel: w3761 -> [_ w3763]
          tunnel: "Fish for Tether" -> [_ w3762]
          frame #0 {
          }
          frame #1 {
            n956 = case shown="True" w3762 {
              frame #0 {
              }
              frame #1 {
                n957 = local write "Scan axis 2"(TRUE) -> ()
                n958 = local write "Tether"(FALSE ("Tether")) -> ()
              }
            }
            n959 = node-c288() -> (w3765:T18)  [unwired: 4 out]
            n960 = timed-loop "Oscillate AOD" {
              timing: w3765 -> [_]
              timing-out: [_] -> w3764
              tunnel: w3763 -> [w3775]
              tunnel: w3762 -> [w3774]
              i -> [w3777]
              stop <- w3773 stop-if-true
              n961 = node-c288() -> (w3776:i64)  [unwired: 1 out]
              n962 = flat-sequence {
                tunnel: w3777 -> [w3804]
                tunnel: w3776 -> [w3803]
                tunnel: w3775 -> [w3782]
                tunnel: w3774 -> [w3785]
                tunnel: [w3785] -> w3772
                tunnel: [w3784] -> w3771
                tunnel: [w3781] -> w3770
                tunnel: [w3778] -> w3768
                tunnel: w3772 -> [w3840]
                tunnel: w3771 -> [w3838]
                tunnel: w3770 -> [w3837]
                tunnel: [w3836] -> w3769
                tunnel: w3768 -> [w3835]
                tunnel: [w3867] -> w3773
                tunnel: w3769 -> [w3866]
                frame #0 {
                  n963 = Divide(x=w3803, y=i64 1000) -> (x/y=w3798:dbl)
                  n964 = Multiply(x=w3798, y=w3804) -> (x*y=w3800:dbl)
                  n965 = local read "BD 1 Frequency 2 (MHz)"() -> (w3783:dbl)
                  n966 = Multiply(x="Osc. freq. (Hz)", y=6.283185307179586) -> (x*y=w3801:dbl)
                  n967 = Multiply(x=w3801, y=w3800) -> (x*y=w3780:dbl)
                  n968 = local read "BD 1 Frequency 1 (MHz)"() -> (w3788:dbl)
                  n969 = case shown="True" w3785 {
                    tunnel: w3780 -> [w3810 w3815]
                    tunnel: w3788 -> [_ w3826]
                    tunnel: w3783 -> [_ w3827]
                    tunnel: [w3807 w3821] -> w3786
                    tunnel: [FALSE w3818] -> w3781
                    tunnel: [0.0 w3811] -> w3778
                    frame #0 {
                      n970 = Sine(x=w3810) -> (sin(x)=w3808:dbl)
                      n971 = Multiply(x=w3808, y="Osc. amp. (MHz)") -> (x*y=w3807:dbl)
                    }
                    frame #1 {
                      n972 = Cosine(x=w3815) -> (cos(x)=w3830:dbl)
                      n973 = Subtract(x=w3827, y=w3826) -> (x-y=w3825:dbl)
                      n974 = Decrement(x=w3830) -> (x-1=w3829:dbl)
                      n975 = Subtract(x=w3825, y="Closest Delta (MHz)") -> (x-y=w3822:dbl)
                      n976 = Divide(x=w3829, y=-2.0) -> (x/y=w3823:dbl)
                      n977 = Multiply(x=w3823, y=w3822) -> (x*y=w3821:dbl)
                      n978 = local read "Vec Mean of T1 T2"() -> (w3817:dbl[])
                      n979 = Greater?(x=w3817, y="Stop F (pN)") -> (0:w3819:bool[])
                      n980 = Or Array Elements(Boolean array=w3819) -> (logical OR=w3818:bool)
                      n981 = Divide(x=w3815, y=6.283185307179586) -> (x/y=w3814:dbl)
                      n982 = Round Toward +Infinity(x=w3814) -> (ceil(x): smallest int >= x=w3811:dbl)
                      "Attempts" <- w3811
                      n983 = Greater?(x=w3811, y="Attempt Limit") -> (0:w3813:bool)
                      n984 = case shown="True" w3813 {
                        frame #0 {
                        }
                        frame #1 {
                          n985 = call <vilib>:"Beep.vi"() -> ()  [unwired: 3 in, 9 out]
                          n986 = local write "Fish for Tether"(FALSE ("Fish for Tether")) -> ()
                          n987 = local read "Messages"() -> (w3832:string)
                          n988 = call "Update messages.vi"("Message to add"="Tether fishing timeout." ("Messages"), "Old message string"=w3832) -> ("New message string"=→"Messages":string)
                        }
                      }
                    }
                  }
                  n989 = local read "BD 2 Frequency 1 (MHz)"() -> (w3787:dbl)
                  n990 = Select(t=w3788, s="Scan axis 2", f=w3787) -> (s? t:f=w3791:dbl)
                  n991 = Add(x=w3786, y=w3791) -> (x+y=w3784:dbl)
                  n992 = Select(t=w3784, s="Scan axis 2", f=w3788) -> (s? t:f=w3794:dbl)
                  n993 = Select(t=w3787, s="Scan axis 2", f=w3784) -> (s? t:f=w3793:dbl)
                  n994 = local read "Y RF Frequency Limits (MHz)"() -> (w3789:T12)
                  n995 = local read "X RF Frequency Limits (MHz)"() -> (w3790:T12)
                  n996 = local read "BD 1 Frequency 3 (MHz)"() -> (w3797:dbl)
                  n997 = local read "BD 2 Frequency 2 (MHz)"() -> (w3796:dbl)
                  n998 = local read "BD 2 Frequency 3 (MHz)"() -> (w3795:dbl)
                  n999 = call "set RF board frequency - interlace.vi"("Board 2 Frequency Limits"=w3789, "Board 1 Frequency Limits"=w3790, "FPGA VI Reference In"=w3782, "Board 2 Frequency 3 (MHz)"=w3795, "Board 1 Frequency 3 (MHz)"=w3797, "Board 2 Frequency 2 (MHz)"=w3796, "Board 2 Frequency 1 (MHz)"=w3793, "Board 1 Frequency 2 (MHz)"=w3783, "Board 1 Frequency 1  (MHz)"=w3794) -> ()  [unwired: 1 in, 2 out]
                }
                frame #1 {
                  n1000 = And(x=w3840, y=w3837) -> (x .and. y?=w3839:bool)
                  n1001 = case "Only if were fishing and now formed tether" shown="True" w3839 {
                    tunnel: w3838 -> [w3842 w3855]
                    tunnel: [w3841 w3854] -> w3836
                    tunnel: w3835 -> [_ w3850]
                    frame #0 {
                      n1002 = local read "Fish for Tether"() -> (w3841:bool)
                      n1003 = case shown="False" w3841 {
                        tunnel: w3842 -> [w3843 _]
                        frame #0 {
                          n1004 = property on="BD 1 Frequency 1 (MHz)" class="DigNum (strict)"("Val(Sgnl)"=w3843) -> ()  [unwired: 2 in, 2 out]
                        }
                        frame #1 {
                        }
                      }
                    }
                    frame #1 {
                      w3854 = FALSE ("Fish for Tether")
                      n1005 = call <vilib>:"Beep.vi"() -> ()  [unwired: 3 in, 9 out]
                      n1006 = Number To Decimal String(number=w3850, width (-)=i16 1) -> (decimal integer string=w3848:string)
                      n1007 = case shown="\"2\", \"3\"" "Then..." {
                        selector: "Then..." -> [_ w3858]
                        tunnel: w3855 -> [w3857 _]
                        frame #0 {
                          n1008 = property on="BD 1 Frequency 1 (MHz)" class="DigNum (strict)"("Val(Sgnl)"=w3857) -> ()  [unwired: 2 in, 2 out]
                        }
                        frame #1 {
                          n1009 = flat-sequence {
                            tunnel: w3858 -> [w3860]
                            frame #0 {
                              n1010 = property on="Trap Delta (MHz)" class="DigNum (strict)"("Val(Sgnl)"="Move to Delta (MHz)") -> ()  [unwired: 2 in, 2 out]
                            }
                            frame #1 {
                              n1011 = case shown="\"3\"" w3860 {
                                frame #0 {
                                n1012 = flat-sequence {
                                frame #0 {
                                n1013 = property on="Green Laser ON/Interlacing" class="Bool (strict)"("Val(Sgnl)"=TRUE ("Value (Signaling)")) -> ()  [unwired: 2 in, 2 out]
                                }
                                frame #1 {
                                n1014 = Multiply(x="Wait Before Save (s)", y=u32 1000 ("x")) -> (x*y=w3863:u32)
                                n1015 = Wait (ms)(milliseconds to wait=w3863) -> ()  [unwired: 1 out]
                                }
                                frame #2 {
                                n1016 = property on="Start Saving" class="Bool (strict)"("Value"=TRUE ("Start Saving")) -> ()  [unwired: 2 in, 2 out]
                                }
                                }
                                }
                                frame #1 {
                                }
                              }
                            }
                          }
                        }
                      }
                      n1017 = Concatenate Strings("Formed tether in ", w3848, " attempt(s)." ("string")) -> (w3845:string)
                      n1018 = local read "Messages"() -> (w3852:string)
                      n1019 = local write "Fish for Tether"(w3854) -> ()
                      n1020 = call "Update messages.vi"("Message to add"=w3845, "Old message string"=w3852) -> ("New message string"=w3851:string)
                      n1021 = local write "Messages"(w3851) -> ()
                      n1022 = Get Date/Time In Seconds() -> (seconds since 1Jan1904=→"Time tether formed":timestamp)
                      "Tether" <- "Tether Alarm?"
                    }
                  }
                }
                frame #2 {
                  n1023 = local read "Oscillate Set 1"() -> (w3871:bool)
                  n1024 = Or(x=w3871, y=w3866) -> (x .or. y?=w3868:bool)
                  n1025 = local read "Stop All"() -> (w3869:bool)
                  n1026 = Not(x=w3868) -> (.not. x?=w3870:bool)
                  n1027 = Compound Arithmetic op=OR(w3869, w3870) -> (w3867:bool)
                }
              }
              n1028 = node-c288() -> ()  [unwired: 2 out]
            }
            n1029 = node-c288(w3764) -> ()  [unwired: 1 out]
          }
        }
      }
      event #1 {
        n1030 = event-data() -> ()  [unwired: 7 out]
        n1031 = case shown="True" "Fl. Triggered..." {
          frame #0 {
          }
          frame #1 {
            n1032 = node-c288() -> (w3880:T18)  [unwired: 4 out]
            n1033 = timed-loop {
              timing: w3880 -> [_]
              timing-out: [_] -> w3879
              tunnel: "Action" -> [w3881]
              stop <- w3882 stop-if-true
              n1034 = node-c288() -> ()  [unwired: 2 out]
              n1035 = flat-sequence {
                tunnel: w3881 -> [w3885]
                tunnel: [w3935] -> w3882
                frame #0 {
                  n1036 = local read "APD 1 Rate (Hz)"() -> (w3888:dbl)
                  n1037 = Multiply(x="Fl. Threshold (kHz)", y=1000.0) -> (x*y=w3884:dbl)
                  n1038 = Greater?(x=w3888, y=w3884) -> (0:w3886:bool)
                  n1039 = case shown="True" w3886 {
                    tunnel: w3885 -> [_ w3891]
                    frame #0 {
                    }
                    frame #1 {
                      n1040 = flat-sequence {
                        tunnel: w3893 -> [w3896]
                        tunnel: [w3896] -> w3892
                        tunnel: w3891 -> [w3895]
                        tunnel: [w3895] -> w3890
                        tunnel: [w3894] -> w3889
                        tunnel: w3892 -> [w3903]
                        tunnel: w3890 -> [w3902]
                        tunnel: w3889 -> [w3901]
                        frame #0 {
                          n1041 = call <vilib>:"Beep.vi"() -> ()  [unwired: 3 in, 9 out]
                          n1042 = case shown="\"Alarm\", Default" w3895 {
                            frame #0 {
                              n1043 = property on="Confocal Image" class="Bool (strict)"("Val(Sgnl)"=TRUE ("Value (Signaling)")) -> ()  [unwired: 2 in, 2 out]
                            }
                            frame #1 {
                            }
                            frame #2 {
                              n1044 = property on="BD 1 Frequency 1 (MHz)" class="DigNum (strict)"("Val(Sgnl)"="Yank to Freq. (MHz)") -> ()  [unwired: 2 in, 2 out]
                            }
                          }
                          n1045 = local write "Waiting"(FALSE ("Waiting")) -> ()
                          n1046 = local read "Time (s)"() -> (w3894:dbl)
                          "Fl. High" <- TRUE ("Yanking")
                        }
                        frame #1 {
                          n1047 = node-c288() -> (w3905:T18)  [unwired: 4 out]
                          n1048 = timed-loop {
                            timing: w3905 -> [_]
                            timing-out: [_] -> w3904
                            tunnel: w3903 -> [w3915]
                            tunnel: w3902 -> [w3913]
                            tunnel: w3901 -> [w3912]
                            stop <- w3914 stop-if-true
                            n1049 = node-c288() -> ()  [unwired: 2 out]
                            n1050 = local read "Fl. Threshold (kHz)"() -> (w3907:dbl)
                            n1051 = local read "Fl. Triggered..."() -> (w3916:bool)
                            n1052 = local read "APD 1 Rate (Hz)"() -> (w3917:dbl)
                            n1053 = local read "Stop All"() -> (w3910:bool)
                            n1054 = Not(x=w3916) -> (.not. x?=w3911:bool)
                            n1055 = Multiply(x=w3907, y=1000.0) -> (x*y=w3908:dbl)
                            n1056 = Less?(x=w3917, y=w3908) -> (x < y?=w3909:bool)
                            n1057 = Compound Arithmetic op=OR(w3909, w3910, w3911) -> (w3914:bool)
                            n1058 = case shown="True" w3914 {
                              tunnel: w3915 -> [_ w3928]
                              tunnel: w3913 -> [_ w3927]
                              tunnel: w3912 -> [_ w3925]
                              frame #0 {
                              }
                              frame #1 {
                                n1059 = case shown="\"Yank\"" w3927 {
                                tunnel: w3928 -> [_ w3929]
                                frame #0 {
                                }
                                frame #1 {
                                n1060 = property on="BD 1 Frequency 1 (MHz)" class="DigNum (strict)"("Val(Sgnl)"=w3929) -> ()  [unwired: 2 in, 2 out]
                                }
                                }
                                n1061 = local read "Time (s)"() -> (w3926:dbl)
                                n1062 = Subtract(x=w3926, y=w3925) -> (x-y=w3922:dbl)
                                "Duration (s)" <- w3922
                                n1063 = Number To Decimal String(number=w3922, width (-)=i16 0) -> (decimal integer string=w3920:string)
                                n1064 = Concatenate Strings(w3920, " s fluorescence event." ("string")) -> (w3918:string)
                                n1065 = local read "Messages"() -> (w3924:string)
                                n1066 = call "Update messages.vi"("Message to add"=w3918, "Old message string"=w3924) -> ("New message string"=w3923:string)
                                n1067 = call <vilib>:"Beep.vi"() -> ()  [unwired: 3 in, 9 out]
                                n1068 = local write "Messages"(w3923) -> ()
                              }
                            }
                            n1069 = node-c288() -> ()  [unwired: 2 out]
                          }
                          n1070 = node-c288(w3904) -> ()  [unwired: 1 out]
                        }
                        frame #2 {
                          n1071 = local write "Fl. High"(FALSE ("Yanking")) -> ()
                        }
                      }
                      n1072 = local read "BD 1 Frequency 1 (MHz)"() -> (w3893:dbl)
                    }
                  }
                }
                frame #1 {
                  n1073 = local read "Stop All"() -> (w3938:bool)
                  n1074 = local read "Fl. Triggered..."() -> (w3936:bool)
                  n1075 = Not(x=w3936) -> (.not. x?=w3937:bool)
                  n1076 = Or(x=w3937, y=w3938) -> (x .or. y?=w3935:bool)
                  n1077 = Not(x=w3935) -> (.not. x?=→"Waiting":bool)
                }
              }
              n1078 = node-c288() -> ()  [unwired: 2 out]
            }
            n1079 = node-c288(w3879) -> ()  [unwired: 1 out]
          }
        }
      }
      event #2 {
        n1080 = event-data() -> ()  [unwired: 7 out]
        n1081 = local read "Stop All"() -> (w3944:bool)
      }
    }
    n1082 = node-c288() -> ()  [unwired: 2 out]
  }
  n1083 = timed-loop "Control parameters (event loop)" {
    tunnel: w76 -> [w3949]
    shift-right: [w3948] -> _
    shift-left: errorcluster {"status"=FALSE, "code"=0, "source"=""} ("error out") -> [w3947]
    tunnel: [w3946] -> w180
    timing: w11 -> [_]
    timing-out: [_] -> w10
    tunnel: w1 -> [w3945]
    stop <- w3946 stop-if-true
    n1084 = node-c288() -> ()  [unwired: 2 out]
    n1085 = event shown="[33] \"Scan steps (MCL)\", \"Number of scans (MCL)\", \"Scan Range (V)\n(of steps)\", \"2D or 1D Scan\", \"N APD Samp/step\", \"Fast Scan Dir\", \"Continuous MCL Scanning\", \"Scan lines (y)\": Value Change" {
      selector: _ -> [_ _ _ _ _ _ _ _ _ _ _ _ _ _ _ _ _ _ _ _ _ _ _ _ _ _ _ _ _ _ _ _ _ _ _ _ _ _ _ _ _ _ _ _ _]
      dyn-events: _ -> [_ _ _ _ _ _ _ _ _ _ _ _ _ _ _ _ _ _ _ _ _ _ _ _ _ _ _ _ _ _ _ _ _ _ _ _ _ _ _ _ _ _ _ _ _]
      timeout: _ -> [_ _ _ _ _ _ _ _ _ _ _ _ _ _ _ _ _ _ _ _ _ _ _ _ _ _ _ _ _ _ _ _ _ _ _ _ _ _ _ _ _ _ _ _ _]
      tunnel: w3949 -> [w3990 _ _ w4117 _ w4212 _ _ _ _ w4278 _ _ _ _ _ _ w4394 w4532 w4594 w4637 w4787 w4862 w4973 w5066 w5150 w5234 w5318 w5402 w5495 w5690 w5890 w5983 w6116 _ w6286 w6327 w6374 w6451 w6492 _ w6537 _ _ _]
      tunnel: [w3989 _ _ w4107 _ w4211 _ _ w4243 _ w4257 _ _ _ _ _ _ w4393 w4528 w4591 w4634 w4786 w4860 w4972 w5060 w5144 w5228 w5312 w5396 w5493 w5689 w5888 w5981 w6114 _ w6284 w6325 w6364 w6449 w6490 _ w6535 _ _ _] -> w3948
      tunnel: w3947 -> [w3988 _ _ w4116 _ w4210 _ _ w4243 _ w4277 _ _ _ _ _ _ w4392 w4527 w4590 w4633 w4785 w4861 w4971 w5065 w5149 w5233 w5317 w5401 w5494 w5688 w5889 w5982 w6115 _ w6285 w6326 w6373 w6450 w6491 _ w6536 _ _ _]
      tunnel: [_ _ _ _ _ _ _ _ w4242 _ _ _ _ _ _ _ _ _ _ _ _ _ _ _ _ _ _ _ _ _ _ _ _ _ _ _ _ _ _ _ _ _ _ _ _] -> w3946
      tunnel: [_ _ _ _ _ _ "Round T1 X" _ _ _ _ _ _ _ _ "Load parameters" _ _ _ _ _ _ _ _ _ _ _ _ _ _ _ _ _ _ _ _ _ _ _ _ _ _ _ _ _] -> _
      tunnel: [_ _ "Adjust Scale\nto Mean" _ _ _ _ _ _ _ _ "Set Position 1" "Set Position 2" "Set Position 3" "Set Position 4" _ _ _ _ _ _ _ _ _ _ _ _ _ _ _ _ _ _ _ _ _ _ _ _ _ _ _ _ _ _] -> _
      tunnel: [_ _ _ _ _ _ _ "Round T2 X" _ "Delayed Interlace Start" _ _ _ _ _ _ _ _ _ _ _ _ _ _ _ _ _ _ _ _ _ _ _ _ _ _ _ _ _ _ _ _ _ _ _] -> _
      tunnel: [_ "Rescale on Mean" _ _ _ _ _ _ _ _ _ _ _ _ _ _ _ _ _ _ _ _ _ _ _ _ _ _ _ _ _ _ _ _ _ _ _ _ _ _ _ _ _ _ _] -> _
      tunnel: w3945 -> [_ _ _ _ _ _ _ _ _ _ _ _ _ _ _ _ _ _ _ _ _ _ _ _ _ _ _ _ _ _ _ _ _ _ _ _ _ _ _ _ _ _ _ _ _]
      event #0 {
        # "So that if 'Save ave N' is updated, the AOD scanning code updates too."
        n1086 = event-data() -> ()  [unwired: 6 out]
        n1087 = local read "AI Count (ticks)"() -> (w3960:u32)
        n1088 = local read "FPGA Ave."() -> (w3964:dbl)
        n1089 = Boolean To (0,1)(Boolean="Sets to FIFO (Traps)") -> (0, 1=w3978:cluster{"Set 1":i16, "Set 2":i16, "Set 3":i16})
        n1090 = xnode "Read/Write Control"("FPGA VI Reference In"=w3990, "error in"=w3988, "ai count"=w3960, "AI1 Sets to FIFO"="Sets to FIFO (Traps)", "AI Averages"=w3964, "N of AI1 Int Acq Sets"="N Acq Sets (Traps)") -> ("error out"=w3989:errorcluster)  [unwired: 1 out]
        n1091 = Cluster To Array(cluster=w3978) -> (array=w3977:i16[])
        n1092 = local read "Scan steps (AOD)"() -> (w3979:u64)
        n1093 = Multiply(x=w3960, y="N Acq Sets (Traps)") -> (x*y=w3958:u32)
        n1094 = Divide(x=40000000.0, y=w3960) -> (x/y=w3986:dbl)
        "AI rate (Hz)" <- w3986
        n1095 = Add Array Elements(numeric array=w3977) -> (sum=w3962:i16)
        "Trap Sets" <- w3962
        n1096 = Divide(x=w3986, y=w3964) -> (x/y=w3987:dbl)
        "Ave. Rate (Hz)" <- w3987
        n1097 = Reciprocal(x=w3987) -> (1/x=→"Ave. Period (s)":dbl)
        n1098 = property on="Scan steps (AOD)" class="DigNum (strict)"("Val(Sgnl)"=w3979) -> ()  [unwired: 2 in, 2 out]
        n1099 = Divide(x=w3987, y="N Acq Sets (Traps)") -> (x/y=w3983:dbl)
        "Data Rate (Hz)" <- w3983
        n1100 = Reciprocal(x=w3983) -> (1/x=→"Data Period (s)":dbl)
        n1101 = local read "Save ave N"() -> (w3982:dbl)
        n1102 = Divide(x=w3983, y=w3982) -> (x/y=w3981:dbl)
        "Save Data Rate (Hz)" <- w3981
        n1103 = Reciprocal(x=w3981) -> (1/x=→"Save Data Period (s)":dbl)
        n1104 = Multiply(x=w3958, y="# Samples/trap") -> (x*y=w3954:dbl)
        "Counts/DMA" <- w3954
        n1105 = Multiply(x=w3962, y="# Samples/trap") -> (x*y=w3961:dbl)
        "# Samples/channel" <- w3961
        n1106 = Greater?(x=w3964, y=1.0) -> (0:w3967:bool)
        "FPGA Averaging" <- w3967
        n1107 = local read "APD Int. Count"() -> (w3956:u32)
        n1108 = Divide(x=w3961, y=u32 2) -> (x/y=w3970:dbl)
        n1109 = Select(t=w3961, s=w3967, f=w3970) -> (s? t:f=w3975:dbl)
        n1110 = Divide(x=w3954, y=w3956) -> (x/y=w3955:dbl)
        "APD Samples/FIFO Acq." <- w3955
        n1111 = Divide(x=w3954, y=40000000.0) -> (x/y=w3952:dbl)
        "DMA Update Period (s)" <- w3952
        n1112 = Multiply(x=w3975, y=u32 8) -> (x*y=→"Elements/DMA read":dbl)
        n1113 = Multiply(x=2.0, y=w3955) -> (x*y=→"APD Elements/DMA read":dbl)
        n1114 = local read "N sets to save"() -> (w3972:u32)
        n1115 = Multiply(x=w3952, y=w3972) -> (x*y=→"Total Time (s)":dbl)
      }
      event #1 {
        n1116 = event-data() -> ()  [unwired: 7 out]
        n1117 = local read "Bead Mean (nm)"() -> (w4095:dbl)
        n1118 = Add(x="Amplitude (nm)", y=w4095) -> (x+y=w4093:dbl)
        n1119 = Subtract(x=w4095, y="Amplitude (nm)") -> (x-y=w4092:dbl)
        n1120 = property on="Bead Separation" class="WFChart (strict)"("YScale.Maximum"=w4093) -> ()  [unwired: 2 in, 2 out]
        n1121 = property on="Bead Separation" class="WFChart (strict)"("YScale.Minimum"=w4092) -> ()  [unwired: 2 in, 2 out]
      }
      event #2 {
        n1122 = event-data() -> ()  [unwired: 7 out]
        n1123 = local read "APD 1 Rate (Hz)"() -> (w4104:dbl)
        n1124 = Multiply(x=1000.0, y="Above (kHz)") -> (x*y=w4102:dbl)
        n1125 = Multiply(x=1000.0, y="Below (kHz)") -> (x*y=w4100:dbl)
        n1126 = Add(x=w4102, y=w4104) -> (x+y=w4097:dbl)
        n1127 = Subtract(x=w4104, y=w4100) -> (x-y=w4098:dbl)
        n1128 = property on="APD 1 Chart" class="WFChart (strict)"("YScale.Maximum"=w4097) -> ()  [unwired: 2 in, 2 out]
        n1129 = property on="APD 1 Chart" class="WFChart (strict)"("YScale.Minimum"=w4098) -> ()  [unwired: 2 in, 2 out]
      }
      event #3 {
        n1130 = event-data() -> ()  [unwired: 7 out]
        n1131 = Negate(x="Phase adj. (AI1)") -> (-x=w4114:i16)
        n1132 = Select(t=w4114, s="- phase (AI1)", f="Phase adj. (AI1)") -> (s? t:f=w4113:i16)
        n1133 = xnode "Read/Write Control"("FPGA VI Reference In"=w4117, "error in"=w4116, "Phase count adjustment"=w4113) -> ("FPGA VI Reference Out"=w4112:T15, "error out"=w4111:errorcluster)
        n1134 = Or(x="- phase (AI1)", y="+ phase (AI1)") -> (x .or. y?=w4108:bool)
        n1135 = xnode "Read/Write Control"("FPGA VI Reference In"=w4112, "error in"=w4111, "+ phase"=w4108) -> ("error out"=w4107:errorcluster)  [unwired: 1 out]
      }
      event #4 {
        w4193 = u32 9868950 ("Color Box")
        n1136 = event-data() -> ("Row"=w4195:i32)  [unwired: 9 out]
        n1137 = property on="All Signals" class="WFChart (strict)"("Active Plot"=w4195) -> (error out=w4206:errorcluster)  [unwired: 2 in, 1 out]
        n1138 = property on="All Signals" class="WFChart (strict)" props=["Plot", "Visible?", "Plot", "Plot Color"](error in=w4206) -> (error out=w4205:errorcluster, "Plot.Visible?"=w4204:bool)  [unwired: 1 in, 2 out]
        n1139 = Select(t=FALSE ("Plot.Visible"), s=w4204, f=TRUE ("Plot.Visible")) -> (s? t:f=w4199:bool)
        n1140 = property on="All Signals" class="WFChart (strict)"(error in=w4205, "Plot.Visible?"=w4199) -> (error out=w4201:errorcluster)  [unwired: 1 in, 1 out]
        n1141 = property on="All Signals" class="WFChart (strict)"(error in=w4201) -> (error out=w4196:errorcluster, "Plot.Plot Color"=w4200:u32)  [unwired: 1 in, 1 out]
        n1142 = property on="Signals to Plot" class="LstBox (strict)"(error in=w4196, "Active Row"=w4195) -> (error out=w4194:errorcluster)  [unwired: 1 in, 1 out]
        n1143 = Select(t=w4200, s=w4199, f=u32 0) -> (s? t:f=w4197:u32)
        n1144 = property on="Signals to Plot" class="LstBox (strict)"(error in=w4194, "CellFontColor"=w4197, "SelColor"=w4193, "CellBG"=w4193, "CellFontSize"=u32 20 ("Active Row:Cell Font:Size"), "CellFontBold"=TRUE ("Active Row:Cell Font:Bold")) -> ()  [unwired: 1 in, 2 out]
      }
      event #5 {
        n1145 = event-data() -> ("CtlRef"=w4209:refnum<vi>)  [unwired: 6 out]
        n1146 = control-ref of="Trap Delta (MHz)"() -> (w4208:refnum<vi>)
        n1147 = Equal?(x=w4208, y=w4209) -> (x = y?=w4207:bool)
        n1148 = case shown="False" "Oscillate Set 1" {
          tunnel: w4212 -> [w4232 _]
          tunnel: [w4231 w4235] -> w4211
          tunnel: w4210 -> [w4230 w4235]
          tunnel: w4207 -> [w4215 _]
          frame #0 {
            n1149 = local read "BD 1 Frequency 2 (MHz)"() -> (w4219:dbl)
            n1150 = local read "BD 1 Frequency 1 (MHz)"() -> (w4217:dbl)
            n1151 = Subtract(x=w4219, y="Trap Delta (MHz)") -> (x-y=w4216:dbl)
            n1152 = Select(t=w4216, s=w4215, f=w4217) -> (s? t:f=w4214:dbl)
            n1153 = local read "Y RF Frequency Limits (MHz)"() -> (w4220:T12)
            n1154 = local read "X RF Frequency Limits (MHz)"() -> (w4221:T12)
            n1155 = local read "BD 1 Frequency 3 (MHz)"() -> (w4233:dbl)
            n1156 = local write "BD 1 Frequency 1 (MHz)"(w4214) -> ()
            n1157 = local read "BD 2 Frequency 1 (MHz)"() -> (w4224:dbl)
            n1158 = local read "BD 2 Frequency 2 (MHz)"() -> (w4223:dbl)
            n1159 = local read "BD 2 Frequency 3 (MHz)"() -> (w4234:dbl)
            n1160 = call "set RF board frequency - interlace.vi"("Board 2 Frequency Limits"=w4220, "Board 1 Frequency Limits"=w4221, "error in"=w4230, "FPGA VI Reference In"=w4232, "Board 2 Frequency 3 (MHz)"=w4234, "Board 1 Frequency 3 (MHz)"=w4233, "Board 2 Frequency 2 (MHz)"=w4223, "Board 2 Frequency 1 (MHz)"=w4224, "Board 1 Frequency 2 (MHz)"=w4219, "Board 1 Frequency 1  (MHz)"=w4214) -> ("error out"=w4231:errorcluster)  [unwired: 1 out]
            n1161 = Subtract(x=w4224, y=w4223) -> (x-y=w4228:dbl)
            n1162 = Subtract(x=w4214, y=w4219) -> (x-y=w4229:dbl)
            n1163 = Square(x=w4228) -> (x^2=w4226:dbl)
            n1164 = Square(x=w4229) -> (x^2=w4227:dbl)
            n1165 = Add(x=w4227, y=w4226) -> (x+y=w4225:dbl)
            n1166 = Square Root(x=w4225) -> (sqrt(x)=w4222:dbl)
            n1167 = local write "Trap Delta (MHz)"(w4222) -> ()
            n1168 = property on="Initial delta (MHz)" class="DigNum (strict)"("Val(Sgnl)"=w4222) -> ()  [unwired: 2 in, 2 out]
          }
          frame #1 {
          }
        }
      }
      event #6 {
        n1169 = event-data() -> ()  [unwired: 7 out]
        n1170 = local read "BD 1 Frequency 1 (MHz)"() -> (w4238:dbl)
        n1171 = Round To Nearest(number=w4238) -> (nearest integer value=w4237:dbl)
        n1172 = property on="BD 1 Frequency 1 (MHz)" class="DigNum (strict)"("Val(Sgnl)"=w4237) -> ()  [unwired: 2 in, 2 out]
      }
      event #7 {
        n1173 = event-data() -> ()  [unwired: 7 out]
        n1174 = local read "BD 1 Frequency 2 (MHz)"() -> (w4240:dbl)
        n1175 = Round To Nearest(number=w4240) -> (nearest integer value=w4239:dbl)
        n1176 = property on="BD 1 Frequency 2 (MHz)" class="DigNum (strict)"("Val(Sgnl)"=w4239) -> ()  [unwired: 2 in, 2 out]
      }
      event #8 {
        n1177 = event-data() -> ()  [unwired: 7 out]
        n1178 = local read "Stop All"() -> (w4242:bool)
      }
      event #9 {
        n1179 = event-data() -> ()  [unwired: 7 out]
        n1180 = flat-sequence {
          frame #0 {
            n1181 = Multiply(x="Delay to Interlace (s)", y=1000.0) -> (x*y=w4245:dbl)
            n1182 = Wait (ms)(milliseconds to wait=w4245) -> ()  [unwired: 1 out]
          }
          frame #1 {
            n1183 = property on="Green laser mode" class="RadioBtnsControl (strict)"("Val(Sgnl)"=enum32{"Laser ON", "Laser OFF", "Interlace"}."Interlace" ("Value (Signaling)")) -> ()  [unwired: 2 in, 2 out]
          }
        }
      }
      event #10 {
        w4269 = i16 1 ("f")
        n1184 = event-data() -> ()  [unwired: 7 out]
        n1185 = local write "Trap 1 (ON/OFF)"("Trap 1 ON") -> ()
        n1186 = local write "Trap 2 (ON/OFF)"("Trap 2 ON") -> ()
        n1187 = Boolean To (0,1)(Boolean="Trap 3 ON") -> (0, 1=w4270:i16)
        n1188 = Boolean To (0,1)(Boolean="Trap 1 ON") -> (0, 1=w4271:i16)
        n1189 = Boolean To (0,1)(Boolean="Trap 2 ON") -> (0, 1=w4272:i16)
        n1190 = Select(t=w4272, s="Trap ON/OFF X or Y Amp?", f=w4269) -> (s? t:f=w4267:i16)
        n1191 = Select(t=w4271, s="Trap ON/OFF X or Y Amp?", f=w4269) -> (s? t:f=w4268:i16)
        n1192 = Select(t=w4270, s="Trap ON/OFF X or Y Amp?", f=w4269) -> (s? t:f=w4266:i16)
        n1193 = Select(t=w4269, s="Trap ON/OFF X or Y Amp?", f=w4272) -> (s? t:f=w4264:i16)
        n1194 = Select(t=w4269, s="Trap ON/OFF X or Y Amp?", f=w4271) -> (s? t:f=w4265:i16)
        n1195 = Select(t=w4269, s="Trap ON/OFF X or Y Amp?", f=w4270) -> (s? t:f=w4263:i16)
        n1196 = And(x="All FB On/Off", y="Feedback On/Off") -> (x .and. y?=w4261:cluster{"Set 1":bool, "Set 2":bool})
        n1197 = local read "BD 1 Amplitude 1 (%)"() -> (w4281:dbl)
        n1198 = local read "BD 1 Amplitude 2 (%)"() -> (w4280:dbl)
        n1199 = local read "BD 1 Amplitude 3 (%)"() -> (w4279:dbl)
        n1200 = Unbundle By Name(w4261) -> ("Set 1"=w4256:bool, "Set 2"=w4253:bool)
        n1201 = local read "Y RF Amplitude Limits (%)"() -> (w4249:T12)
        n1202 = local read "X RF Amplitude Limits (%)"() -> (w4250:T12)
        n1203 = local read "BD 2 Amplitude 1 (%)"() -> (w4282:dbl)
        n1204 = local read "BD 2 Amplitude 2 (%)"() -> (w4283:dbl)
        n1205 = local read "BD 2 Amplitude 3 (%)"() -> (w4284:dbl)
        n1206 = And(x="Trap 2 ON", y=w4253) -> (x .and. y?=w4251:bool)
        n1207 = And(x="Trap 1 ON", y=w4256) -> (x .and. y?=w4254:bool)
        n1208 = Multiply(x=w4268, y=w4281) -> (x*y=w4276:dbl)
        n1209 = Multiply(x=w4280, y=w4267) -> (x*y=w4274:dbl)
        n1210 = Multiply(x=w4279, y=w4266) -> (x*y=w4275:dbl)
        n1211 = Multiply(x=w4282, y=w4265) -> (x*y=w4285:dbl)
        n1212 = Multiply(x=w4283, y=w4264) -> (x*y=w4286:dbl)
        n1213 = Multiply(x=w4284, y=w4263) -> (x*y=w4287:dbl)
        n1214 = call "set RF board amplitude - interlace.vi"("Board 2 Amplitude Limits"=w4249, "Board 1 Amplitude Limits"=w4250, "error in"=w4277, "FPGA VI Reference In"=w4278, "Board 2 Amplitude 3 (%)"=w4287, "Board 1 Amplitude 3 (%)"=w4275, "Board 2 Amplitude 2 (%)"=w4286, "Board 2 Amplitude 1 (%)"=w4285, "Board 1 Amplitude 2 (%)"=w4274, "Board 1 Amplitude 1 (%)"=w4276) -> ("error out"=w4258:errorcluster, "FPGA VI Reference Out"=w4259:T15)
        n1215 = xnode "Read/Write Control"("FPGA VI Reference In"=w4259, "error in"=w4258, "FB On/Off Set 1"=w4254, "FB On/Off Set 2"=w4251) -> ("error out"=w4257:errorcluster)  [unwired: 1 out]
      }
      event #11 {
        n1216 = event-data() -> ()  [unwired: 7 out]
        n1217 = local read "Current Stage  Position"() -> (w4348:cluster{dbl, dbl, dbl})
        n1218 = local read "Saved Stage Positions"() -> (w4347:T4)
        n1219 = Bundle By Name(cluster=w4347, "Position 1"=w4348) -> (w4346:T4)
        n1220 = local write "Saved Stage Positions"(w4346) -> ()
      }
      event #12 {
        n1221 = event-data() -> ()  [unwired: 7 out]
        n1222 = local read "Current Stage  Position"() -> (w4352:cluster{dbl, dbl, dbl})
        n1223 = local read "Saved Stage Positions"() -> (w4351:T4)
        n1224 = Bundle By Name(cluster=w4351, "Position 2"=w4352) -> (w4350:T4)
        n1225 = local write "Saved Stage Positions"(w4350) -> ()
      }
      event #13 {
        n1226 = event-data() -> ()  [unwired: 7 out]
        n1227 = local read "Saved Stage Positions"() -> (w4356:T4)
        n1228 = local read "Current Stage  Position"() -> (w4355:cluster{dbl, dbl, dbl})
        n1229 = Bundle By Name(cluster=w4356, "Position 3"=w4355) -> (w4354:T4)
        n1230 = local write "Saved Stage Positions"(w4354) -> ()
      }
      event #14 {
        n1231 = event-data() -> ()  [unwired: 7 out]
        n1232 = local read "Current Stage  Position"() -> (w4359:cluster{dbl, dbl, dbl})
        n1233 = local read "Saved Stage Positions"() -> (w4360:T4)
        n1234 = Bundle By Name(cluster=w4360, "Position 4"=w4359) -> (w4358:T4)
        n1235 = local write "Saved Stage Positions"(w4358) -> ()
      }
      event #15 {
        n1236 = event-data() -> ()  [unwired: 7 out]
        n1237 = property on="Saved AOD Raster Scan Parameter Sets" class="Arr (strict)"() -> ("Index Values"=w4370:u32[])  [unwired: 2 in, 2 out]
        n1238 = Index Array(array=w4370, index=0) -> (element=w4367:u32)
        n1239 = Index Array(array="Saved AOD Raster Scan Parameter Sets", index=w4367) -> (element=w4366:T38)
        n1240 = Unbundle By Name(w4366) -> ("Scan Range AOD (nm) 2"=w4365:dbl, "Step Size AOD (nm) 2"=w4364:dbl, "Scan Speed AOD (nm/s) 2"=w4363:dbl, "Number of scans (AOD) 2"=w4362:u16)
        n1241 = flat-sequence {
          tunnel: w4365 -> [w4374]
          tunnel: w4364 -> [w4373]
          tunnel: w4363 -> [w4372]
          tunnel: w4362 -> [w4375]
          frame #0 {
            n1242 = local write "Scan Speed (nm/s)"(w4372) -> ()
            n1243 = local write "Scan Range (nm)"(w4374) -> ()
            n1244 = local write "Step Size (nm)"(w4373) -> ()
          }
          frame #1 {
            n1245 = property on="Number of F/B Scans (AOD)" class="DigNum (strict)"("Val(Sgnl)"=w4375) -> ()  [unwired: 2 in, 2 out]
          }
        }
      }
      event #16 {
        n1246 = event-data() -> ()  [unwired: 7 out]
        n1247 = property on="Trap 2 ON" class="Bool (strict)"("Val(Sgnl)"="Trap 2 (ON/OFF)") -> ()  [unwired: 2 in, 2 out]
        n1248 = property on="Trap 1 ON" class="Bool (strict)"("Val(Sgnl)"="Trap 1 (ON/OFF)") -> ()  [unwired: 2 in, 2 out]
      }
      event #17 {
        n1249 = event-data() -> ()  [unwired: 7 out]
        n1250 = local read "DIO count 3 (ticks)"() -> (w4388:u32)
        n1251 = local read "DIO count 1 (ticks)"() -> (w4390:u32)
        n1252 = local read "DIO count 2 (ticks)"() -> (w4389:u32)
        n1253 = To Unsigned Byte Integer(number="Not-Interlacing Set") -> (unsigned 8bit integer=w4379:u8)
        n1254 = Add(x=w4379, y=u8 1) -> (x+y=w4383:u8)
        n1255 = xnode "Read/Write Control"("FPGA VI Reference In"=w4394, "error in"=w4392, "DIO count 1 (ticks)"=w4390, "DIO count 2 (ticks)"=w4389, "DIO count 3 (ticks)"=w4388, "Interlace ON/OFF"="Interlace", "Number Interlace Cycles"="Number Interlace Sets", "Interlace Off Parameters"=w4383) -> ("error out"=w4393:errorcluster)  [unwired: 1 out]
        n1256 = Build Array(w4390, w4389, w4388) -> (w4381:u32[])
        n1257 = Split 1D Array(array=w4381, index="Number Interlace Sets") -> (first subarray=w4391:u32[])  [unwired: 1 out]
        n1258 = Index Array(array=w4381, index=w4379) -> (element=w4380:u32)
        n1259 = Add Array Elements(numeric array=w4391) -> (sum=w4385:u32)
        n1260 = Select(t=w4385, s="Interlace", f=w4380) -> (s? t:f=→"Total Counts (ticks)":u32)
      }
      event #18 {
        n1261 = event-data() -> ()  [unwired: 7 out]
        n1262 = Unbundle By Name("Reset Feedback") -> ("Set 1"=w4530:bool, "Set 2"=w4529:bool)
        n1263 = xnode "Read/Write Control"("FPGA VI Reference In"=w4532, "error in"=w4527, "FB Reset Set 1"=w4530, "FB Reset Set 2"=w4529) -> ("error out"=w4528:errorcluster)  [unwired: 1 out]
      }
      event #19 {
        n1264 = event-data() -> ()  [unwired: 7 out]
        n1265 = Unbundle By Name("PID Gains") -> ("Set 1"=w4593:T10, "Set 2"=w4592:T10)
        n1266 = xnode "Read/Write Control"("FPGA VI Reference In"=w4594, "error in"=w4590, "FB Gains Set 1"=w4593, "FB Gains Set 2"=w4592) -> ("error out"=w4591:errorcluster)  [unwired: 1 out]
      }
      event #20 {
        n1267 = event-data() -> ()  [unwired: 7 out]
        n1268 = xnode "Read/Write Control"("FPGA VI Reference In"=w4637, "error in"=w4633) -> ("FPGA VI Reference Out"=w4636:T15, "error out"=w4635:errorcluster, "AI2 Y Sum Set 1"=w4644:i16, "AI2 Y Sum Set 2"=w4643:i16)
        n1269 = Cluster To Array(cluster="AI2 to Setpoint") -> (array=w4647:bool[])
        n1270 = local read "AI2 (V)"() -> (w4645:cluster{"Set 1":dbl, "Set 2":dbl})
        n1271 = Or Array Elements(Boolean array=w4647) -> (logical OR=w4648:bool)
        n1272 = Bundle By Name(cluster=w4645, "Set 1"=w4644, "Set 2"=w4643) -> (w4642:cluster{"Set 1":dbl, "Set 2":dbl})
        n1273 = Divide(x=w4642, y=3276.7) -> (x/y=w4641:cluster{"Set 1":dbl, "Set 2":dbl})
        "AI2 (V)" <- w4641
        n1274 = case shown="True" w4648 {
          tunnel: [w4710 w4727] -> w4640
          tunnel: "AI2 to Setpoint" -> [_ w4723]
          tunnel: "Setpoints (V)" -> [w4711 w4726]
          tunnel: w4641 -> [_ w4720]
          frame #0 {
            n1275 = Multiply(x=3276.7, y=w4711) -> (x*y=w4712:cluster{"Set 1":dbl, "Set 2":dbl})
            n1276 = To Word Integer(number=w4712) -> (16bit integer=w4710:cluster{"Set 1":i16, "Set 2":i16})
          }
          frame #1 {
            n1277 = Unbundle By Name(w4720) -> ("Set 1"=w4719:dbl, "Set 2"=w4718:dbl)
            n1278 = Unbundle By Name(w4726) -> ("Set 1"=w4725:dbl, "Set 2"=w4724:dbl)
            n1279 = Unbundle By Name(w4723) -> ("Set 1"=w4722:bool, "Set 2"=w4721:bool)
            n1280 = Select(t=w4719, s=w4722, f=w4725) -> (s? t:f=w4717:dbl)
            n1281 = Select(t=w4718, s=w4721, f=w4724) -> (s? t:f=w4716:dbl)
            n1282 = Bundle By Name(cluster=w4726, "Set 1"=w4717, "Set 2"=w4716) -> (w4714:cluster{"Set 1":dbl, "Set 2":dbl})
            n1283 = Multiply(x=3276.7, y=w4714) -> (x*y=w4715:cluster{"Set 1":dbl, "Set 2":dbl})
            n1284 = local write "Setpoints (V)"(w4714) -> ()
            n1285 = To Word Integer(number=w4715) -> (16bit integer=w4727:cluster{"Set 1":i16, "Set 2":i16})
          }
        }
        n1286 = Unbundle By Name(w4640) -> ("Set 1"=w4639:i16, "Set 2"=w4638:i16)
        n1287 = xnode "Read/Write Control"("FPGA VI Reference In"=w4636, "error in"=w4635, "FB Setpoint Set 1"=w4639, "FB Setpoint Set 2"=w4638) -> ("error out"=w4634:errorcluster)  [unwired: 1 out]
      }
      event #21 {
        n1288 = event-data() -> ()  [unwired: 7 out]
        n1289 = xnode "Read/Write Control"("FPGA VI Reference In"=w4787, "error in"=w4785, "Invert GI"="Invert GI", "Invert GI 2"="Invert GI") -> ("error out"=w4786:errorcluster)  [unwired: 1 out]
      }
      event #22 {
        n1290 = event-data() -> ()  [unwired: 7 out]
        n1291 = local read "Green FB Setpoint (mV)"() -> (w4851:dbl)
        n1292 = local read "Current When FB OFF (%)"() -> (w4854:dbl)
        n1293 = Multiply(x=w4851, y=3.2767) -> (x*y=w4850:dbl)
        n1294 = Multiply(x=w4854, y=655.35) -> (x*y=w4855:dbl)
        n1295 = To Unsigned Word Integer(number=w4855) -> (unsigned 16bit integer=w4853:u16)
        n1296 = local read "Green int current ON count adj"() -> (w4858:u32)
        n1297 = local read "Green FB Gains"() -> (w4857:T10)
        n1298 = local read "Green Laser ON/Interlacing"() -> (w4848:bool)
        n1299 = local read "Green laser mode"() -> (w4847:enum32{"Laser ON", "Laser OFF", "Interlace"})
        n1300 = local read "Green FB On/Off"() -> (w4859:bool)
        n1301 = Equal?(x=w4847, y=enum32{"Laser ON", "Laser OFF", "Interlace"}."Interlace") -> (x = y?=w4845:bool)
        n1302 = Compound Arithmetic op=AND(w4845, w4859, w4848) -> (w4849:bool)
        n1303 = xnode "Read/Write Control"("FPGA VI Reference In"=w4862, "error in"=w4861, "Green FB Setpoint"=w4850, "Green FB On/Off"=w4849, "Current Out"=w4853, "Green int current ON count adj"=w4858, "Green FB Gains"=w4857) -> ("error out"=w4860:errorcluster)  [unwired: 1 out]
      }
      event #23 {
        n1304 = event-data() -> ()  [unwired: 7 out]
        n1305 = case shown="True" "Green Laser ON/Interlacing" {
          tunnel: "Green laser mode" -> [_ w4980]
          tunnel: [enum32{"Laser ON", "Laser OFF", "Interlace"}."Laser OFF" ("Green laser mode") w4980] -> w4968
          tunnel: [FALSE w4976] -> w4967
          frame #0 {
          }
          frame #1 {
            n1306 = local read "Green FB On/Off"() -> (w4977:bool)
            n1307 = Equal?(x=w4980, y=enum32{"Laser ON", "Laser OFF", "Interlace"}."Interlace") -> (x = y?=w4978:bool)
            n1308 = And(x=w4978, y=w4977) -> (x .and. y?=w4976:bool)
          }
        }
        n1309 = xnode "Read/Write Control"("FPGA VI Reference In"=w4973, "error in"=w4971, "Operating Mode"=w4968, "Operating Mode 2"=w4968, "Green FB On/Off"=w4967) -> ("error out"=w4972:errorcluster)  [unwired: 1 out]
      }
      event #24 {
        n1310 = event-data() -> ()  [unwired: 7 out]
        n1311 = local read "Phase Adj. (APD Gate)"() -> (w5056:i16)
        n1312 = Negate(x=w5056) -> (-x=w5064:i16)
        n1313 = Select(t=w5064, s="- phase (APD Gate)", f=w5056) -> (s? t:f=w5063:i16)
        n1314 = Or(x="- phase (APD Gate)", y="+ phase (APD Gate)") -> (x .or. y?=w5059:bool)
        n1315 = xnode "Read/Write Control"("FPGA VI Reference In"=w5066, "error in"=w5065, "Phase count adjustment (APD Gate)"=w5063) -> ("FPGA VI Reference Out"=w5061:T15, "error out"=w5062:errorcluster)
        n1316 = xnode "Read/Write Control"("FPGA VI Reference In"=w5061, "error in"=w5062, "+ phase (APD Gate)"=w5059) -> ("error out"=w5060:errorcluster)  [unwired: 1 out]
      }
      event #25 {
        n1317 = event-data() -> ()  [unwired: 7 out]
        n1318 = local read "Phase Adj. (APD Acq)"() -> (w5142:i16)
        n1319 = Negate(x=w5142) -> (-x=w5148:i16)
        n1320 = Select(t=w5148, s="+ phase (APD Acq)", f=w5142) -> (s? t:f=w5147:i16)
        n1321 = Or(x="+ phase (APD Acq)", y="- phase (APD Acq)") -> (x .or. y?=w5143:bool)
        n1322 = xnode "Read/Write Control"("FPGA VI Reference In"=w5150, "error in"=w5149, "Phase Count Adjustment (APD Acq)"=w5147) -> ("FPGA VI Reference Out"=w5145:T15, "error out"=w5146:errorcluster)
        n1323 = xnode "Read/Write Control"("FPGA VI Reference In"=w5145, "error in"=w5146, "+ phase (APD Acq)"=w5143) -> ("error out"=w5144:errorcluster)  [unwired: 1 out]
      }
      event #26 {
        n1324 = event-data() -> ()  [unwired: 7 out]
        n1325 = Negate(x="Phase adj. (GI)") -> (-x=w5232:i16)
        n1326 = Select(t=w5232, s="+ phase (GI)", f="Phase adj. (GI)") -> (s? t:f=w5231:i16)
        n1327 = Or(x="+ phase (GI)", y="- phase (GI)") -> (x .or. y?=w5227:bool)
        n1328 = xnode "Read/Write Control"("FPGA VI Reference In"=w5234, "error in"=w5233, "Phase count adjustment (GI)"=w5231) -> ("FPGA VI Reference Out"=w5229:T15, "error out"=w5230:errorcluster)
        n1329 = xnode "Read/Write Control"("FPGA VI Reference In"=w5229, "error in"=w5230, "+ phase (GI)"=w5227) -> ("error out"=w5228:errorcluster)  [unwired: 1 out]
      }
      event #27 {
        n1330 = event-data() -> ()  [unwired: 7 out]
        n1331 = Negate(x="Phase adj. (GI) 2") -> (-x=w5316:i16)
        n1332 = Select(t=w5316, s="+ phase (GI) 2", f="Phase adj. (GI) 2") -> (s? t:f=w5315:i16)
        n1333 = Or(x="+ phase (GI) 2", y="- phase (GI) 2") -> (x .or. y?=w5311:bool)
        n1334 = xnode "Read/Write Control"("FPGA VI Reference In"=w5318, "error in"=w5317, "Phase count adjustment (GI) 2"=w5315) -> ("FPGA VI Reference Out"=w5313:T15, "error out"=w5314:errorcluster)
        n1335 = xnode "Read/Write Control"("FPGA VI Reference In"=w5313, "error in"=w5314, "+ phase (GI) 2"=w5311) -> ("error out"=w5312:errorcluster)  [unwired: 1 out]
      }
      event #28 {
        n1336 = event-data() -> ()  [unwired: 7 out]
        n1337 = Negate(x="Phase adj. (Green FB)") -> (-x=w5400:i16)
        n1338 = Select(t=w5400, s="+ phase (Green FB)", f="Phase adj. (Green FB)") -> (s? t:f=w5399:i16)
        n1339 = Or(x="+ phase (Green FB)", y="- phase (Green FB)") -> (x .or. y?=w5395:bool)
        n1340 = xnode "Read/Write Control"("FPGA VI Reference In"=w5402, "error in"=w5401, "Phase count adjustment (Green FB)"=w5399) -> ("FPGA VI Reference Out"=w5397:T15, "error out"=w5398:errorcluster)
        n1341 = xnode "Read/Write Control"("FPGA VI Reference In"=w5397, "error in"=w5398, "+ phase (Green FB)"=w5395) -> ("error out"=w5396:errorcluster)  [unwired: 1 out]
      }
      event #29 {
        n1342 = event-data() -> ()  [unwired: 7 out]
        n1343 = local read "Invert APD Gate"() -> (w5492:bool)
        n1344 = local read "APD Gate ON Count"() -> (w5491:u32)
        n1345 = local read "APD Gate OFF Count"() -> (w5490:u32)
        n1346 = local read "APD Integration Time (s)"() -> (w5476:dbl)
        n1347 = local read "APD Gate"() -> (w5489:enum32{"ON", "OFF", "Interlace"})
        n1348 = Multiply(x=w5476, y=40000000.0) -> (x*y=w5487:dbl)
        n1349 = Reciprocal(x=w5476) -> (1/x=→"APD Acq Rate (Hz)":dbl)
        n1350 = To Unsigned Long Integer(number=w5487) -> (unsigned 32bit integer=w5486:u32)
        n1351 = local read "DMA Update Period (s)"() -> (w5477:dbl)
        n1352 = Divide(x=w5477, y=w5476) -> (x/y=w5480:dbl)
        n1353 = local read "APD 1 AO offset"() -> (w5482:i16)
        n1354 = local read "APD 2 AO offset"() -> (w5481:i16)
        n1355 = local read "APD 1 AO Mult."() -> (w5484:i16)
        n1356 = local read "APD 2 AO Mult."() -> (w5483:i16)
        n1357 = Multiply(x=2.0, y=w5480) -> (x*y=w5479:dbl)
        n1358 = local write "APD Samples/FIFO Acq."(w5480) -> ()
        n1359 = local write "APD Elements/DMA read"(w5479) -> ()
        n1360 = xnode "Read/Write Control"("FPGA VI Reference In"=w5495, "error in"=w5494, "Invert APD Gate"=w5492, "APD Gate ON Count"=w5491, "APD Gate OFF Count"=w5490, "APD Acq Rate Count"=w5486, "APD Gate Operating Mode"=w5489, "APD 1 AO scale factor"=w5484, "APD 2 AO scale factor"=w5483, "APD 1 AO offset"=w5482, "APD 2 AO offset"=w5481) -> ("error out"=w5493:errorcluster)  [unwired: 1 out]
      }
      event #30 {
        n1361 = event-data() -> ()  [unwired: 7 out]
        n1362 = xnode "Read/Write Control"("FPGA VI Reference In"=w5690, "error in"=w5688, "Green interlace ON count"="GI Frequency, ON count", "Green interlace OFF count"="GI Frequency, OFF count", "Green interlace ON count 2"="GI Frequency, ON count", "Green interlace OFF count 2"="GI Frequency, OFF count", "Green FB Count"="Green FB Count") -> ("error out"=w5689:errorcluster)  [unwired: 1 out]
      }
      event #31 {
        w5858 = 123.0  # AOM cal (nm/MHz)
        n1363 = event-data() -> ()  [unwired: 7 out]
        n1364 = local read "BD 1 Frequency 1 (MHz)"() -> (w5841:dbl)
        n1365 = local read "BD 2 Frequency 1 (MHz)"() -> (w5847:dbl)
        n1366 = local read "X RF Frequency Limits (MHz)"() -> (w5845:T12)
        n1367 = local read "Y RF Frequency Limits (MHz)"() -> (w5842:T12)
        n1368 = local read "AOM X Cal (nm/MHz)"() -> (w5833:dbl)
        n1369 = Negate(x="Scan Range (nm)") -> (-x=w5810:dbl)
        n1370 = Divide(x=w5810, y=w5833) -> (x/y=w5814:dbl)
        n1371 = Select(t=w5845, s="Scan BD", f=w5842) -> (s? t:f=w5844:T12)
        n1372 = Select(t=w5841, s="Scan BD", f=w5847) -> (s? t:f=w5846:dbl)
        n1373 = Unbundle By Name(w5844) -> ("Maximum"=w5853:dbl, "Minimum"=w5852:dbl)
        n1374 = Add(x=w5814, y=w5846) -> (x+y=w5850:dbl)
        n1375 = Divide(x=w5810, y="Step Size (nm)") -> (x/y=w5830:dbl)
        n1376 = Divide(x="Step Size (nm)", y=w5833) -> (x/y=w5839:dbl)
        n1377 = Absolute Value(x=w5830) -> (abs(x)=w5813:dbl)
        n1378 = Sign(1:w5810) -> (0:w5811:dbl)
        n1379 = In Range and Coerce(upper limit=w5853, x=w5850, lower limit=w5852) -> (coerced(x)=w5849:dbl, In Range?=w5851:bool)
        n1380 = To Unsigned Quad Integer(1:w5813) -> (0:w5829:u64)
        "Scan steps (AOD)" <- w5829
        n1381 = call "IR AOM freq to word.vi"("Frequency In (MHz)"=w5839) -> ("Frequency Word Out (double)"=w5836:dbl)
        n1382 = Multiply(x=w5811, y=w5836) -> (x*y=w5812:dbl)
        n1383 = Subtract(x=w5850, y=w5849) -> (x-y=w5848:dbl)
        n1384 = To Quad Integer(1:w5812) -> (0:w5835:i64)
        "Incr. int (AOD)" <- w5835
        n1385 = Subtract(x=w5814, y=w5848) -> (x-y=w5834:dbl)
        "Scan Range (MHz)" <- w5834
        n1386 = Select(t=w5814, s=w5851, f=w5834) -> (s? t:f=w5854:dbl)
        n1387 = Multiply(x=w5834, y=w5833) -> (x*y=w5832:dbl)
        n1388 = Decrement(x=w5829) -> (x-1=w5882:u64)
        n1389 = Negate(x=w5832) -> (-x=w5828:dbl)
        n1390 = local write "Scan Range (nm)"(w5828) -> ()
        n1391 = Divide(x=w5854, y=w5882) -> (x/y=w5838:dbl)
        "Scan Increment (MHz)" <- w5838
        n1392 = call "IR AOM freq to word.vi"("Frequency In (MHz)"=w5838) -> ("Frequency Word Out (double)"=w5837:dbl)
        n1393 = Divide(x="Step Size (nm)", y="Scan Speed (nm/s)") -> (x/y=w5825:dbl)
        n1394 = To Quad Integer(1:w5837) -> ()  [unwired: 1 out]
        n1395 = local read "Number Interlace Sets"() -> (w5808:u8)
        n1396 = local read "AI Count (ticks)"() -> (w5809:u32)
        n1397 = local read "Total Counts (ticks)"() -> (w5807:u32)
        n1398 = local read "# Samples/trap"() -> (w5840:dbl)
        n1399 = Multiply(x=w5809, y=w5808) -> (x*y=w5806:u32)
        n1400 = Divide(x=w5807, y=w5806) -> (x/y=w5805:dbl)
        n1401 = Select(t=w5841, s="Scan BD", f=w5847) -> (s? t:f=w5879:dbl)
        "Initial freq. (MHz)" <- w5879
        n1402 = Add(x=w5854, y=w5879) -> (x+y=→"Final freq. (MHz)":dbl)
        n1403 = Divide(x=w5807, y=40000000.0) -> (x/y=w5824:dbl)
        n1404 = Divide(x=w5825, y=w5824) -> (x/y=w5823:dbl)
        n1405 = To Unsigned Quad Integer(1:w5823) -> (0:w5822:u64)
        "Cycles/step (AOD)" <- w5822
        n1406 = xnode "Read/Write Control"("FPGA VI Reference In"=w5890, "error in"=w5889, "Scan steps"=w5829, "Number of scans"="Number of F/B Scans (AOD)", "Cycles per step"=w5822, "Scan freq.  increment"=w5835, "Scan BD"="Scan BD") -> ("error out"=w5888:errorcluster)  [unwired: 1 out]
        n1407 = Multiply(x=w5829, y=w5822) -> (x*y=w5883:u64)
        n1408 = Multiply(x=w5883, y=u64 2) -> (x*y=w5804:u64)
        n1409 = Multiply(x=w5805, y=w5804) -> (x*y=w5803:dbl)
        "Data points/scan (f/b)" <- w5803
        n1410 = Multiply(x=w5803, y="Number of F/B Scans (AOD)") -> (x*y=w5886:dbl)
        "Data points/scans" <- w5886
        n1411 = Divide(x=w5886, y=w5840) -> (x/y=→"N sets should be saved":dbl)
        n1412 = Multiply(x=w5883, y=w5824) -> (x*y=w5821:dbl)
        "Time/Scan (s) (AOD)" <- w5821
        n1413 = Select(t=w5854, s="Scan BD", f=0.0) -> (s? t:f=w5880:dbl)
        n1414 = Select(t=0.0, s="Scan BD", f=w5854) -> (s? t:f=w5876:dbl)
        n1415 = local read "BD 2 Frequency 2 (MHz)"() -> (w5872:dbl)
        n1416 = local read "BD 1 Frequency 2 (MHz)"() -> (w5875:dbl)
        n1417 = Add(x=w5876, y=w5847) -> (x+y=w5873:dbl)
        n1418 = Add(x=w5841, y=w5880) -> (x+y=w5874:dbl)
        n1419 = Multiply(x=w5821, y=2.0) -> (x*y=w5820:dbl)
        n1420 = Multiply(x=w5820, y="Number of F/B Scans (AOD)") -> (x*y=w5817:dbl)
        n1421 = Divide(x=w5817, y=60.0) -> (x/y=→"Time to Finish All (min)":dbl)
        n1422 = Add(x="Trap 2 Bead Size (nm)", y="Trap 1 Bead Size (nm)") -> (x+y=w5862:dbl)
        n1423 = Divide(x=w5862, y=2.0) -> (x/y=w5856:dbl)
        n1424 = Subtract(x=w5873, y=w5872) -> (x-y=w5870:dbl)
        n1425 = Subtract(x=w5874, y=w5875) -> (x-y=w5871:dbl)
        n1426 = local read "Initial delta (MHz)"() -> (w5859:dbl)
        n1427 = Square(x=w5870) -> (x^2=w5869:dbl)
        n1428 = Square(x=w5871) -> (x^2=w5868:dbl)
        n1429 = Add(x=w5868, y=w5869) -> (x+y=w5867:dbl)
        n1430 = Square Root(x=w5867) -> (sqrt(x)=w5866:dbl)
        "Final delta (MHz)" <- w5866
        n1431 = Multiply(x=w5858, y=w5866) -> (x*y=w5865:dbl)
        n1432 = Multiply(x=w5859, y=w5858) -> (x*y=w5857:dbl)
        n1433 = Subtract(x=w5857, y=w5856) -> (x-y=→"Initial sep (nm)":dbl)
        n1434 = Subtract(x=w5865, y=w5856) -> (x-y=→"Final sep (nm)":dbl)
      }
      event #32 {
        n1435 = event-data() -> ()  [unwired: 7 out]
        n1436 = local read "Freq or Amp switch first"() -> (w5977:bool)
        n1437 = local read "Freq switch delay"() -> (w5980:u16)
        n1438 = local read "Amp switch delay"() -> (w5978:u16)
        n1439 = local read "Swap F1 and F2"() -> (w5979:bool)
        n1440 = xnode "Read/Write Control"("FPGA VI Reference In"=w5983, "error in"=w5982, "Freq switch delay"=w5980, "Swap F1 and F2"=w5979, "Amp switch delay"=w5978, "Freq or Amp switch first"=w5977) -> ("error out"=w5981:errorcluster)  [unwired: 1 out]
      }
      event #33 {
        w6080 = 32767.0 ("y")
        n1441 = event-data() -> ()  [unwired: 7 out]
        n1442 = Select(t="Scan lines (y)", s="2D or 1D Scan", f="Number of scans (MCL)") -> (s? t:f=w6085:u64)
        n1443 = Decrement(x="Scan steps (MCL)") -> (x-1=w6101:u64)
        n1444 = Divide(x="Scan Range (V)\n(of steps)", y=w6101) -> (x/y=w6100:dbl)
        "Desired Scan Incr (V)" <- w6100
        n1445 = local read "APD Integration Time (s)"() -> (w6093:dbl)
        n1446 = Multiply(x=w6100, y=w6080) -> (x*y=w6109:dbl)
        n1447 = Divide(x=w6109, y=10.0) -> (x/y=w6099:dbl)
        "Desired incr (int)" <- w6099
        n1448 = local read "Update Count (MCL)"() -> (w6105:u32)
        n1449 = Round Toward -Infinity(1:w6099) -> (0:w6108:dbl)
        n1450 = To Word Integer(number=w6108) -> (16bit integer=w6083:i16)
        "Actual Incr. int (MCL)" <- w6083
        n1451 = Multiply(x=w6093, y=40000000.0) -> (x*y=w6106:dbl)
        n1452 = Divide(x=w6106, y=w6105) -> (x/y=w6104:dbl)
        n1453 = Multiply(x=i16 10, y=w6083) -> (x*y=w6081:i16)
        n1454 = Multiply(x="N APD Samp/step", y=w6104) -> (x*y=w6103:dbl)
        "Cycles/step (MCL)" <- w6103
        n1455 = Divide(x=w6081, y=w6080) -> (x/y=→"Actual MCL Inc (V)":dbl)
        n1456 = Multiply(x="N APD Samp/step", y="Scan steps (MCL)") -> (x*y=w6095:dbl)
        n1457 = local read "APD Samples/FIFO Acq."() -> (w6092:dbl)
        n1458 = Multiply(x=w6095, y=u64 2) -> (x*y=w6094:dbl)
        "Data points/scan (f+b)" <- w6094
        n1459 = Multiply(x=w6094, y=w6085) -> (x*y=w6112:dbl)
        "Data points/scans (MCL)" <- w6112
        n1460 = Multiply(x=w6093, y=w6094) -> (x*y=w6086:dbl)
        "Time/f+b scan (s) (MCL)" <- w6086
        n1461 = Divide(x=w6112, y=w6092) -> (x/y=→"N sets should be saved (MCL)":dbl)
        n1462 = Multiply(x=w6086, y=w6085) -> (x*y=→"Total Time (s)":dbl)
        n1463 = Not(x="Fast Scan Dir") -> (.not. x?=w6090:bool)
        n1464 = xnode "Read/Write Control"("FPGA VI Reference In"=w6116, "error in"=w6115, "Scan steps (MCL)"="Scan steps (MCL)", "Number of scans (MCL)"=w6085, "Cycles per step (MCL)"=w6103, "Scan freq.  increment (MCL)"=w6083, "1D or 2D Scan?"="2D or 1D Scan", "MCL Scan Axis"=w6090, "Cont. Scan (MCL)"="Continuous MCL Scanning") -> ("error out"=w6114:errorcluster)  [unwired: 1 out]
      }
      event #34 {
        w6253 = 1000.0 ("y")
        n1465 = event-data() -> ()  [unwired: 7 out]
        n1466 = local read "Save file name"() -> (w6278:path)
        n1467 = local write "Read Cal"(FALSE ("Read Cal")) -> ()
        n1468 = Strip Path(path=w6278) -> (stripped path=w6277:path)  [unwired: 1 out]
        n1469 = Path To String(path=w6277) -> (string=w6276:string)
        n1470 = Concatenate Strings(w6276, "\\current.cal" ("string")) -> (w6274:string)
        n1471 = String To Path(string=w6274) -> (path=w6273:path)
        n1472 = Open/Create/Replace File(file path (use dialog)=w6273, operation (0:open)=T30."open", access (0:read/write)=enum16{"read/write", "read-only", "write-only"}."read-only") -> (refnum out=w6281:refnum<file>, error out=w6267:errorcluster)  [unwired: 1 in, 3 out]
        n1473 = Deny Access(4:w6267, 7:w6281) -> (0:w6266:errorcluster, 3:w6272:refnum<file>)  [unwired: 1 out]
        n1474 = Read from Binary File(5:0.0, 8:w6266, 9:T31."big-endian, network order" ("byte order (0:big-endian, network order)"), 10:-1 ("count (1)"), 11:w6272) -> (0:w6265:errorcluster, 2:w6263:dbl[], 3:w6268:refnum<file>)  [unwired: 2 out]
        n1475 = Array To Cluster(array=w6263) -> (cluster=w6262:T39)
        n1476 = Unbundle(w6262) -> ("[0]"=w6261:dbl, "[1]"=w6260:dbl, "[2]"=w6259:dbl, "[3]"=w6258:dbl, "[4]"=w6257:dbl, "[5]"=w6256:dbl)
        n1477 = Close File(refnum=w6268, error in=w6265) -> (error out=→"Read cal error":errorcluster)  [unwired: 1 out]
        n1478 = Multiply(x=w6256, y=w6253) -> (x*y=w6254:dbl)
        n1479 = local write "T2 kappa_x (pN/nm)"(w6258) -> ()
        n1480 = local write "T1 kappa_x (pN/nm)"(w6259) -> ()
        n1481 = local write "T1 alpha_x (nm/V)"(w6261) -> ()
        n1482 = local write "T2 alpha_x (nm/V)"(w6260) -> ()
        n1483 = Multiply(x=w6257, y=w6253) -> (x*y=w6255:dbl)
        n1484 = local write "T1 offset_x (mV)"(w6255) -> ()
        n1485 = local write "T2 offset_x (mV)"(w6254) -> ()
      }
      event #35 {
        n1486 = event-data() -> ()  [unwired: 7 out]
        n1487 = local write "MCL Scanning"(FALSE ("MCL Scanning")) -> ()
        n1488 = xnode "Read/Write Control"("FPGA VI Reference In"=w6286, "error in"=w6285, "Abort scan (MCL)"="Abort MCL Scan") -> ("error out"=w6284:errorcluster)  [unwired: 1 out]
      }
      event #36 {
        n1489 = event-data() -> ()  [unwired: 7 out]
        n1490 = xnode "Read/Write Control"("FPGA VI Reference In"=w6327, "error in"=w6326, "MCL count"="Update Count (MCL)") -> ("error out"=w6325:errorcluster)  [unwired: 1 out]
      }
      event #37 {
        n1491 = event-data() -> ()  [unwired: 7 out]
        n1492 = Negate(x="Phase adjust (MCL)") -> (-x=w6372:i16)
        n1493 = Select(t=w6372, s="- phase (MCL)", f="Phase adjust (MCL)") -> (s? t:f=w6370:i16)
        n1494 = Or(x="- phase (MCL)", y="+ phase (MCL)") -> (x .or. y?=w6365:bool)
        n1495 = xnode "Read/Write Control"("FPGA VI Reference In"=w6374, "error in"=w6373, "Phase count adjustment (MCL)"=w6370) -> ("FPGA VI Reference Out"=w6366:T15, "error out"=w6367:errorcluster)
        n1496 = xnode "Read/Write Control"("FPGA VI Reference In"=w6366, "error in"=w6367, "+ phase (MCL)"=w6365) -> ("error out"=w6364:errorcluster)  [unwired: 1 out]
      }
      event #38 {
        n1497 = event-data() -> ()  [unwired: 7 out]
        n1498 = xnode "Read/Write Control"("FPGA VI Reference In"=w6451, "error in"=w6450, "Abort scan"="Abort AOD Scan") -> ("error out"=w6449:errorcluster)  [unwired: 1 out]
      }
      event #39 {
        n1499 = event-data() -> ()  [unwired: 7 out]
        n1500 = xnode "Read/Write Control"("FPGA VI Reference In"=w6492, "error in"=w6491, "Cont. Scan"="Continuous AOD Scanning") -> ("error out"=w6490:errorcluster)  [unwired: 1 out]
      }
      event #40 {
        n1501 = event-data() -> ()  [unwired: 7 out]
        n1502 = call "Create new save file.vi"("Insert"="", "Ext"=".dat" ("string"), "Index In"="Index") -> ("Path Out"=→"Save file name":path, "Index Out"=w6530:dbl)
        "Save index" <- w6530
        n1503 = local write "Index"(w6530) -> ()
      }
      event #41 {
        w6545 = 10.0 ("y")
        w6544 = 32767.0 ("y")
        n1504 = event-data() -> ()  [unwired: 7 out]
        n1505 = local read "AO2"() -> (w6543:dbl)
        n1506 = local read "AO1"() -> (w6540:dbl)
        n1507 = Multiply(x=w6540, y=w6544) -> (x*y=w6539:dbl)
        n1508 = Multiply(x=w6543, y=w6544) -> (x*y=w6542:dbl)
        n1509 = Divide(x=w6539, y=w6545) -> (x/y=w6538:dbl)
        n1510 = Divide(x=w6542, y=w6545) -> (x/y=w6541:dbl)
        n1511 = To Word Integer(number=w6538) -> (16bit integer=w6546:i16)
        n1512 = To Word Integer(number=w6541) -> (16bit integer=w6547:i16)
        n1513 = xnode "Read/Write Control"("FPGA VI Reference In"=w6537, "error in"=w6536, "AO1"=w6546, "AO2"=w6547) -> ("error out"=w6535:errorcluster)  [unwired: 1 out]
      }
      event #42 {
        n1514 = event-data() -> ()  [unwired: 7 out]
        n1515 = local read "Syringe Pump Serial Port"() -> (w6603:refnum<visa-resource-name>)
        n1516 = local read "Pump write delay (ms)"() -> (w6604:dbl)
        n1517 = case shown="True" "Inject Top Channel" {
          tunnel: w6604 -> [w6609 w6617]
          tunnel: w6603 -> [w6606 w6616]
          frame #0 {
            n1518 = flat-sequence {
              tunnel: w6606 -> [w6610]
              tunnel: [w6610] -> w6607
              tunnel: w6609 -> [_]
              tunnel: [w6613] -> w6608
              tunnel: w6607 -> [w6613]
              tunnel: w6608 -> [w6614]
              frame #0 {
                n1519 = call "Write to pump.vi"("string"="enter pump1", "VISA resource name"=w6610) -> ()  [unwired: 1 out]
              }
              frame #1 {
                n1520 = Wait (ms)(milliseconds to wait="Pump pause delay (ms)") -> ()  [unwired: 1 out]
              }
              frame #2 {
                n1521 = call "Write to pump.vi"("string"="stop", "VISA resource name"=w6614) -> ()  [unwired: 1 out]
              }
            }
          }
          frame #1 {
            n1522 = flat-sequence {
              tunnel: w6616 -> [w6626]
              tunnel: w6617 -> [w6621]
              tunnel: w6617 -> [w6628]
              tunnel: w6616 -> [w6629]
              frame #0 {
                n1523 = local read "All Pump Parameters"() -> (w6620:T5)
                n1524 = Unbundle By Name(w6620) -> ("Pump 1"=w6627:T40)
                n1525 = call "Set pump parameters.vi"("Pump write delay (ms)"=w6621, "Volume (uL)"="Top Ch Inject Volume (uL)", "Rate (uL/h)"="Top Ch Inject Rate (ul/h)", "Units"=4.0, "Pump #"=1.0, "Pump Parameters In"=w6627, "VISA resource name"=w6626) -> ("Pump Parameters Out"=w6619:T40)  [unwired: 3 in]
                n1526 = Bundle By Name(cluster=w6620, "Pump 1"=w6619) -> (w6618:T5)
                n1527 = local write "All Pump Parameters"(w6618) -> ()
              }
              frame #1 {
                n1528 = Wait (ms)(milliseconds to wait=w6628) -> ()  [unwired: 1 out]
              }
              frame #2 {
                n1529 = call "Write to pump.vi"("string"="start", "VISA resource name"=w6629) -> ()  [unwired: 1 out]
              }
            }
          }
        }
      }
      event #43 {
        n1530 = event-data() -> ()  [unwired: 7 out]
        n1531 = local read "Pump write delay (ms)"() -> (w6632:dbl)
        n1532 = case shown="False" "Inject Bottom Channel" {
          tunnel: w6632 -> [w6637 w6645]
          tunnel: "Syringe Pump Serial Port" -> [w6634 w6644]
          frame #0 {
            n1533 = flat-sequence {
              tunnel: w6634 -> [w6638]
              tunnel: [w6638] -> w6635
              tunnel: w6637 -> [_]
              tunnel: [w6641] -> w6636
              tunnel: w6635 -> [w6641]
              tunnel: w6636 -> [w6642]
              frame #0 {
                n1534 = call "Write to pump.vi"("string"="enter pump3", "VISA resource name"=w6638) -> ()  [unwired: 1 out]
              }
              frame #1 {
                n1535 = local read "Pump pause delay (ms)"() -> (w6640:u32)
                n1536 = Wait (ms)(milliseconds to wait=w6640) -> ()  [unwired: 1 out]
              }
              frame #2 {
                n1537 = call "Write to pump.vi"("string"="stop", "VISA resource name"=w6642) -> ()  [unwired: 1 out]
              }
            }
          }
          frame #1 {
            n1538 = flat-sequence {
              tunnel: w6644 -> [w6654]
              tunnel: w6645 -> [w6649]
              tunnel: w6645 -> [w6656]
              tunnel: w6644 -> [w6657]
              frame #0 {
                n1539 = local read "All Pump Parameters"() -> (w6648:T5)
                n1540 = Unbundle By Name(w6648) -> ("Pump 3"=w6655:T40)
                n1541 = call "Set pump parameters.vi"("Pump write delay (ms)"=w6649, "Volume (uL)"="Bottom Ch Inject Volume (uL)", "Rate (uL/h)"="Bottom Ch Inject Rate (ul/h)", "Units"=4.0, "Pump #"=3.0, "Pump Parameters In"=w6655, "VISA resource name"=w6654) -> ("Pump Parameters Out"=w6647:T40)  [unwired: 3 in]
                n1542 = Bundle By Name(cluster=w6648, "Pump 3"=w6647) -> (w6646:T5)
                n1543 = local write "All Pump Parameters"(w6646) -> ()
              }
              frame #1 {
                n1544 = Wait (ms)(milliseconds to wait=w6656) -> ()  [unwired: 1 out]
              }
              frame #2 {
                n1545 = call "Write to pump.vi"("string"="start", "VISA resource name"=w6657) -> ()  [unwired: 1 out]
              }
            }
          }
        }
      }
      event #44 {
        n1546 = event-data() -> ()  [unwired: 7 out]
        n1547 = local read "Pump write delay (ms)"() -> (w6661:dbl)
        n1548 = flat-sequence {
          tunnel: w6659 -> [w6674]
          tunnel: w6661 -> [w6670]
          tunnel: "Flush Center Channel" -> [_]
          tunnel: w6661 -> [w6676]
          tunnel: w6659 -> [w6677]
          frame #0 {
            n1549 = local read "All Pump Parameters"() -> (w6669:T5)
            n1550 = Multiply(x=60.0, y="Flush Center Ch Rate (ul/m)") -> (x*y=w6666:dbl)
            n1551 = Unbundle By Name(w6669) -> ("Pump 2"=w6675:T40)
            n1552 = call "Set pump parameters.vi"("Pump write delay (ms)"=w6670, "Volume (uL)"="Flush Center Ch Volume (uL)", "Rate (uL/h)"=w6666, "Units"=3.0, "Pump #"=2.0, "Pump Parameters In"=w6675, "VISA resource name"=w6674) -> ("Pump Parameters Out"=w6668:T40)  [unwired: 3 in]
            n1553 = Bundle By Name(cluster=w6669, "Pump 2"=w6668) -> (w6667:T5)
            n1554 = Add(x="Flush Center Ch Volume (uL)", y="Total Volume\nFlushed (uL)") -> (x+y=w6663:dbl)
            n1555 = local write "All Pump Parameters"(w6667) -> ()
            n1556 = local write "Total Volume\nFlushed (uL)"(w6663) -> ()
          }
          frame #1 {
            n1557 = Wait (ms)(milliseconds to wait=w6676) -> ()  [unwired: 1 out]
          }
          frame #2 {
            n1558 = call "Write to pump.vi"("string"="start", "VISA resource name"=w6677) -> ()  [unwired: 1 out]
          }
        }
        n1559 = local read "Syringe Pump Serial Port"() -> (w6659:refnum<visa-resource-name>)
      }
    }
    "error out 2" <- w3948
    n1560 = node-c288() -> ()  [unwired: 2 out]
  }
  n1561 = timed-loop "Rough control of MCL mirror stage (debugging)" {
    tunnel: w76 -> [w6681]
    tunnel: [w6680] -> w182
    timing: w7 -> [_]
    timing-out: [_] -> w6
    stop <- w6680 stop-if-true
    n1562 = node-c288() -> ()  [unwired: 2 out]
    n1563 = case shown="1" "MCL Mode" {
      tunnel: w6681 -> [_ w6684 w6786]
      frame #0 {
      }
      frame #1 {
        n1564 = node-c288() -> (w6686:T18)  [unwired: 4 out]
        n1565 = timed-loop "Oscillate MCL mirror" {
          timing: w6686 -> [_]
          timing-out: [_] -> w6685
          tunnel: w6684 -> [w6725]
          i -> [w6724]
          stop <- w6687 stop-if-true
          n1566 = node-c288() -> (w6723:i64)  [unwired: 1 out]
          n1567 = Multiply(x="AO1", y=32767.0) -> (x*y=w6719:dbl)
          n1568 = Multiply(x="AO2", y=32767.0) -> (x*y=w6714:dbl)
          n1569 = Divide(x=w6719, y=10.0) -> (x/y=w6720:dbl)
          n1570 = Divide(x=w6714, y=10.0) -> (x/y=w6715:dbl)
          n1571 = To Word Integer(number=w6720) -> (16bit integer=w6712:i16)
          n1572 = To Word Integer(number=w6715) -> (16bit integer=w6711:i16)
          n1573 = Divide(x=w6723, y=i64 1000) -> (x/y=w6694:dbl)
          n1574 = Multiply(x=w6694, y=w6724) -> (x*y=w6705:dbl)
          n1575 = Multiply(x="Osc. freq. (Hz) 2", y=6.283185307179586) -> (x*y=w6706:dbl)
          n1576 = Multiply(x=w6706, y=w6705) -> (x*y=w6704:dbl)
          n1577 = Sine(x=w6704) -> (sin(x)=w6703:dbl)
          n1578 = Multiply(x=w6703, y="Osc. amp. (V)") -> (x*y=w6701:dbl)
          n1579 = Add(x=w6701, y="Osc. center (V)") -> (x+y=w6699:dbl)
          n1580 = Divide(x=w6699, y=10.0) -> (x/y=w6697:dbl)
          n1581 = Multiply(x=w6697, y=32767.0) -> (x*y=w6692:dbl)
          n1582 = Select(t=w6692, s="Scan axis", f=w6712) -> (s? t:f=w6710:dbl)
          n1583 = Select(t=w6711, s="Scan axis", f=w6692) -> (s? t:f=w6709:dbl)
          n1584 = local read "MCL Mode"() -> (w6691:u16)
          n1585 = Not Equal?(x=w6691, y=u16 1) -> (x != y?=w6688:bool)
          n1586 = local read "Stop All"() -> (w6689:bool)
          n1587 = xnode "Read/Write Control"("FPGA VI Reference In"=w6725, "AO1"=w6710, "AO2"=w6709) -> ()  [unwired: 1 in, 2 out]
          n1588 = Compound Arithmetic op=OR(w6689, w6688) -> (w6687:bool)
          n1589 = node-c288() -> ()  [unwired: 2 out]
        }
        n1590 = node-c288(w6685) -> ()  [unwired: 1 out]
      }
      frame #2 {
        n1591 = case shown="True" "Start Scan" {
          tunnel: w6786 -> [_ w6798]
          frame #0 {
          }
          frame #1 {
            n1592 = Subtract(x="End (V)", y="Begin (V)") -> (x-y=w6794:dbl)
            n1593 = Decrement(x="N Points") -> (x-1=w6793:dbl)
            n1594 = Divide(x=w6794, y=w6793) -> (x/y=w6791:dbl)
            n1595 = for {
              N: "N Points" -> [_]
              tunnel: "Begin (V)" -> [w6811]
              tunnel: w6798 -> [w6803]
              tunnel: [w6802] -> w6797 mode=indexing
              tunnel: w6791 -> [w6801]
              tunnel: [w6799] -> w6790 mode=indexing
              i -> [w6810]
              n1596 = Multiply(x=w6801, y=w6810) -> (x*y=w6809:dbl)
              n1597 = Add(x=w6811, y=w6809) -> (x+y=w6806:dbl)
              n1598 = local read "Scan axis"() -> (w6800:bool)
              n1599 = local read "AO1"() -> (w6808:dbl)
              n1600 = local read "AO2"() -> (w6807:dbl)
              n1601 = Select(t=w6806, s=w6800, f=w6808) -> (s? t:f=w6805:dbl)
              n1602 = Select(t=w6807, s=w6800, f=w6806) -> (s? t:f=w6804:dbl)
              n1603 = flat-sequence {
                tunnel: w6805 -> [w6815]
                tunnel: w6804 -> [w6814]
                tunnel: w6803 -> [w6812]
                tunnel: [w6880] -> w6802
                tunnel: [w6879] -> w6799
                frame #0 {
                  w6818 = 10.0 ("y")
                  w6813 = 32767.0 ("y")
                  n1604 = Multiply(x=w6815, y=w6813) -> (x*y=w6821:dbl)
                  n1605 = Multiply(x=w6814, y=w6813) -> (x*y=w6819:dbl)
                  n1606 = Divide(x=w6821, y=w6818) -> (x/y=w6822:dbl)
                  n1607 = Divide(x=w6819, y=w6818) -> (x/y=w6820:dbl)
                  n1608 = To Word Integer(number=w6822) -> (16bit integer=w6816:i16)
                  n1609 = To Word Integer(number=w6820) -> (16bit integer=w6817:i16)
                  n1610 = xnode "Read/Write Control"("FPGA VI Reference In"=w6812, "AO1"=w6816, "AO2"=w6817) -> ()  [unwired: 1 in, 2 out]
                }
                frame #1 {
                  n1611 = Wait (ms)(milliseconds to wait="DAQ Delay (ms)") -> ()  [unwired: 1 out]
                }
                frame #2 {
                  n1612 = local read "Slow mean"() -> (w6880:dbl)
                  n1613 = local read "Sigma"() -> (w6879:dbl)
                }
              }
            }
            n1614 = Bundle("Begin (V)"="Begin (V)", w6791, w6797) -> (→"MCL Scan":cluster{"Begin (V)":dbl, dbl, dbl[]})  [unwired: 1 out]
            n1615 = Bundle("Begin (V)"="Begin (V)", w6791, w6790) -> (→"MCL Scan 2":cluster{"Begin (V)":dbl, dbl, dbl[]})  [unwired: 1 out]
          }
        }
      }
    }
    n1616 = local read "Stop All"() -> (w6680:bool)
    n1617 = node-c288() -> ()  [unwired: 2 out]
  }
  n1618 = timed-loop "Mouse control: trap position (AOM deflection), set confocal spot from image" {
    tunnel: [w6882] -> w133
    tunnel: w76 -> [w6881]
    timing: w15 -> [_]
    timing-out: [_] -> w14
    stop <- w6882 stop-if-true
    n1619 = node-c288() -> ()  [unwired: 2 out]
    n1620 = event shown="[0] \"Pane\": Mouse Down" {
      selector: _ -> [_ _]
      dyn-events: _ -> [_ _]
      timeout: _ -> [_ _]
      tunnel: w6881 -> [w6885 _]
      event #0 {
        n1621 = event-data() -> ("Time"=w6887:u32, "Coords"=w6886:T7, "Button"=w6888:u16)  [unwired: 6 out]
        n1622 = case shown="1" w6888 {
          tunnel: w6887 -> [_ _ w6946]
          tunnel: w6886 -> [_ w6908 w6944]
          tunnel: w6885 -> [_ _ w6942]
          frame #0 {
          }
          frame #1 {
            n1623 = property on="APD 1b" class="ImageControl"() -> ("Displayed Image Position"=w6907:cluster{"Left":i32, "Top":i32})  [unwired: 2 in, 2 out]
            n1624 = property on="APD 1b" class="ImageControl"() -> ("Displayed Image Size"=w6906:cluster{"Width":u32, "Height":u32})  [unwired: 2 in, 2 out]
            n1625 = Unbundle By Name(w6908) -> ("Horizontal"=w6905:i32, "Vertical"=w6902:i32)
            n1626 = Unbundle By Name(w6906) -> ("Width"=w6898:u32, "Height"=w6899:u32)
            n1627 = Unbundle By Name(w6907) -> ("Left"=w6904:i32, "Top"=w6903:i32)
            n1628 = To Long Integer(number=w6898) -> (32bit integer=w6893:i32)
            n1629 = To Long Integer(number=w6899) -> (32bit integer=w6892:i32)
            n1630 = Subtract(x=w6905, y=w6904) -> (x-y=w6897:i32)
            n1631 = Add(x=w6903, y=w6892) -> (x+y=w6901:i32)
            n1632 = Subtract(x=w6902, y=w6901) -> (x-y=w6900:i32)
            n1633 = Negate(x=w6900) -> (-x=w6896:i32)
            n1634 = In Range and Coerce(upper limit=w6893, x=w6897, lower limit=0) -> (In Range?=w6891:bool)  [unwired: 1 out]
            n1635 = In Range and Coerce(upper limit=w6892, x=w6896, lower limit=0) -> (In Range?=w6890:bool)  [unwired: 1 out]
            n1636 = And(x=w6891, y=w6890) -> (x .and. y?=w6889:bool)
            n1637 = case shown="True" w6889 {
              tunnel: w6897 -> [_ w6916]
              tunnel: w6896 -> [_ w6915]
              tunnel: w6893 -> [_ w6914]
              tunnel: w6892 -> [_ w6913]
              frame #0 {
              }
              frame #1 {
                n1638 = local read "Scan lines (y)"() -> (w6918:u64)
                n1639 = local read "Actual MCL Inc (V)"() -> (w6909:dbl)
                n1640 = local read "Scan steps (MCL)"() -> (w6917:u64)
                n1641 = Divide "Y Pix/step"(x=w6913, y=w6918) -> (x/y=w6925:dbl)
                n1642 = Divide "Y V/pix"(x=w6909, y=w6925) -> (x/y=w6924:dbl)
                n1643 = Divide "Y half step offset"(x=w6909, y=2.0) -> (x/y=w6926:dbl)
                n1644 = Divide "X pix/step"(x=w6914, y=w6917) -> (x/y=w6923:dbl)
                n1645 = Negate(x=w6926) -> (-x=w6927:dbl)
                n1646 = local read "Initial Y"() -> (w6933:dbl)
                n1647 = Multiply(x=w6915, y=w6924) -> (x*y=w6934:dbl)
                n1648 = Divide "X half step offset"(x=w6909, y=2.0) -> (x/y=w6920:dbl)
                n1649 = Divide "X V/pix"(x=w6909, y=w6923) -> (x/y=w6922:dbl)
                n1650 = Multiply(x=w6909, y=w6917) -> (x*y=w6929:dbl)
                n1651 = Compound Arithmetic op=ADD(w6927, w6934, w6933) -> (w6910:dbl)
                "Y (V)" <- w6910
                n1652 = Multiply(x=w6922, y=w6916) -> (x*y=w6931:dbl)
                n1653 = Negate(x=w6920) -> (-x=w6919:dbl)
                n1654 = local read "Initial X"() -> (w6932:dbl)
                n1655 = Negate(x=w6931) -> (-x=w6930:dbl)
                n1656 = Compound Arithmetic op=ADD(w6919, w6929, w6932, w6930) -> (w6911:dbl)
                "X (V)" <- w6911
                n1657 = case shown="True" "Set Confocal Spot" {
                  tunnel: w6911 -> [_ w6936]
                  tunnel: w6910 -> [_ w6935]
                  frame #0 {
                  }
                  frame #1 {
                    n1658 = flat-sequence {
                      tunnel: w6936 -> [w6938]
                      tunnel: w6935 -> [w6939]
                      frame #0 {
                        n1659 = local write "AO2"(w6938) -> ()
                      }
                      frame #1 {
                        n1660 = property on="AO1" class="Slide (strict)"("Val(Sgnl)"=w6939) -> ()  [unwired: 2 in, 2 out]
                      }
                    }
                    n1661 = local write "Set Confocal Spot"(FALSE ("Get Point")) -> ()
                  }
                }
              }
            }
          }
          frame #2 {
            n1662 = local read "BD 2 Frequency 1 (MHz)"() -> (w6940:dbl)
            n1663 = local read "BD 1 Frequency 1 (MHz)"() -> (w6941:dbl)
            n1664 = local write "Manipulating Trap"(TRUE ("Manipulating Trap")) -> ()
            n1665 = local write "Coords"(T7 {"Horizontal"=0, "Vertical"=0} ("Coords")) -> ()
            n1666 = while {
              tunnel: w6946 -> [w6951]
              tunnel: w6944 -> [w6950]
              tunnel: w6942 -> [w6949]
              tunnel: w6941 -> [w6948]
              tunnel: w6940 -> [w6947]
              stop <- w6952 stop-if-true
              n1667 = event shown="[0] \"Pane\": Mouse Move" {
                selector: _ -> [_ _]
                dyn-events: _ -> [_ _]
                timeout: _ -> [_ _]
                tunnel: ["Force Manip Abort" w7016] -> w6952
                tunnel: w6951 -> [w6959 _]
                tunnel: w6950 -> [w6957 _]
                tunnel: w6949 -> [w6956 _]
                tunnel: w6948 -> [w6955 _]
                tunnel: w6947 -> [w6954 _]
                event #0 {
                  n1668 = event-data() -> ("Time"=w6960:u32, "Coords"=w6961:T7)  [unwired: 3 out]
                  n1669 = Less?(x=w6960, y=w6959) -> (x < y?=w6958:bool)
                  n1670 = case "Makes sure old motion events prior to mouse click aren't used" shown="False" w6958 {
                    tunnel: w6961 -> [w7003 _]
                    tunnel: w6957 -> [w7004 _]
                    tunnel: w6956 -> [w6981 _]
                    tunnel: w6955 -> [w6977 _]
                    tunnel: w6954 -> [w6976 _]
                    frame #0 {
                      n1671 = Subtract(x=w7003, y=w7004) -> (x-y=w7002:T7)
                      "Coords" <- w7002
                      n1672 = local read "Y RF Frequency Limits (MHz)"() -> (w6962:T12)
                      n1673 = To Double Precision Float(number=w7002) -> (double precision float=w7001:cluster{"Horizontal":dbl, "Vertical":dbl})
                      n1674 = Multiply(x=cluster{"Horizontal":dbl, "Vertical":dbl} {"Horizontal"=-1.0, "Vertical"=1.0}, y="Manipulation Scaling") -> (x*y=w6997:cluster{"Horizontal":dbl, "Vertical":dbl})
                      n1675 = Multiply(x=w7001, y=w6997) -> (x*y=w6999:cluster{"Horizontal":dbl, "Vertical":dbl})
                      n1676 = local read "X RF Frequency Limits (MHz)"() -> (w6963:T12)
                      n1677 = Unbundle By Name(w6999) -> ("Horizontal"=w6994:dbl, "Vertical"=w6998:dbl)
                      n1678 = Boolean To (0,1)(Boolean="Manip. X?") -> (0, 1=w6992:i16)
                      n1679 = Unbundle By Name(w6962) -> ("Maximum"=w6965:dbl, "Minimum"=w6964:dbl)
                      n1680 = Boolean To (0,1)(Boolean="Manip. Y?") -> (0, 1=w6989:i16)
                      n1681 = Multiply(x=w6998, y=w6989) -> (x*y=w6991:dbl)
                      n1682 = Multiply(x=w6992, y=w6994) -> (x*y=w6995:dbl)
                      n1683 = local read "BD 1 Frequency 2 (MHz)"() -> (w6979:dbl)
                      n1684 = Unbundle By Name(w6963) -> ("Maximum"=w6967:dbl, "Minimum"=w6966:dbl)
                      n1685 = local read "BD 2 Frequency 2 (MHz)"() -> (w6978:dbl)
                      n1686 = Add(x=w6976, y=w6991) -> (x+y=w6969:dbl)
                      n1687 = Add(x=w6977, y=w6995) -> (x+y=w6971:dbl)
                      n1688 = In Range and Coerce(upper limit=w6967, x=w6971, lower limit=w6966) -> (coerced(x)=w6970:dbl)  [unwired: 1 out]
                      n1689 = In Range and Coerce(upper limit=w6965, x=w6969, lower limit=w6964) -> (coerced(x)=w6968:dbl)  [unwired: 1 out]
                      n1690 = Subtract(x=w6970, y=w6979) -> (x-y=w6988:dbl)
                      n1691 = Subtract(x=w6968, y=w6978) -> (x-y=w6987:dbl)
                      n1692 = Square(x=w6988) -> (x^2=w6986:dbl)
                      n1693 = Square(x=w6987) -> (x^2=w6985:dbl)
                      n1694 = Add(x=w6986, y=w6985) -> (x+y=w6984:dbl)
                      n1695 = Square Root(x=w6984) -> (sqrt(x)=w6980:dbl)
                      n1696 = In Range and Coerce(upper limit="Limit Max (MHz)", x=w6980, lower limit="Limit Min (MHz)") -> (In Range?=w6973:bool)  [unwired: 1 out]
                      n1697 = Not(x="Limits Enable") -> (.not. x?=w6972:bool)
                      n1698 = Or(x=w6973, y=w6972) -> (x .or. y?=w6974:bool)
                      n1699 = case shown="True" w6974 {
                        tunnel: w6981 -> [_ w7014]
                        tunnel: w6980 -> [_ w7005]
                        tunnel: w6970 -> [_ w7012]
                        tunnel: w6979 -> [_ w7011]
                        tunnel: w6968 -> [_ w7010]
                        tunnel: w6978 -> [_ w7009]
                        tunnel: w6963 -> [_ w7007]
                        tunnel: w6962 -> [_ w7006]
                        frame #0 {
                        }
                        frame #1 {
                          n1700 = local read "BD 1 Frequency 3 (MHz)"() -> (w7013:dbl)
                          n1701 = local read "BD 2 Frequency 3 (MHz)"() -> (w7008:dbl)
                          n1702 = local write "Trap Delta (MHz)"(w7005) -> ()
                          n1703 = property on="Initial delta (MHz)" class="DigNum (strict)"("Val(Sgnl)"=w7005) -> ()  [unwired: 2 in, 2 out]
                          n1704 = call "set RF board frequency - interlace.vi"("Board 2 Frequency Limits"=w7006, "Board 1 Frequency Limits"=w7007, "FPGA VI Reference In"=w7014, "Board 2 Frequency 3 (MHz)"=w7008, "Board 1 Frequency 3 (MHz)"=w7013, "Board 2 Frequency 2 (MHz)"=w7009, "Board 2 Frequency 1 (MHz)"=w7010, "Board 1 Frequency 2 (MHz)"=w7011, "Board 1 Frequency 1  (MHz)"=w7012) -> ()  [unwired: 1 in, 2 out]
                          n1705 = local write "BD 2 Frequency 1 (MHz)"(w7010) -> ()
                          n1706 = local write "BD 1 Frequency 1 (MHz)"(w7012) -> ()
                        }
                      }
                    }
                    frame #1 {
                    }
                  }
                }
                event #1 {
                  n1707 = event-data() -> ("Button"=w7015:u16)  [unwired: 8 out]
                  n1708 = case shown="3" w7015 {
                    tunnel: [FALSE TRUE] -> w7016
                    frame #0 {
                    }
                    frame #1 {
                      n1709 = local write "Manipulating Trap"(FALSE ("Manipulating Trap")) -> ()
                    }
                  }
                }
              }
            }
          }
        }
      }
      event #1 {
        n1710 = event-data() -> ()  [unwired: 6 out]
      }
    }
    n1711 = local read "Stop All"() -> (w6882:bool)
    n1712 = node-c288() -> ()  [unwired: 2 out]
  }
  n1713 = timed-loop "Stage Control and Stage + Action Control" {
    shift-right: [w7031] -> w57
    shift-left: w59 -> [w7048]
    shift-right: [w7030] -> w56
    shift-left: w58 -> [w7047]
    tunnel: w55 -> [w7032]
    timing: w13 -> [_]
    timing-out: [_] -> w12
    shift-right: ["Dump Beads"] -> _
    shift-left: FALSE ("Dump Beads") -> [w7023]
    stop <- w7049 stop-if-true
    (unwired) T12 {"Minimum"=0.0, "Maximum"=0.0, "Increment"=0.0}  # Y Limits
    (unwired) T12 {"Minimum"=0.0, "Maximum"=0.0, "Increment"=0.0}  # X Limits
    n1714 = node-c288() -> ()  [unwired: 2 out]
    n1715 = local read "Stop All"() -> (w7049:bool)
    n1716 = call "Read Stage Position.vi"("error in"=w7047, "VISA resource name in"=w7048) -> ("Current Position"=w7033:cluster{dbl, dbl, dbl}, "error out"=w7040:errorcluster, "VISA resource name out"=w7041:refnum<visa-resource-name>)  [unwired: 1 out]
    "Current Stage  Position" <- w7033
    n1717 = Or(x="Move to Position 3", y="Data Acq. Spot") -> (x .or. y?=w7026:bool)
    n1718 = Or(x="Lower Cap.", y=w7023) -> (x .or. y?=w7022:bool)
    n1719 = Or(x="Move to Position 1", y="Upper Cap.") -> (x .or. y?=w7029:bool)
    n1720 = Compound Arithmetic op=OR(w7022, "Move to Position 2") -> (w7028:bool)
    n1721 = Or(x="Dump Beads", y="Move to Position 4") -> (x .or. y?=w7025:bool)
    n1722 = Build Array(w7029, w7028, w7026, w7025) -> (w7039:bool[])
    n1723 = Or Array Elements(Boolean array=w7039) -> (logical OR=w7042:bool)
    n1724 = case shown="True" w7042 {
      tunnel: w7041 -> [w7094 w7102]
      tunnel: w7040 -> [w7093 w7101]
      tunnel: [w7094 w7105] -> w7038
      tunnel: [w7093 w7104] -> w7037
      tunnel: w7039 -> [_ w7103]
      tunnel: "Dump Beads" -> [_ w7098]
      tunnel: w7022 -> [_ w7097]
      tunnel: "Upper Cap." -> [_ w7096]
      tunnel: "Data Acq. Spot" -> [_ w7095]
      frame #0 {
      }
      frame #1 {
        n1725 = flat-sequence {
          tunnel: w7103 -> [w7113]
          tunnel: w7102 -> [w7108]
          tunnel: w7101 -> [w7107]
          tunnel: [w7116] -> w7100
          tunnel: [w7115] -> w7099
          tunnel: [w7122] -> w7104
          tunnel: [w7123] -> w7105
          tunnel: w7100 -> [w7123]
          tunnel: w7099 -> [w7122]
          tunnel: w7098 -> [w7120]
          tunnel: w7097 -> [w7119]
          tunnel: w7096 -> [w7118]
          tunnel: w7095 -> [w7117]
          frame #0 {
            n1726 = Boolean Array To Number(Boolean array=w7113) -> (number=w7114:u32)
            n1727 = local read "Saved Stage Positions"() -> (w7112:T4)
            n1728 = Logarithm Base 2(1:w7114) -> (0:w7110:dbl)
            n1729 = Cluster To Array(cluster=w7112) -> (array=w7111:cluster{dbl, dbl, dbl}[])
            n1730 = Index Array(array=w7111, index=w7110) -> (element=w7109:cluster{dbl, dbl, dbl})
            n1731 = call "Set Stage Position.vi"("Position"=w7109, "error in"=w7107, "VISA resource name in"=w7108) -> ("error out"=w7115:errorcluster, "VISA resource name out"=w7116:refnum<visa-resource-name>)  [unwired: 1 out]
            "Stage Moving" <- TRUE ("Stage Moving")
          }
          frame #1 {
            n1732 = local write "Stage Moving"(FALSE ("Stage Moving")) -> ()
            n1733 = case shown="True" w7120 {
              frame #0 {
              }
              frame #1 {
                w7138 = FALSE ("Value (Signaling)")
                n1734 = property on="Green Laser ON/Interlacing" class="Bool (strict)"("Val(Sgnl)"=w7138) -> ()  [unwired: 2 in, 2 out]
                n1735 = property on="Trap 1 (ON/OFF)" class="Bool (strict)"("Val(Sgnl)"=w7138) -> ()  [unwired: 2 in, 2 out]
                n1736 = property on="Trap 2 (ON/OFF)" class="Bool (strict)"("Val(Sgnl)"=w7138) -> ()  [unwired: 2 in, 2 out]
              }
            }
            n1737 = call <vilib>:"Beep.vi"() -> ()  [unwired: 3 in, 9 out]
            n1738 = case shown="True" w7118 {
              selector: w7118 -> [_ w7136]
              frame #0 {
              }
              frame #1 {
                n1739 = property on="Trap 2 (ON/OFF)" class="Bool (strict)"("Val(Sgnl)"=w7136) -> ()  [unwired: 2 in, 2 out]
              }
            }
            n1740 = case shown="True" w7117 {
              selector: w7117 -> [_ w7124]
              frame #0 {
              }
              frame #1 {
                n1741 = flat-sequence {
                  tunnel: w7124 -> [w7125]
                  frame #0 {
                    n1742 = property on="Save Calibration" class="Bool (strict)"("Val(Sgnl)"=w7125) -> ()  [unwired: 2 in, 2 out]
                  }
                  frame #1 {
                    n1743 = Wait (ms)(milliseconds to wait=u32 2000) -> ()  [unwired: 1 out]
                  }
                  frame #2 {
                    n1744 = while {
                      stop <- w7127 stop-if-true
                      n1745 = local read "Saving..."() -> (w7128:bool)
                      n1746 = Wait (ms)(milliseconds to wait=u32 1000) -> ()  [unwired: 1 out]
                      n1747 = Not(x=w7128) -> (.not. x?=w7127:bool)
                    }
                  }
                  frame #3 {
                    n1748 = Multiply(x="Cal read wait (s)", y=u32 1000 ("milliseconds to wait")) -> (x*y=w7131:u32)
                    n1749 = Wait (ms)(milliseconds to wait=w7131) -> ()  [unwired: 1 out]
                  }
                  frame #4 {
                    n1750 = property on="Read Cal" class="Bool (strict)"("Val(Sgnl)"=TRUE ("Value (Signaling)")) -> ()  [unwired: 2 in, 2 out]
                  }
                  frame #5 {
                    n1751 = Wait (ms)(milliseconds to wait=u32 2000) -> ()  [unwired: 1 out]
                  }
                  frame #6 {
                    n1752 = property on="Fish for Tether" class="Bool (strict)"("Val(Sgnl)"=TRUE ("Value (Signaling)")) -> ()  [unwired: 2 in, 2 out]
                  }
                }
              }
            }
            n1753 = case shown="True" w7119 {
              selector: w7119 -> [_ w7137]
              frame #0 {
              }
              frame #1 {
                n1754 = property on="Trap 1 (ON/OFF)" class="Bool (strict)"("Val(Sgnl)"=w7137) -> ()  [unwired: 2 in, 2 out]
              }
            }
          }
        }
      }
    }
    n1755 = Or(x="+z", y="-z") -> (x .or. y?=w7036:bool)
    n1756 = case shown="True" w7036 {
      tunnel: w7038 -> [w7053 w7057]
      tunnel: w7037 -> [w7052 w7056]
      tunnel: [w7053 w7060] -> w7031
      tunnel: [w7052 w7059] -> w7030
      tunnel: "+z" -> [_ w7063]
      tunnel: "-z" -> [_ w7062]
      tunnel: w7033 -> [_ w7061]
      tunnel: w7032 -> [_ w7058]
      frame #0 {
      }
      frame #1 {
        n1757 = flat-sequence {
          tunnel: w7063 -> [w7089]
          tunnel: w7062 -> [w7088]
          tunnel: w7061 -> [w7084]
          tunnel: w7058 -> [w7069]
          tunnel: w7057 -> [w7066]
          tunnel: w7056 -> [w7065]
          tunnel: [w7076] -> w7055
          tunnel: [w7075] -> w7054
          tunnel: [w7091] -> w7059
          tunnel: [w7092] -> w7060
          tunnel: w7055 -> [w7092]
          tunnel: w7054 -> [w7091]
          frame #0 {
            n1758 = Boolean To (0,1)(Boolean=w7089) -> (0, 1=w7087:i16)
            n1759 = Boolean To (0,1)(Boolean=w7088) -> (0, 1=w7086:i16)
            n1760 = Unbundle(w7084) -> (w7083:dbl, w7082:dbl, w7078:dbl)
            n1761 = Divide(x="z nudge increment (um)", y=1000.0) -> (x/y=w7072:dbl)
            n1762 = Multiply(x=w7087, y=w7072) -> (x*y=w7080:dbl)
            n1763 = Multiply(x=w7086, y=w7072) -> (x*y=w7085:dbl)
            n1764 = Negate(x=w7085) -> (-x=w7081:dbl)
            n1765 = Add(x=w7080, y=w7081) -> (x+y=w7079:dbl)
            n1766 = local write "Stage Moving"(TRUE ("Stage Moving")) -> ()
            n1767 = Add(x=w7079, y=w7078) -> (x+y=w7071:dbl)
            n1768 = Unbundle(w7069) -> ("Minimum"=w7068:dbl, "Maximum"=w7067:dbl)  [unwired: 1 out]
            n1769 = In Range and Coerce(upper limit=w7067, x=w7071, lower limit=w7068) -> (coerced(x)=w7070:dbl)  [unwired: 1 out]
            n1770 = Bundle(cluster=w7084, w7083, w7082, w7070) -> (w7077:cluster{dbl, dbl, dbl})
            n1771 = call "Set Stage Position.vi"("Position"=w7077, "error in"=w7065, "VISA resource name in"=w7066) -> ("error out"=w7075:errorcluster, "VISA resource name out"=w7076:refnum<visa-resource-name>)  [unwired: 1 out]
          }
          frame #1 {
            n1772 = local write "Stage Moving"(FALSE ("Stage Moving")) -> ()
          }
        }
      }
    }
    n1773 = node-c288() -> ()  [unwired: 2 out]
  }
  n1774 = for "Create Greyscale map" {
    N: 256 -> [_]
    tunnel: [w7140] -> w186 mode=indexing
    i -> [w7143]
    n1775 = To Unsigned Byte Integer(number=w7143) -> (unsigned 8bit integer=w7139:u8)
    n1776 = Join Numbers(hi=w7139, lo=w7139) -> ((hi.lo)=w7142:u16)
    n1777 = Join Numbers(hi=w7139, lo=w7139) -> ((hi.lo)=w7141:u16)
    n1778 = Join Numbers(hi=w7142, lo=w7141) -> ((hi.lo)=w7140:u32)
  }
  n1779 = node-c288(w6) -> ()  [unwired: 1 out]
  n1780 = node-c288(w10) -> ()  [unwired: 1 out]
  n1781 = node-c288(w14) -> ()  [unwired: 1 out]
  n1782 = node-c288(w12) -> ()  [unwired: 1 out]
  n1783 = VISA Close(VISA resource name=w57, error in (no error)=w56) -> (error out=w61:errorcluster)
  n1784 = node-c288(w8) -> ()  [unwired: 1 out]
  n1785 = call <vilib>:"Simple Error Handler.vi"("error in (no error)"=w61) -> ()  [unwired: 1 in, 8 out]
  n1786 = node-c288(w125) -> ()  [unwired: 1 out]
  n1787 = flat-sequence {
    tunnel: w227 -> [w7147]
    tunnel: w229 -> [w7148]
    tunnel: [w7146] -> w207
    tunnel: [w7145] -> w206
    tunnel: w182 -> [_]
    tunnel: w180 -> [_]
    tunnel: w133 -> [_]
    tunnel: w16 -> [_]
    tunnel: w207 -> [w7206]
    tunnel: w206 -> [w7207]
    frame #0 {
      w7144 = FALSE ("AI to FIFO")
      n1788 = xnode "Read/Write Control"("FPGA VI Reference In"=w7148, "error in"=w7147, "AI to FIFO"=w7144, "APD to FIFO"=w7144) -> ("FPGA VI Reference Out"=w7146:T15, "error out"=w7145:errorcluster)
    }
    frame #1 {
      n1789 = xnode "Close FPGA VI Reference"("FPGA VI Reference In"=w7206, "error in"=w7207) -> ("error out"=→"error out":errorcluster)
    }
  }
